vi "Sievert_auto_RLC.vi"() -> ()   [LabVIEW 2011]
uses:
  <vilib>/Utility/error.llb/DialogType.ctl
  <vilib>/DAQmx/write.llb/DAQmx Write (Digital Bool 1Line 1Point).vi
  <vilib>/DAQmx/create/channels.llb/DAQmx Create Channel (DO-Digital Output).vi
  <vilib>/DAQmx/miscellaneous.llb/DAQmx Fill In Error Info.vi
  <vilib>/Analysis/Matrix/Numeric/Conversions/Array To Matrix - RA.vi
  <vilib>/Analysis/Matrix/Numeric/Conversions/Matrix To Array - RM.vi
  <vilib>/Analysis/NI_AALPro.lvlib
  <vilib>/Analysis/Matrix/NI_Matrix.lvlib
  <vilib>/Analysis/NI_AALBase.lvlib
panel:
  out "MEASURE C [F ]":dbl
  out "Automatico 2":dynamicdata(graph)
  out "termopar K 2":dbl format="%.3g"
  out "termopar K":string
  out "output NTC":dbl
  out "termopar K":dbl format="%.3g"
  out "path RLC_mean":path
  out "estagio 5":i32
  out "FIM":bool=TRUE
  out "limpo":i32
  in  "N fit":i32=5
  in  "ATM wait":u32
  in  "SET":i32
  in  "time subarray":dbl[](array[numeric])
  out "P cinetica mean 2":dbl format="%0.2f"
  out "T cinetica mean 3":dbl format="%0.2f"
  out "Time cinetica":dbl format="%0.2f"
  in  "T subarray 3":dbl[](array[numeric])
  in  "P T  index 2":i32
  in  "P subarray 2":dbl[](array[numeric])
  in  "Numeric":dbl=4.0
  in  "T subarray 2":dbl[](array[numeric])
  out "T cinetica mean 2":dbl format="%0.2f"
  out "P cinetica mean":dbl format="%0.2f"
  in  "P subarray":dbl[](array[numeric])
  in  "P T  index":i32
  out "T string":string
  out "P string":string
  out "path 2_cinetica":path
  out "Polynomial Coefficients 2":dbl[](array[numeric])
  out "Polynomial Coefficients":dbl[](array[numeric])
  in  "Count SET":i32=-1
  out "Set atual":i32
  out "mean pressure":dbl format="%.4p"
  out "Set number":i32
  in  "Tab Control":enum32{"Manual", "Automatico", "RLC - CDH2"}(tab)
  out "T":bool
  out "ZPf2":bool
  out "Pf2":bool
  out "Pit":bool
  out "ZPit":bool
  out "Camara":dbl(slide) scale=0.0..59.5 scale format="%#_3g"
  in  "Save manual":bool
  in  "Open Button":bool
  out "String 2":string
  in  "ATM":bool
  in  "Câmara":bool
  in  "Vácuo":bool
  in  "Entrada Gás":bool
  in  "Manual Ctrl":bool
  in  "stop":bool
  out "P-manual":dynamicdata(graph)
  in  "Clear":bool
  out "path":path
  in  "Nota":string
  in  "Sample name":string
  in  "File name":string
  out "Linear Model Graph":dbl[][](graph)
  out "Linear Model Graph 2":dbl[][](graph)
  in  "N to fit":i32=60
  out "N":i32
  out "Vácuo":bool
  out "Atm":bool
  out "Câmara":bool
  out "String_cinetica":string
  out "Vol Ref":dbl(slide) scale=0.0..60.0 scale format="%#_4f"
  out "Entrada gás":bool
  in  "Guardar\nCinetica":bool
  out "p fit":dbl format="%#_4g"
  out "T fit":dbl format="%#_4g"
  in  "Open Button 2":bool
  out "x >= y?":bool
  in  "seconds":dbl
  out "Elapsed Time (sec)":dbl format="%.1f"
  out "bar/N":dbl format="%#_4p"
  in  "correção NTC":dbl
  out "mean H2 sensor (V)":dbl format="%#_4p"
  out "Boolean 3":bool
  out "String 3":string
  out "T 2":bool
  out "ZPit 2":bool
  out "Pit 2":bool
  out "Pf2 2":bool
  out "ZPf2 2":bool
  out "Camara 2":dbl(slide) scale=0.0..18.0 scale format="%#_3g"
  out "Vácuo 2":bool
  out "Atm 2":bool
  out "Câmara 2":bool
  out "Vol Ref 3":dbl(slide) scale=0.0..25.0 scale format="%#_4f"
  out "Entrada gás 2":bool
  in  "Auto Ctrl":bool
  in  "Play Button":bool
  out "time stamp":timestamp format="%<%.2X>T"
  out "Time (sec)":dbl format="%.1f"
  in  "clear":bool
  out "Automatico":dynamicdata(graph)
  out "Linear P":T1(graph)
  out "Linear T":T1(graph)
  out "Contador":i32
  in  "STOP (bar/s)":dbl format="%#_5p"
  out "P (bar/s)":dbl format="%#_5p"
  out "bar/s":dbl format="%#_4p"
  out "P fit":dbl format="%#_4g"
  out "T fit":dbl format="%#_4g"
  out "x = y?":bool
  out "teste slope":i32
  in  "Set P auto":dbl
  in  "Step P":dbl=2.0
  in  "P_max":dbl=2.0
  in  "P_max camara":dbl=2.0
  out "Carga":bool=TRUE
  out "Descarga":bool
  out "String":string
  in  "P_min descarga":dbl
  in  "Boolean":bool
  in  "Array":dbl[](array[numeric])
  out "Boolean 2":bool
  out "Desc SET":i32
  in  "ZPf2 time":dbl=24.0
  in  "Ciclos":dbl
  out "Efetuados":dbl
  in  "patamar milliseconds to wait":u32=500
  in  "N fit patamar":i32=100
  in  "Step ZPit":dbl
  out "Read ZPit":bool
  in  "Estagio auto":i32
  out "mean H2 sensor":dbl format="%#_4p"
  out "String 4":string
  in  "Combo Box":string(combo)
  in  "Refresh Button":bool
  in  "Close RLC 2":bool
  in  "RLC on/off":bool
  out "mean 16":dbl format="%.3p"
  out "mean 15":dbl format="%.3p"
  out "mean 14":dbl format="%.3p"
  out "mean 13":dbl format="%.3p"
  out "mean 12":dbl format="%.3p"
  out "mean 11":dbl format="%.3p"
  out "mean 10":dbl format="%.3p"
  out "mean 9":dbl format="%.3p"
  out "mean 8":dbl format="%.3p"
  out "mean 7":dbl format="%.3p"
  out "mean 6":dbl format="%.3p"
  out "mean 5":dbl format="%.3p"
  out "mean 4":dbl format="%.3p"
  out "mean 3":dbl format="%.3p"
  out "mean 2":dbl format="%.3p"
  out "mean":dbl format="%.3p"
  out "SET 2":dbl format="%#_3g"
  out "C-50-L":bool
  out "MEASURE B":dbl
  out "MEASURE A":dbl
  out "C-50-N":bool
  out "MEASURE B 2":dbl
  out "MEASURE A 2":dbl
  out "C-100-L":bool
  out "MEASURE B 3":dbl
  out "MEASURE A 3":dbl
  out "C-100-N":bool
  out "MEASURE B 4":dbl
  out "MEASURE A 4":dbl
  out "C-1K-L":bool
  out "MEASURE B 5":dbl
  out "MEASURE A 5":dbl
  out "C-1K-N":bool
  out "MEASURE B 6":dbl
  out "MEASURE A 6":dbl
  out "C-10K-L":bool
  out "MEASURE B 7":dbl
  out "MEASURE A 7":dbl
  out "C-10K-N":bool
  out "MEASURE B 8":dbl
  out "MEASURE A 8":dbl
  out "Z-50-L":bool
  out "MEASURE B 9":dbl
  out "MEASURE A 9":dbl
  out "Z-50-N":bool
  out "MEASURE B 10":dbl
  out "MEASURE A 10":dbl
  out "Z-100-L":bool
  out "MEASURE B 11":dbl
  out "MEASURE A 11":dbl
  out "Z-100-N":bool
  out "MEASURE B 12":dbl
  out "MEASURE A 12":dbl
  out "Z-1K-L":bool
  out "MEASURE B 13":dbl
  out "MEASURE A 13":dbl
  out "Z-1K-N":bool
  out "MEASURE B 14":dbl
  out "MEASURE A 14":dbl
  out "Z-10K-L":bool
  out "MEASURE B 15":dbl
  out "MEASURE A 15":dbl
  out "Z-10K-N":bool
  out "MEASURE B 16":dbl
  out "MEASURE A 16":dbl
  out "RLC300 - digimess":string
  in  "Time RLC":u32=5000
  in  "Ligar RLC":bool
  out "path RLC_completo":path
  out "Waveform Chart P 2":dbl[][](graph)
  out "Waveform Chart":dynamicdata(graph)
  in  "graph RLC":bool
  in  "Refresh Button 2":bool
  # "P vol ref"
  # "P Câmara"
  # "P vol ref"
  # "P Câmara"
  # "C ( F )"
  # "R ( Ohm )"
  # "Z ( Ohm )"
  # "Phase ( deg)"
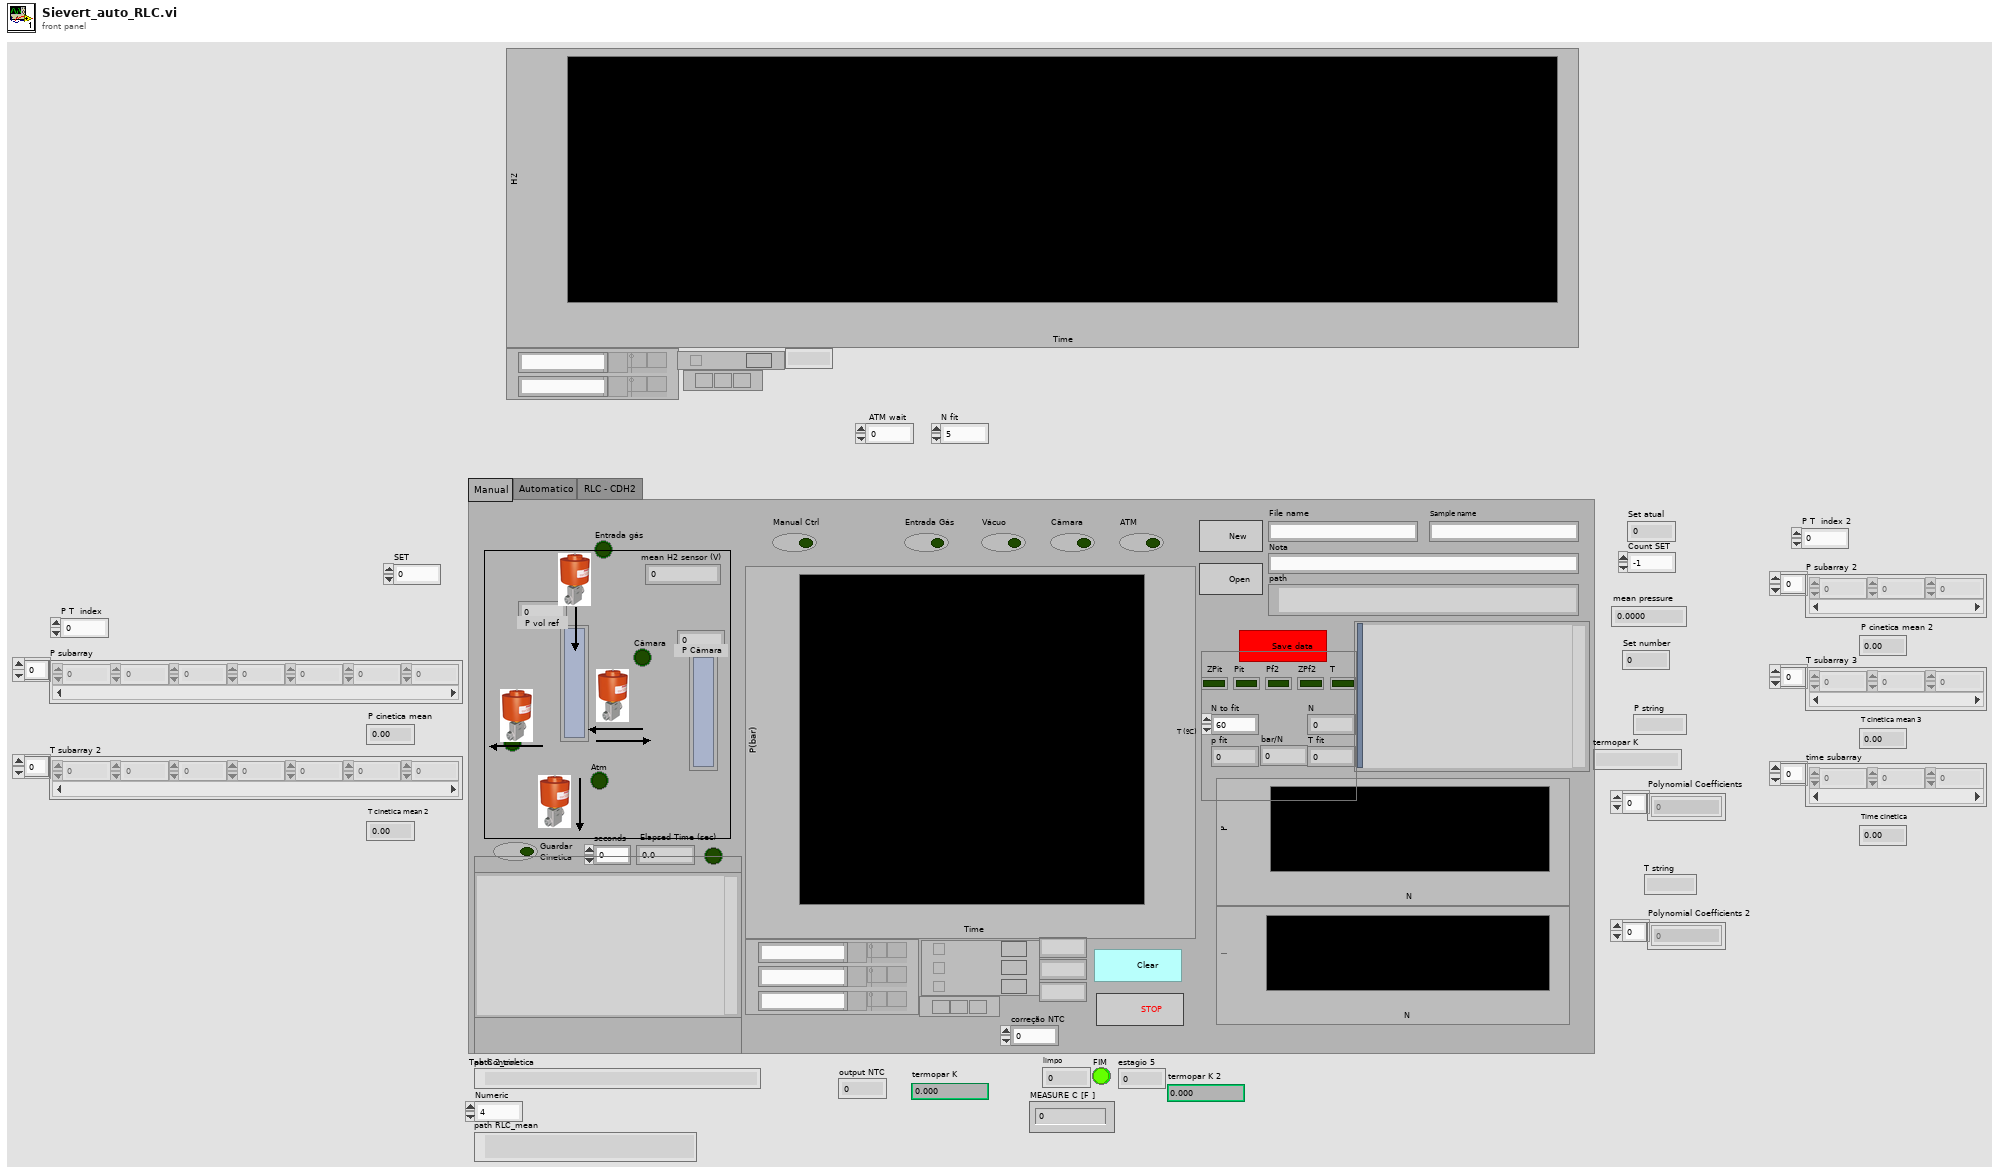
[diagram p1: front panel]
types:
  T1 = cluster{"Real 2D Array":dbl[], "Best Linear Fit":dbl[]}[]
  T2 = enum16{"open", "replace", "create", "open or create", "replace or create", "replace or create with confirmation"}
  T3 = typedef "NI_Matrix.lvlib/RealMatrix.ctl" = dbl[][]
  T4 = cluster{"Real 2D Array":dbl[], "Real 2D Array":dbl[]}
  T5 = typedef "DialogType.ctl" = u16
  T6 = cluster{"Real 2D Array":dbl[], "Best Linear Fit":dbl[]}
  T7 = cluster{"Real 2D Array":dbl[], "Best Polynomial Fit":dbl[]}
  T8 = cluster{"Real 2D Array":dbl[], "Best Polynomial Fit":dbl[]}[]
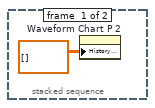
[diagram p5: hidden frame]
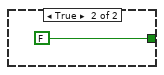
[diagram p10: hidden frame]
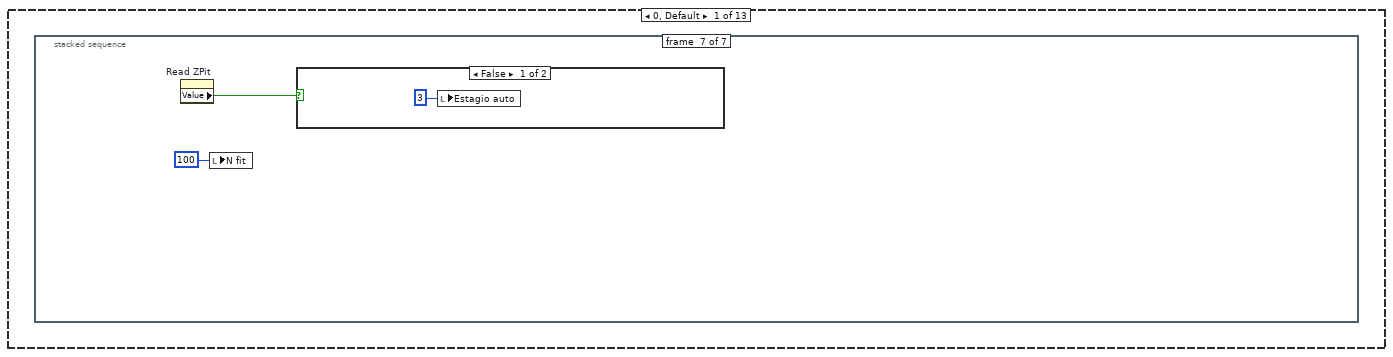
[diagram p13: hidden frame]
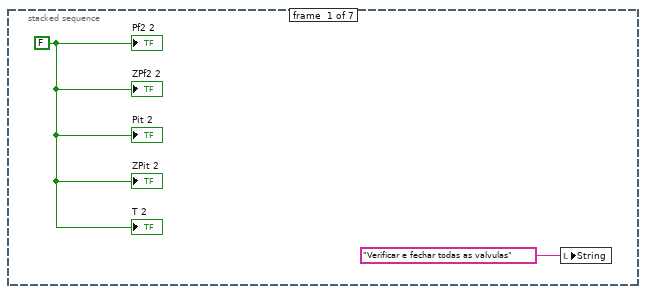
[diagram p14: hidden frame]
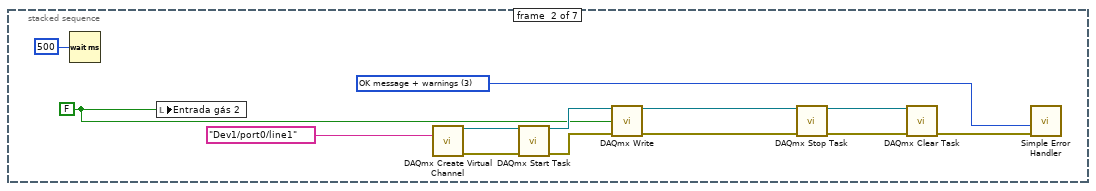
[diagram p15: hidden frame]
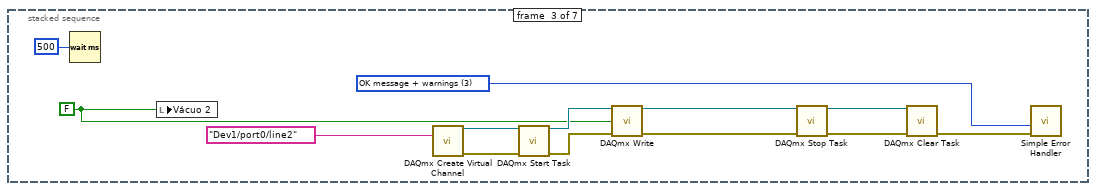
[diagram p16: hidden frame]
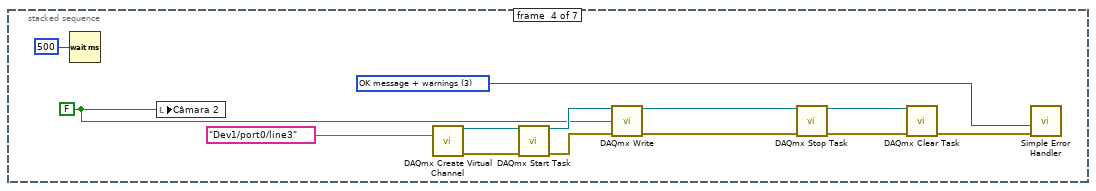
[diagram p17: hidden frame]
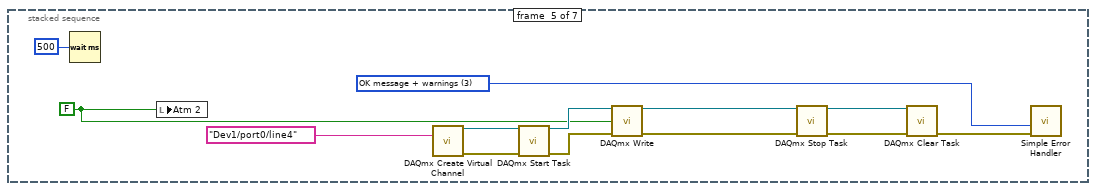
[diagram p18: hidden frame]
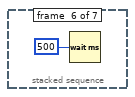
[diagram p19: hidden frame]
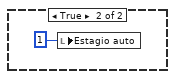
[diagram p20: hidden frame]
diagram:
  n1 = local write "N to fit"(5 ("Numeric")) -> ()
  n2 = local write "correção NTC"(0.5 ("correção NTC")) -> ()
  n3 = local write "Step ZPit"(5.0 ("Step ZPit")) -> ()
  n4 = local write "Time RLC"(u32 5 ("Time RLC")) -> ()
  n5 = local write "Ciclos"(0.0 ("Ciclos")) -> ()
  n6 = local write "Desc SET"(0 ("Desc SET")) -> ()
  n7 = local write "Efetuados"(0.0 ("Efetuados")) -> ()
  n8 = local write "estagio 5"(0 ("estagio 5")) -> ()
  n9 = local write "teste slope"(0 ("teste slope")) -> ()
  n10 = local write "SET"(0 ("SET auto")) -> ()
  n11 = local write "limpo"(0 ("limpo")) -> ()
  n12 = local write "N fit"(5 ("N fit")) -> ()
  n13 = local write "ATM wait"(u32 4 ("ATM wait")) -> ()
  n14 = local write "Estagio auto"(0 ("Estagio auto")) -> ()
  n15 = local write "P T  index"(0 ("index")) -> ()
  n16 = local write "seconds"(2.0 ("seconds")) -> ()
  n17 = local write "Read ZPit"(TRUE ("Read ZPit")) -> ()
  n18 = local write "Descarga"(FALSE ("Descarga")) -> ()
  n19 = local write "Carga"(TRUE ("Carga")) -> ()
  n20 = local write "FIM"(FALSE ("FIM")) -> ()
  n21 = local write "P_max"(50.0 ("P_max")) -> ()
  n22 = local write "P_max camara"(25.0 ("P_max camara")) -> ()
  n23 = local write "Set P auto"(0.5 ("Set P auto")) -> ()
  n24 = local write "P_min descarga"(0.025 ("P_min descarga")) -> ()
  n25 = local write "P subarray"(dbl[] [0.0, 1.0] ("subarray")) -> ()
  n26 = local write "T subarray 2"(dbl[] [0.0, 1.0] ("subarray")) -> ()
  n27 = local write "Combo Box"("rlc_read_cCN.py" ("Combo Box")) -> ()
  n28 = while {
    tunnel: path "C:/H2_Painel/painel_auto/RLC_CDH" ("Path") -> [w35]
    stop <- w47 stop-if-true
    n29 = property on="FIM" class="Bool (strict)"() -> ("Value"=w45:bool)  [unwired: 2 in, 2 out]
    n30 = property on="path" class="Path"() -> ("Value"=w42:path)  [unwired: 2 in, 2 out]
    n31 = case shown="True" "Ligar RLC" {
      tunnel: w35 -> [_ w222]
      frame False {
      }
      frame True {
        n32 = call "RLC_open.vi"("Path"=w222) -> ("String 2"=w223:string)  [unwired: 9 in, 1 out]
        n33 = local write "RLC300 - digimess"(w223) -> ()
      }
    }
    n34 = case shown="True" "Auto Ctrl" {
      tunnel: w35 -> [_ w228]
      tunnel: "RLC on/off" -> [_ w227]
      tunnel: [_ w226] -> w38
      frame False {
      }
      frame True {
        n35 = local write "P T  index 2"(0 ("P T  index")) -> ()
        n36 = for {
          N: "N fit" -> [w250]
          tunnel: w228 -> [w241]
          tunnel: w227 -> [w240]
          tunnel: [w239] -> w226
          i -> [w252]
          w256 = 0 ("polynomial order")
          w247 = 0 ("polynomial order")
          n37 = case shown="True" "clear" {
            frame False {
            }
            frame True {
              n38 = property on="Linear P" class="XYGraph (strict)"("Value"=T1 [] ("Linear P")) -> ()  [unwired: 2 in, 2 out]
              n39 = property on="Linear T" class="XYGraph (strict)"("Value"=T1 [] ("Linear T")) -> ()  [unwired: 2 in, 2 out]
              n40 = property on="Automatico" class="WFChart (strict)"("History Data"=dynamicdata[] []) -> ()  [unwired: 2 in, 2 out]
            }
          }
          n41 = property on="path 2_cinetica" class="Path"() -> ("Value"=w244:path)  [unwired: 2 in, 2 out]
          n42 = Increment(x=w252) -> (x+1=w251:i32)
          n43 = call "Read P T.vi"("correção NTC"="correção NTC") -> ("P Set 2 Output 2"=w277:dbl, "output NTC"=w238:dbl, "mean H2 sensor"=w234:dbl, "termopar K"=w237:dbl)  [unwired: 7 out]
          "termopar K 2" <- w237
          "mean H2 sensor" <- w234
          n44 = Equal?(x=w251, y=w250) -> (x = y?=w253:bool)
          "x = y?" <- w253
          n45 = Merge Signals(w234) -> (→"Automatico 2":dynamicdata)
          n46 = Multiply(x=w277, y=10.0) -> (x*y=w246:dbl)
          n47 = local write "Vol Ref 3"(w246) -> ()
          n48 = Merge Signals(w246, w238, w237) -> (→"Automatico":dynamicdata)
          n49 = call "Elapsed Time2"("Reset"=w253) -> ("Elapsed Time (s)"=w267:dbl)  [unwired: 11 in, 7 out]
          "Time (sec)" <- w267
          n50 = stacked-sequence {
            tunnel: w246 -> [w1588 _]
            tunnel: w238 -> [w1574 _]
            tunnel: [w1555 _] -> w265
            tunnel: [w1571 _] -> w264
            tunnel: w267 -> [w1558 _]
            tunnel: [w1556 _] -> w261
            tunnel: [w1554 _] -> w243
            tunnel: [w1553 _] -> w242
            frame #0 {
              w1557 = 2 ("y")
              n51 = property on="P subarray 2" class="Arr (strict)"() -> ("Value"=w1590:dbl[])  [unwired: 2 in, 2 out]
              n52 = property on="T subarray 3" class="Arr (strict)"() -> ("Value"=w1580:dbl[])  [unwired: 2 in, 2 out]
              n53 = property on="time subarray" class="Arr (strict)"() -> ("Value"=w1567:dbl[])  [unwired: 2 in, 2 out]
              n54 = property on="P T  index 2" class="DigNum (strict)"() -> ("Value"=w1559:i32)  [unwired: 2 in, 2 out]
              n55 = Replace Array Subset(array=w1567, new element=w1558, index=w1559) -> (w1560:dbl[])
              n56 = Replace Array Subset(array=w1590, new element=w1588, index=w1559) -> (w1573:dbl[])
              n57 = Replace Array Subset(array=w1580, new element=w1574, index=w1559) -> (w1572:dbl[])
              n58 = call-poly <vilib>:"Array To Matrix.vi"("Real 1D Array"=w1560) -> ("Real Matrix (Column Vector)"=w1570:T3)
              n59 = call-poly <vilib>:"Array To Matrix.vi"("Real 1D Array"=w1573) -> ("Real Matrix (Column Vector)"=w1593:T3)
              n60 = call-poly <vilib>:"Array To Matrix.vi"("Real 1D Array"=w1572) -> ("Real Matrix (Column Vector)"=w1583:T3)
              n61 = Matrix Size(0:w1570) -> (1:w1569:i32, 2:w1568:i32)
              n62 = Matrix Size(0:w1593) -> (1:w1592:i32, 2:w1591:i32)
              n63 = Matrix Size(0:w1583) -> (1:w1582:i32, 2:w1581:i32)
              n64 = Increment(x=w1569) -> (x+1=w1561:i32)
              n65 = Increment(x=w1592) -> (x+1=w1584:i32)
              n66 = Increment(x=w1582) -> (x+1=w1575:i32)
              n67 = Subtract(x=w1561, y=w1557) -> (x-y=w1562:i32)
              n68 = Subtract(x=w1584, y=w1557) -> (x-y=w1585:i32)
              n69 = Subtract(x=w1575, y=w1557) -> (x-y=w1576:i32)
              n70 = Resize Matrix(1:w1568, 2:w1561, 4:w1570) -> (0:w1566:T3)
              n71 = Resize Matrix(1:w1591, 2:w1584, 4:w1593) -> (0:w1589:T3)
              n72 = Resize Matrix(1:w1581, 2:w1575, 4:w1583) -> (0:w1579:T3)
              n73 = call-poly <vilib>:"Matrix To Array.vi"("Real Matrix"=w1566) -> ("Real 2D Array"=w1564:dbl[][])
              n74 = call-poly <vilib>:"Matrix To Array.vi"("Real Matrix"=w1589) -> ("Real 2D Array"=w1587:dbl[][])
              n75 = call-poly <vilib>:"Matrix To Array.vi"("Real Matrix"=w1579) -> ("Real 2D Array"=w1578:dbl[][])
              n76 = Reshape Array(w1564, w1561) -> (w1563:dbl[])
              n77 = Reshape Array(w1587, w1584) -> (w1586:dbl[])
              n78 = Reshape Array(w1578, w1575) -> (w1577:dbl[])
              n79 = local write "time subarray"(w1563) -> ()
              n80 = local write "P subarray 2"(w1586) -> ()
              n81 = local write "T subarray 3"(w1577) -> ()
              n82 = Reshape Array(w1563, w1562) -> (w1556:dbl[])
              n83 = Reshape Array(w1586, w1585) -> (w1555:dbl[])
              n84 = Reshape Array(w1577, w1576) -> (w1571:dbl[])
              n85 = call <vilib>:"Mean.vi"("X"=w1556) -> ("mean"=→"Time cinetica":dbl)  [unwired: 1 out]
              n86 = call <vilib>:"Mean.vi"("X"=w1555) -> ("mean"=w1554:dbl)  [unwired: 1 out]
              "P cinetica mean 2" <- w1554
              n87 = call <vilib>:"Mean.vi"("X"=w1571) -> ("mean"=w1553:dbl)  [unwired: 1 out]
              "T cinetica mean 3" <- w1553
            }
            frame #1 {
              n88 = property on="P T  index 2" class="DigNum (strict)"() -> ("Value"=w1595:i32)  [unwired: 2 in, 2 out]
              n89 = Increment(x=w1595) -> (x+1=w1594:i32)
              n90 = local write "P T  index 2"(w1594) -> ()
            }
          }
          n91 = To Time Stamp(1:w267) -> (0:→"time stamp":timestamp)
          n92 = call <vilib>:"Linear Fit.vi"("Y"=w264, "X"=w261) -> ("Best Linear Fit"=w273:dbl[])  [unwired: 9 in, 4 out]
          n93 = Bundle("Real 2D Array"=w261, "Real 2D Array"=w264) -> (w271:T4)  [unwired: 1 in]
          n94 = Bundle("Real 2D Array"=w261, "Real 2D Array"=w265) -> (w270:T4)  [unwired: 1 in]
          n95 = call <vilib>:"General Polynomial Fit.vi"("Y"=w264, "polynomial order"=w247, "X"=w261) -> ("Best Polynomial Fit"=w262:dbl[], "Polynomial Coefficients"=w257:dbl[])  [unwired: 9 in, 2 out]
          n96 = call <vilib>:"General Polynomial Fit.vi"("Y"=w265, "polynomial order"=w247, "X"=w261) -> ("Best Polynomial Fit"=w263:dbl[], "Polynomial Coefficients"=w258:dbl[])  [unwired: 9 in, 2 out]
          n97 = call <vilib>:"Linear Fit.vi"("Y"=w265, "X"=w261) -> ("Best Linear Fit"=w268:dbl[], "slope"=w248:dbl)  [unwired: 9 in, 3 out]
          "bar/s" <- w248
          n98 = property on="path" class="Path"() -> ("Value"=w245:path)  [unwired: 2 in, 2 out]
          n99 = case shown="True" "Play Button" {
            tunnel: w245 -> [_ w288]
            tunnel: w246 -> [_ w287]
            tunnel: w244 -> [_ w286]
            tunnel: w243 -> [_ w285]
            tunnel: w242 -> [_ w284]
            tunnel: w241 -> [_ w283]
            tunnel: w240 -> [_ w282]
            tunnel: [_ w281] -> w239
            tunnel: w237 -> [_ w280]
            frame False {
            }
            frame True {
              n100 = case shown="1" "Estagio auto" {
                tunnel: w288 -> [_ _ _ w380 _ _ w533 _ w682 _ _ w1394 w1463]
                tunnel: w287 -> [_ w354 _ _ w429 w480 _ _ _ w1312 _ _ _]
                tunnel: w286 -> [_ _ _ _ _ _ _ w572 _ _ _ _ _]
                tunnel: w285 -> [_ _ _ _ _ _ _ w571 _ _ _ _ _]
                tunnel: w284 -> [_ _ _ _ _ _ _ w570 _ _ _ _ _]
                tunnel: w283 -> [_ _ _ _ _ _ _ _ w660 _ _ _ _]
                tunnel: w282 -> [_ _ _ _ _ _ _ _ w677 _ _ _ _]
                tunnel: [_ _ _ _ _ _ _ _ w659 _ _ _ _] -> w281
                tunnel: w280 -> [_ _ _ _ _ _ _ _ _ _ _ w1389 _]
                frame 0, Default {
                  n101 = stacked-sequence {
                    frame #0 {
                      w290 = FALSE ("Pit")
                      n102 = local write "String"("Verificar e fechar todas as valvulas" ("String")) -> ()
                      "ZPf2 2" <- w290
                      "Pf2 2" <- w290
                      "Pit 2" <- w290
                      "ZPit 2" <- w290
                      "T 2" <- w290
                    }
                    frame #1 {
                      w293 = FALSE ("Boolean 4")
                      w298 = T5 3 items=["no dialog", "OK message", "continue or stop message", "OK message + warnings", "continue/stop + warnings"] ("type of dialog (OK msg:1)")
                      n103 = Wait (ms)(milliseconds to wait=u32 500) -> ()  [unwired: 1 out]
                      n104 = local write "Entrada gás 2"(w293) -> ()
                      n105 = call-poly <vilib>:"DAQmx Create Virtual Channel.vi"("lines"=tag "Dev1/port0/line1") -> ("task out"=w296:refnum<k21>, "error out"=w297:errorcluster)  [unwired: 13 in]
                      n106 = call <vilib>:"DAQmx Start Task.vi"("task/channels in"=w296, "error in"=w297) -> ("task out"=w299:refnum<k21>, "error out"=w300:errorcluster)  [unwired: 12 in]
                      n107 = call-poly <vilib>:"DAQmx Write.vi"("task/channels in"=w299, "data"=w293, "error in"=w300) -> ("task out"=w304:refnum<k21>, "error out"=w301:errorcluster)  [unwired: 10 in, 1 out]
                      n108 = call <vilib>:"DAQmx Stop Task.vi"("task/channels in"=w304, "error in"=w301) -> ("task out"=w303:refnum<k21>, "error out"=w302:errorcluster)  [unwired: 12 in]
                      n109 = call <vilib>:"DAQmx Clear Task.vi"("task in"=w303, "error in"=w302) -> ("error out"=w295:errorcluster)  [unwired: 13 in]
                      n110 = call <vilib>:"Simple Error Handler.vi"("type of dialog (OK msg:1)"=w298, "error in (no error)"=w295) -> ()  [unwired: 3 in, 5 out]
                    }
                    frame #2 {
                      w306 = FALSE ("Boolean 4")
                      w311 = T5 3 items=["no dialog", "OK message", "continue or stop message", "OK message + warnings", "continue/stop + warnings"] ("type of dialog (OK msg:1)")
                      n111 = Wait (ms)(milliseconds to wait=u32 500) -> ()  [unwired: 1 out]
                      n112 = local write "Vácuo 2"(w306) -> ()
                      n113 = call-poly <vilib>:"DAQmx Create Virtual Channel.vi"("lines"=tag "Dev1/port0/line2") -> ("task out"=w309:refnum<k21>, "error out"=w310:errorcluster)  [unwired: 13 in]
                      n114 = call <vilib>:"DAQmx Start Task.vi"("task/channels in"=w309, "error in"=w310) -> ("task out"=w312:refnum<k21>, "error out"=w313:errorcluster)  [unwired: 12 in]
                      n115 = call-poly <vilib>:"DAQmx Write.vi"("task/channels in"=w312, "data"=w306, "error in"=w313) -> ("task out"=w317:refnum<k21>, "error out"=w314:errorcluster)  [unwired: 10 in, 1 out]
                      n116 = call <vilib>:"DAQmx Stop Task.vi"("task/channels in"=w317, "error in"=w314) -> ("task out"=w316:refnum<k21>, "error out"=w315:errorcluster)  [unwired: 12 in]
                      n117 = call <vilib>:"DAQmx Clear Task.vi"("task in"=w316, "error in"=w315) -> ("error out"=w308:errorcluster)  [unwired: 13 in]
                      n118 = call <vilib>:"Simple Error Handler.vi"("type of dialog (OK msg:1)"=w311, "error in (no error)"=w308) -> ()  [unwired: 3 in, 5 out]
                    }
                    frame #3 {
                      w319 = FALSE ("Boolean 4")
                      w324 = T5 3 items=["no dialog", "OK message", "continue or stop message", "OK message + warnings", "continue/stop + warnings"] ("type of dialog (OK msg:1)")
                      n119 = Wait (ms)(milliseconds to wait=u32 500) -> ()  [unwired: 1 out]
                      n120 = local write "Câmara 2"(w319) -> ()
                      n121 = call-poly <vilib>:"DAQmx Create Virtual Channel.vi"("lines"=tag "Dev1/port0/line3") -> ("task out"=w322:refnum<k21>, "error out"=w323:errorcluster)  [unwired: 13 in]
                      n122 = call <vilib>:"DAQmx Start Task.vi"("task/channels in"=w322, "error in"=w323) -> ("task out"=w325:refnum<k21>, "error out"=w326:errorcluster)  [unwired: 12 in]
                      n123 = call-poly <vilib>:"DAQmx Write.vi"("task/channels in"=w325, "data"=w319, "error in"=w326) -> ("task out"=w330:refnum<k21>, "error out"=w327:errorcluster)  [unwired: 10 in, 1 out]
                      n124 = call <vilib>:"DAQmx Stop Task.vi"("task/channels in"=w330, "error in"=w327) -> ("task out"=w329:refnum<k21>, "error out"=w328:errorcluster)  [unwired: 12 in]
                      n125 = call <vilib>:"DAQmx Clear Task.vi"("task in"=w329, "error in"=w328) -> ("error out"=w321:errorcluster)  [unwired: 13 in]
                      n126 = call <vilib>:"Simple Error Handler.vi"("type of dialog (OK msg:1)"=w324, "error in (no error)"=w321) -> ()  [unwired: 3 in, 5 out]
                    }
                    frame #4 {
                      w332 = FALSE ("Boolean 4")
                      w337 = T5 3 items=["no dialog", "OK message", "continue or stop message", "OK message + warnings", "continue/stop + warnings"] ("type of dialog (OK msg:1)")
                      n127 = Wait (ms)(milliseconds to wait=u32 500) -> ()  [unwired: 1 out]
                      n128 = local write "Atm 2"(w332) -> ()
                      n129 = call-poly <vilib>:"DAQmx Create Virtual Channel.vi"("lines"=tag "Dev1/port0/line4") -> ("task out"=w335:refnum<k21>, "error out"=w336:errorcluster)  [unwired: 13 in]
                      n130 = call <vilib>:"DAQmx Start Task.vi"("task/channels in"=w335, "error in"=w336) -> ("task out"=w338:refnum<k21>, "error out"=w339:errorcluster)  [unwired: 12 in]
                      n131 = call-poly <vilib>:"DAQmx Write.vi"("task/channels in"=w338, "data"=w332, "error in"=w339) -> ("task out"=w343:refnum<k21>, "error out"=w340:errorcluster)  [unwired: 10 in, 1 out]
                      n132 = call <vilib>:"DAQmx Stop Task.vi"("task/channels in"=w343, "error in"=w340) -> ("task out"=w342:refnum<k21>, "error out"=w341:errorcluster)  [unwired: 12 in]
                      n133 = call <vilib>:"DAQmx Clear Task.vi"("task in"=w342, "error in"=w341) -> ("error out"=w334:errorcluster)  [unwired: 13 in]
                      n134 = call <vilib>:"Simple Error Handler.vi"("type of dialog (OK msg:1)"=w337, "error in (no error)"=w334) -> ()  [unwired: 3 in, 5 out]
                    }
                    frame #5 {
                      n135 = Wait (ms)(milliseconds to wait=u32 500) -> ()  [unwired: 1 out]
                    }
                    frame #6 {
                      n136 = property on="Read ZPit" class="Bool (strict)"() -> ("Value"=w346:bool)  [unwired: 2 in, 2 out]
                      n137 = local write "N fit"(100 ("N fit")) -> ()
                      n138 = case shown="False" w346 {
                        frame False {
                          n139 = local write "Estagio auto"(3 ("Estagio auto")) -> ()
                        }
                        frame True {
                          n140 = local write "Estagio auto"(1 ("Estagio auto")) -> ()
                        }
                      }
                    }
                  }
                }
                frame 1 {
                  n141 = Greater?(x=w354, y=1.0) -> (0:w353:bool)
                  n142 = case shown="True" w353 {
                    tunnel: [FALSE ("Boolean") TRUE ("Boolean")] -> w350
                    frame False {
                      w366 = TRUE ("Boolean")
                      n143 = local write "Vácuo 2"(w366) -> ()
                      n144 = call "Controle_vacuo.vi"("time (s) to wait vacuo"=u32 5, "Boolean"=w366) -> ("Vacuo"=w367:bool)  [unwired: 9 in]
                      n145 = local write "Vácuo 2"(w367) -> ()
                      n146 = local write "String"("Limpar volume referencia" ("String")) -> ()
                    }
                    frame True {
                      n147 = call "Controle_ATM.vi"("seconds to wait"="ATM wait") -> ("String 2"=w371:string, "Atm"=w370:bool)  [unwired: 9 in]
                      n148 = local write "Atm 2"(w370) -> ()
                      n149 = local write "String"(w371) -> ()
                    }
                  }
                  n150 = for {
                    N: 1 -> [_]
                    tunnel: [w356] -> w351
                    tunnel: w350 -> [w356]
                    n151 = Wait (ms)(milliseconds to wait=u32 500 ("x")) -> ()  [unwired: 1 out]
                  }
                  n152 = case shown="True" w351 {
                    frame False {
                      n153 = local write "Estagio auto"(2 ("Estagio auto")) -> ()
                    }
                    frame True {
                      w361 = TRUE ("Boolean")
                      n154 = local write "Estagio auto"(2 ("Estagio auto")) -> ()
                      n155 = local write "Vácuo 2"(w361) -> ()
                      n156 = call "Controle_vacuo.vi"("time (s) to wait vacuo"=u32 5, "Boolean"=w361) -> ("Vacuo"=w362:bool)  [unwired: 9 in]
                      n157 = local write "Vácuo 2"(w362) -> ()
                      n158 = local write "String"("Limpar volume referencia" ("String")) -> ()
                    }
                  }
                }
                frame 2 {
                  n159 = property on="Contador" class="DigNum (strict)"() -> ("Value"=w375:i32)  [unwired: 2 in, 2 out]
                  n160 = local write "String"("Ler ZPit" ("String")) -> ()
                  n161 = Increment(x=w375) -> (x+1=w374:i32)
                  n162 = Equal?(x=w374, y=100) -> (x = y?=w372:bool)
                  n163 = case shown="True" w372 {
                    frame False {
                    }
                    frame True {
                      n164 = local write "Estagio auto"(3 ("Estagio auto")) -> ()
                    }
                  }
                }
                frame 3 {
                  w383 = "\t"
                  n165 = property on="SET" class="DigNum (strict)"() -> ("Value"=w379:i32)  [unwired: 2 in, 2 out]
                  n166 = property on="Read ZPit" class="Bool (strict)"() -> ("Value"=w378:bool)  [unwired: 2 in, 2 out]
                  n167 = case shown="False" w378 {
                    tunnel: ["  ==>" w390] -> w384
                    frame False {
                    }
                    frame True {
                      n168 = property on="P fit" class="DigNum (strict)"() -> ("Value"=w389:dbl)  [unwired: 2 in, 2 out]
                      n169 = Number To Fractional String(number=w389, precision (6)=i16 3) -> (F-format string=w390:string)  [unwired: 2 in]
                    }
                  }
                  n170 = Number To Decimal String(number=w379) -> (decimal integer string=w382:string)  [unwired: 1 in]
                  n171 = Concatenate Strings(w382, w383, w384, w383) -> (w381:string)
                  n172 = flat-sequence {
                    tunnel: [w394] -> w386
                    tunnel: [w393] -> w385
                    tunnel: w381 -> [w392]
                    tunnel: w380 -> [w391]
                    tunnel: w386 -> [w410]
                    tunnel: w385 -> [w409]
                    frame #0 {
                      n173 = Open/Create/Replace File(file path (use dialog)=w391, operation (0:open)=T2."open") -> (refnum out=w400:refnum<file>, error out=w401:errorcluster)  [unwired: 2 in, 3 out]
                      n174 = Set File Position(refnum=w400, from (0:start)=enum16{"start", "end", "current"}."end", error in=w401) -> (refnum out=w398:refnum<file>, error out=w397:errorcluster)  [unwired: 1 in]
                      n175 = Write to Text File(file (use dialog)=w398, text=w392, error in=w397) -> (refnum out=w402:refnum<file>, error out=w403:errorcluster)  [unwired: 2 out]
                      n176 = Close File(refnum=w402, error in=w403) -> (path=w394:path, error out=w395:errorcluster)
                      n177 = call <vilib>:"Simple Error Handler.vi"("error in (no error)"=w395) -> ("error out"=w393:errorcluster)  [unwired: 1 in, 7 out]
                    }
                    frame #1 {
                      w404 = 0 ("limpo")
                      n178 = local write "Estagio auto"(4 ("Estagio auto")) -> ()
                      n179 = local write "ZPit 2"(TRUE ("ZPit")) -> ()
                      n180 = Wait (ms)(milliseconds to wait=u32 500) -> ()  [unwired: 1 out]
                      n181 = local write "limpo"(w404) -> ()
                      n182 = Read from Text File(file (use dialog)=w410, count=-1 ("Count  3"), error in=w409) -> (refnum out=w411:refnum<file>, text=w415:string, error out=w412:errorcluster)  [unwired: 1 in, 1 out]
                      n183 = local write "String 3"(w415) -> ()
                      n184 = local write "estagio 5"(w404) -> ()
                      n185 = Close File(refnum=w411, error in=w412) -> (error out=w413:errorcluster)  [unwired: 1 out]
                      n186 = call <vilib>:"Simple Error Handler.vi"("error in (no error)"=w413) -> ()  [unwired: 1 in, 8 out]
                      n187 = local write "String"("abrir valvula entrada gas" ("String")) -> ()
                    }
                    frame #2 {
                      w416 = T5 3 items=["no dialog", "OK message", "continue or stop message", "OK message + warnings", "continue/stop + warnings"] ("type of dialog (OK msg:1)")
                      w422 = TRUE ("Boolean 4")
                      n188 = local write "Entrada gás 2"(w422) -> ()
                      n189 = call-poly <vilib>:"DAQmx Create Virtual Channel.vi"("lines"=tag "Dev1/port0/line1") -> ("task out"=w424:refnum<k21>, "error out"=w425:errorcluster)  [unwired: 13 in]
                      n190 = call <vilib>:"DAQmx Start Task.vi"("task/channels in"=w424, "error in"=w425) -> ("task out"=w426:refnum<k21>, "error out"=w427:errorcluster)  [unwired: 12 in]
                      n191 = call-poly <vilib>:"DAQmx Write.vi"("task/channels in"=w426, "data"=w422, "error in"=w427) -> ("task out"=w419:refnum<k21>, "error out"=w418:errorcluster)  [unwired: 10 in, 1 out]
                      n192 = call <vilib>:"DAQmx Stop Task.vi"("task/channels in"=w419, "error in"=w418) -> ("task out"=w420:refnum<k21>, "error out"=w421:errorcluster)  [unwired: 12 in]
                      n193 = call <vilib>:"DAQmx Clear Task.vi"("task in"=w420, "error in"=w421) -> ("error out"=w417:errorcluster)  [unwired: 13 in]
                      n194 = call <vilib>:"Simple Error Handler.vi"("type of dialog (OK msg:1)"=w416, "error in (no error)"=w417) -> ()  [unwired: 3 in, 5 out]
                    }
                  }
                }
                frame 4 {
                  n195 = Greater Or Equal?(x=w429, y="Set P auto") -> (x >= y?=w430:bool)
                  n196 = case shown="True" w430 {
                    tunnel: "Set P auto" -> [_ w445]
                    frame False {
                      w438 = T5 3 items=["no dialog", "OK message", "continue or stop message", "OK message + warnings", "continue/stop + warnings"] ("type of dialog (OK msg:1)")
                      w444 = TRUE ("data")
                      n197 = local write "Estagio auto"(5 ("Estagio auto")) -> ()
                      n198 = Wait (ms)(milliseconds to wait=u32 500) -> ()  [unwired: 1 out]
                      n199 = local write "Entrada gás 2"(w444) -> ()
                      n200 = call-poly <vilib>:"DAQmx Create Virtual Channel.vi"("lines"=tag "Dev1/port0/line1") -> ("task out"=w435:refnum<k21>, "error out"=w434:errorcluster)  [unwired: 13 in]
                      n201 = call <vilib>:"DAQmx Start Task.vi"("task/channels in"=w435, "error in"=w434) -> ("task out"=w433:refnum<k21>, "error out"=w432:errorcluster)  [unwired: 12 in]
                      n202 = call-poly <vilib>:"DAQmx Write.vi"("task/channels in"=w433, "data"=w444, "error in"=w432) -> ("task out"=w441:refnum<k21>, "error out"=w440:errorcluster)  [unwired: 10 in, 1 out]
                      n203 = call <vilib>:"DAQmx Stop Task.vi"("task/channels in"=w441, "error in"=w440) -> ("task out"=w443:refnum<k21>, "error out"=w442:errorcluster)  [unwired: 12 in]
                      n204 = call <vilib>:"DAQmx Clear Task.vi"("task in"=w443, "error in"=w442) -> ("error out"=w439:errorcluster)  [unwired: 13 in]
                      n205 = call <vilib>:"Simple Error Handler.vi"("type of dialog (OK msg:1)"=w438, "error in (no error)"=w439) -> ()  [unwired: 3 in, 5 out]
                    }
                    frame True {
                      n206 = flat-sequence {
                        tunnel: [w448] -> w446
                        tunnel: w445 -> [w448]
                        tunnel: [w463] -> w447
                        tunnel: w446 -> [w462]
                        tunnel: w447 -> [w477]
                        frame #0 {
                          w454 = T5 3 items=["no dialog", "OK message", "continue or stop message", "OK message + warnings", "continue/stop + warnings"] ("type of dialog (OK msg:1)")
                          w461 = FALSE ("data")
                          n207 = Wait (ms)(milliseconds to wait=u32 500) -> ()  [unwired: 1 out]
                          n208 = local write "Entrada gás 2"(w461) -> ()
                          n209 = call-poly <vilib>:"DAQmx Create Virtual Channel.vi"("lines"=tag "Dev1/port0/line1") -> ("task out"=w452:refnum<k21>, "error out"=w453:errorcluster)  [unwired: 13 in]
                          n210 = call <vilib>:"DAQmx Start Task.vi"("task/channels in"=w452, "error in"=w453) -> ("task out"=w450:refnum<k21>, "error out"=w449:errorcluster)  [unwired: 12 in]
                          n211 = call-poly <vilib>:"DAQmx Write.vi"("task/channels in"=w450, "data"=w461, "error in"=w449) -> ("task out"=w458:refnum<k21>, "error out"=w457:errorcluster)  [unwired: 10 in, 1 out]
                          n212 = call <vilib>:"DAQmx Stop Task.vi"("task/channels in"=w458, "error in"=w457) -> ("task out"=w460:refnum<k21>, "error out"=w459:errorcluster)  [unwired: 12 in]
                          n213 = call <vilib>:"DAQmx Clear Task.vi"("task in"=w460, "error in"=w459) -> ("error out"=w455:errorcluster)  [unwired: 13 in]
                          n214 = call <vilib>:"Simple Error Handler.vi"("type of dialog (OK msg:1)"=w454, "error in (no error)"=w455) -> ()  [unwired: 3 in, 5 out]
                        }
                        frame #1 {
                          n215 = stacked-sequence {
                            tunnel: [_ _ _ w474] -> w463
                            tunnel: w462 -> [_ _ w467 _]
                            frame #0 {
                              n216 = call "Controle_ATM.vi"("seconds to wait"=2.0) -> ("Atm"=w465:bool)  [unwired: 9 in, 1 out]
                              n217 = local write "Atm 2"(w465) -> ()
                            }
                            frame #1 {
                              n218 = Wait (ms)(milliseconds to wait=u32 1000) -> ()  [unwired: 1 out]
                            }
                            frame #2 {
                              n219 = Less Or Equal?(x=w467, y=1.5) -> (x <= y?=w469:bool)
                              n220 = case shown="True" w469 {
                                frame False {
                                n221 = call "Controle_ATM.vi"("seconds to wait"=2.0) -> ()  [unwired: 9 in, 2 out]
                                }
                                frame True {
                                w472 = TRUE ("Vácuo")
                                n222 = local write "Vácuo 2"(w472) -> ()
                                n223 = call "Controle_vacuo.vi"("time (s) to wait vacuo"=3.0, "Boolean"=w472) -> ("Vacuo"=w473:bool)  [unwired: 9 in]
                                n224 = local write "Vácuo 2"(w473) -> ()
                                }
                              }
                            }
                            frame #3 {
                              n225 = property on="limpo" class="DigNum (strict)"() -> ("Value"=w475:i32)  [unwired: 2 in, 2 out]
                              n226 = Wait (ms)(milliseconds to wait=u32 1000) -> ()  [unwired: 1 out]
                              n227 = Increment(x=w475) -> (x+1=w474:i32)
                            }
                          }
                        }
                        frame #2 {
                          "limpo" <- w477
                        }
                      }
                    }
                  }
                }
                frame 5 {
                  n228 = property on="Set P auto" class="DigNum (strict)"() -> ("Value"=w479:dbl)  [unwired: 2 in, 2 out]
                  n229 = Greater Or Equal?(x=w480, y=w479) -> (x >= y?=w478:bool)
                  n230 = case shown="False" w478 {
                    selector: w478 -> [_ w502]
                    frame False {
                      n231 = flat-sequence {
                        tunnel: [w482] -> w481
                        tunnel: w481 -> [w498]
                        frame #0 {
                          w485 = T5 3 items=["no dialog", "OK message", "continue or stop message", "OK message + warnings", "continue/stop + warnings"] ("type of dialog (OK msg:1)")
                          w495 = TRUE ("Boolean 4")
                          n232 = property on="estagio 5" class="DigNum (strict)"() -> ("Value"=w483:i32)  [unwired: 2 in, 2 out]
                          n233 = local write "Entrada gás 2"(w495) -> ()
                          n234 = Increment(x=w483) -> (x+1=w482:i32)
                          n235 = call-poly <vilib>:"DAQmx Create Virtual Channel.vi"("lines"=tag "Dev1/port0/line1") -> ("task out"=w489:refnum<k21>, "error out"=w488:errorcluster)  [unwired: 13 in]
                          n236 = call <vilib>:"DAQmx Start Task.vi"("task/channels in"=w489, "error in"=w488) -> ("task out"=w487:refnum<k21>, "error out"=w486:errorcluster)  [unwired: 12 in]
                          n237 = call-poly <vilib>:"DAQmx Write.vi"("task/channels in"=w487, "data"=w495, "error in"=w486) -> ("task out"=w492:refnum<k21>, "error out"=w491:errorcluster)  [unwired: 10 in, 1 out]
                          n238 = call <vilib>:"DAQmx Stop Task.vi"("task/channels in"=w492, "error in"=w491) -> ("task out"=w493:refnum<k21>, "error out"=w494:errorcluster)  [unwired: 12 in]
                          n239 = call <vilib>:"DAQmx Clear Task.vi"("task in"=w493, "error in"=w494) -> ("error out"=w484:errorcluster)  [unwired: 13 in]
                          n240 = call <vilib>:"Simple Error Handler.vi"("type of dialog (OK msg:1)"=w485, "error in (no error)"=w484) -> ()  [unwired: 3 in, 5 out]
                        }
                        frame #1 {
                          n241 = Less?(x=w498, y=6) -> (x < y?=w496:bool)
                          n242 = case shown="False" w496 {
                            frame False {
                              n243 = local write "Estagio auto"(5 ("Estagio auto")) -> ()
                            }
                            frame True {
                              n244 = local write "Estagio auto"(4 ("Estagio auto")) -> ()
                            }
                          }
                          "estagio 5" <- w498
                        }
                      }
                    }
                    frame True {
                      n245 = flat-sequence {
                        tunnel: w502 -> [w503]
                        tunnel: [w503] -> w501
                        tunnel: w501 -> [w519]
                        frame #0 {
                          w504 = FALSE ("Boolean 4")
                          w509 = T5 3 items=["no dialog", "OK message", "continue or stop message", "OK message + warnings", "continue/stop + warnings"] ("type of dialog (OK msg:1)")
                          n246 = local write "Entrada gás 2"(w504) -> ()
                          n247 = call-poly <vilib>:"DAQmx Create Virtual Channel.vi"("lines"=tag "Dev1/port0/line1") -> ("task out"=w507:refnum<k21>, "error out"=w508:errorcluster)  [unwired: 13 in]
                          n248 = call <vilib>:"DAQmx Start Task.vi"("task/channels in"=w507, "error in"=w508) -> ("task out"=w510:refnum<k21>, "error out"=w511:errorcluster)  [unwired: 12 in]
                          n249 = call-poly <vilib>:"DAQmx Write.vi"("task/channels in"=w510, "data"=w504, "error in"=w511) -> ("task out"=w515:refnum<k21>, "error out"=w512:errorcluster)  [unwired: 10 in, 1 out]
                          n250 = call <vilib>:"DAQmx Stop Task.vi"("task/channels in"=w515, "error in"=w512) -> ("task out"=w514:refnum<k21>, "error out"=w513:errorcluster)  [unwired: 12 in]
                          n251 = call <vilib>:"DAQmx Clear Task.vi"("task in"=w514, "error in"=w513) -> ("error out"=w506:errorcluster)  [unwired: 13 in]
                          n252 = call <vilib>:"Simple Error Handler.vi"("type of dialog (OK msg:1)"=w509, "error in (no error)"=w506) -> ()  [unwired: 3 in, 5 out]
                        }
                        frame #1 {
                          n253 = property on="estagio 5" class="DigNum (strict)"() -> ("Value"=w517:i32)  [unwired: 2 in, 2 out]
                          n254 = Greater?(x=w517, y=5) -> (0:w520:bool)
                          n255 = And(x=w519, y=w520) -> (x .and. y?=w518:bool)
                          n256 = case shown="False" w518 {
                            frame False {
                              n257 = local write "Estagio auto"(4 ("Estagio auto")) -> ()
                              n258 = Wait (ms)(milliseconds to wait=u32 500) -> ()  [unwired: 1 out]
                            }
                            frame True {
                              n259 = property on="Contador" class="DigNum (strict)"() -> ("Value"=w523:i32)  [unwired: 2 in, 2 out]
                              n260 = local write "String"("Ler Pit" ("String")) -> ()
                              n261 = Increment(x=w523) -> (x+1=w526:i32)
                              n262 = Equal?(x=w526, y=100) -> (x = y?=w524:bool)
                              n263 = case shown="True" w524 {
                                frame False {
                                }
                                frame True {
                                n264 = local write "Estagio auto"(6 ("Estagio auto")) -> ()
                                }
                              }
                            }
                          }
                        }
                      }
                    }
                  }
                }
                frame 6 {
                  n265 = property on="Contador" class="DigNum (strict)"() -> ("Value"=w529:i32)  [unwired: 2 in, 2 out]
                  n266 = Increment(x=w529) -> (x+1=w532:i32)
                  n267 = Equal?(x=w532, y=100) -> (x = y?=w530:bool)
                  n268 = case shown="True" w530 {
                    tunnel: w533 -> [_ w534]
                    frame False {
                    }
                    frame True {
                      n269 = property on="P fit" class="DigNum (strict)"() -> ("Value"=w535:dbl)  [unwired: 2 in, 2 out]
                      n270 = Number To Fractional String(number=w535, precision (6)=i16 3) -> (F-format string=w539:string)  [unwired: 2 in]
                      n271 = Concatenate Strings(w539, "\t") -> (w537:string)
                      n272 = flat-sequence {
                        tunnel: [w545] -> w541
                        tunnel: [w544] -> w540
                        tunnel: w537 -> [w543]
                        tunnel: w534 -> [w542]
                        tunnel: w541 -> [w561]
                        tunnel: w540 -> [w560]
                        frame #0 {
                          n273 = Open/Create/Replace File(file path (use dialog)=w542, operation (0:open)=T2."open") -> (refnum out=w551:refnum<file>, error out=w552:errorcluster)  [unwired: 2 in, 3 out]
                          n274 = Set File Position(refnum=w551, from (0:start)=enum16{"start", "end", "current"}."end", error in=w552) -> (refnum out=w549:refnum<file>, error out=w548:errorcluster)  [unwired: 1 in]
                          n275 = Write to Text File(file (use dialog)=w549, text=w543, error in=w548) -> (refnum out=w553:refnum<file>, error out=w554:errorcluster)  [unwired: 2 out]
                          n276 = Close File(refnum=w553, error in=w554) -> (path=w545:path, error out=w546:errorcluster)
                          n277 = call <vilib>:"Simple Error Handler.vi"("error in (no error)"=w546) -> ("error out"=w544:errorcluster)  [unwired: 1 in, 7 out]
                        }
                        frame #1 {
                          n278 = local write "Estagio auto"(7 ("Estagio auto")) -> ()
                          n279 = local write "teste slope"(0 ("teste slope")) -> ()
                          n280 = local write "Pit 2"(TRUE ("ZPit")) -> ()
                          n281 = Wait (ms)(milliseconds to wait=u32 500) -> ()  [unwired: 1 out]
                          n282 = Read from Text File(file (use dialog)=w561, count=-1 ("Count  3"), error in=w560) -> (refnum out=w562:refnum<file>, text=w566:string, error out=w563:errorcluster)  [unwired: 1 in, 1 out]
                          n283 = local write "String 3"(w566) -> ()
                          n284 = Close File(refnum=w562, error in=w563) -> (error out=w564:errorcluster)  [unwired: 1 out]
                          n285 = call <vilib>:"Simple Error Handler.vi"("error in (no error)"=w564) -> ()  [unwired: 1 in, 8 out]
                          n286 = local write "String"("abrir valvula entrada camara" ("String")) -> ()
                        }
                      }
                    }
                  }
                }
                frame 7 {
                  n287 = flat-sequence {
                    tunnel: w570 -> [w574]
                    tunnel: w571 -> [w575]
                    tunnel: w572 -> [w576]
                    tunnel: [w576] -> w569
                    tunnel: [w575] -> w568
                    tunnel: [w574] -> w567
                    tunnel: w569 -> [w580]
                    tunnel: w568 -> [w579]
                    tunnel: w567 -> [w578]
                    frame #0 {
                      n288 = local write "N fit"("N fit patamar") -> ()
                    }
                    frame #1 {
                      n289 = flat-sequence {
                        tunnel: w580 -> [w592]
                        tunnel: w579 -> [w591]
                        tunnel: w578 -> [w590]
                        frame #0 {
                          w605 = "\t"
                          w611 = i16 4 ("precision (6)")
                          n290 = Number To Fractional String(number=w591, precision (6)=w611) -> (F-format string=w606:string)  [unwired: 2 in]
                          n291 = Number To Fractional String(number=w590, precision (6)=w611) -> (F-format string=w604:string)  [unwired: 2 in]
                          n292 = Open/Create/Replace File(file path (use dialog)=w592, operation (0:open)=T2."open") -> (refnum out=w600:refnum<file>, error out=w593:errorcluster)  [unwired: 2 in, 3 out]
                          n293 = Get Date/Time String(date format (0)=enum16{"short", "long", "abbreviated"}."short", want seconds? (F)=TRUE) -> (date string=w608:string, time string=w607:string)  [unwired: 1 in]
                          n294 = Set File Position(refnum=w600, from (0:start)=enum16{"start", "end", "current"}."end", error in=w593) -> (refnum out=w598:refnum<file>, error out=w597:errorcluster)  [unwired: 1 in]
                          n295 = Concatenate Strings(w608, w605, w607, w605, w606, w605, w604, "\r\n") -> (w594:string)
                          n296 = Write to Text File(file (use dialog)=w598, text=w594, error in=w597) -> (refnum out=w601:refnum<file>, error out=w602:errorcluster)  [unwired: 2 out]
                          n297 = Close File(refnum=w601, error in=w602) -> (error out=w595:errorcluster)  [unwired: 1 out]
                          n298 = call <vilib>:"Simple Error Handler.vi"("error in (no error)"=w595) -> ()  [unwired: 1 in, 8 out]
                        }
                      }
                      n299 = property on="Contador" class="DigNum (strict)"() -> ("Value"=w588:i32)  [unwired: 2 in, 2 out]
                      n300 = Increment(x=w588) -> (x+1=w587:i32)
                      n301 = property on="N fit patamar" class="DigNum (strict)"() -> ("Value"=w577:i32)  [unwired: 2 in, 2 out]
                      n302 = Equal?(x=w587, y=w577) -> (x = y?=w589:bool)
                      n303 = case shown="True" w589 {
                        tunnel: [FALSE w616] -> w586
                        tunnel: [_ w615] -> w585
                        frame False {
                        }
                        frame True {
                          n304 = property on="P (bar/s)" class="DigNum (strict)"() -> ("Value"=w618:dbl)  [unwired: 2 in, 2 out]
                          n305 = Absolute Value(x=w618) -> (abs(x)=w617:dbl)
                          n306 = Less Or Equal?(x=w617, y="STOP (bar/s)") -> (x <= y?=w616:bool)
                          n307 = case shown="True" w616 {
                            tunnel: [_ w620] -> w615
                            frame False {
                            }
                            frame True {
                              n308 = property on="teste slope" class="DigNum (strict)"() -> ("Value"=w621:i32)  [unwired: 2 in, 2 out]
                              n309 = local write "Estagio auto"(7 ("Estagio auto")) -> ()
                              n310 = Increment(x=w621) -> (x+1=w620:i32)
                              "teste slope" <- w620
                            }
                          }
                        }
                      }
                      n311 = Greater Or Equal?(x=w585, y=5) -> (x >= y?=w583:bool)
                      n312 = And(x=w589, y=w583) -> (x .and. y?=w582:bool)
                      n313 = case shown="True" w582 {
                        frame False {
                        }
                        frame True {
                          n314 = flat-sequence {
                            frame #0 {
                              n315 = Wait (ms)(milliseconds to wait=u32 500) -> ()  [unwired: 1 out]
                              n316 = local write "N fit"(100 ("N fit")) -> ()
                            }
                            frame #1 {
                              n317 = local write "Estagio auto"(8 ("Estagio auto")) -> ()
                            }
                          }
                        }
                      }
                      n318 = case shown="True" w582 {
                        tunnel: [TRUE ("Boolean") FALSE ("Boolean")] -> w581
                        frame False {
                        }
                        frame True {
                        }
                      }
                      n319 = case shown="False" w586 {
                        tunnel: w581 -> [_ w637]
                        frame False {
                          w635 = T5 3 items=["no dialog", "OK message", "continue or stop message", "OK message + warnings", "continue/stop + warnings"] ("type of dialog (OK msg:1)")
                          w631 = TRUE ("Boolean")
                          n320 = case shown="True" w631 {
                            frame False {
                            }
                            frame True {
                              n321 = property on="Vol Ref 3" class="Slide (strict)"() -> ("Value"=w636:dbl)  [unwired: 2 in, 2 out]
                              n322 = local write "Camara 2"(w636) -> ()
                            }
                          }
                          n323 = local write "Câmara 2"(w631) -> ()
                          n324 = call-poly <vilib>:"DAQmx Create Virtual Channel.vi"("lines"=tag "Dev1/port0/line3") -> ("task out"=w624:refnum<k21>, "error out"=w625:errorcluster)  [unwired: 13 in]
                          n325 = Wait (ms)(milliseconds to wait="patamar milliseconds to wait") -> ()  [unwired: 1 out]
                          n326 = call <vilib>:"DAQmx Start Task.vi"("task/channels in"=w624, "error in"=w625) -> ("task out"=w626:refnum<k21>, "error out"=w627:errorcluster)  [unwired: 12 in]
                          n327 = call-poly <vilib>:"DAQmx Write.vi"("task/channels in"=w626, "data"=w631, "error in"=w627) -> ("task out"=w632:refnum<k21>, "error out"=w633:errorcluster)  [unwired: 10 in, 1 out]
                          n328 = call <vilib>:"DAQmx Stop Task.vi"("task/channels in"=w632, "error in"=w633) -> ("task out"=w629:refnum<k21>, "error out"=w628:errorcluster)  [unwired: 12 in]
                          n329 = call <vilib>:"DAQmx Clear Task.vi"("task in"=w629, "error in"=w628) -> ("error out"=w634:errorcluster)  [unwired: 13 in]
                          n330 = call <vilib>:"Simple Error Handler.vi"("type of dialog (OK msg:1)"=w635, "error in (no error)"=w634) -> ()  [unwired: 3 in, 5 out]
                        }
                        frame True {
                          n331 = flat-sequence {
                            tunnel: w637 -> [w638]
                            frame #0 {
                              w640 = T5 3 items=["no dialog", "OK message", "continue or stop message", "OK message + warnings", "continue/stop + warnings"] ("type of dialog (OK msg:1)")
                              n332 = local write "Câmara 2"(w638) -> ()
                              n333 = call-poly <vilib>:"DAQmx Create Virtual Channel.vi"("lines"=tag "Dev1/port0/line3") -> ("task out"=w649:refnum<k21>, "error out"=w648:errorcluster)  [unwired: 13 in]
                              n334 = call <vilib>:"DAQmx Start Task.vi"("task/channels in"=w649, "error in"=w648) -> ("task out"=w647:refnum<k21>, "error out"=w646:errorcluster)  [unwired: 12 in]
                              n335 = call-poly <vilib>:"DAQmx Write.vi"("task/channels in"=w647, "data"=w638, "error in"=w646) -> ("task out"=w642:refnum<k21>, "error out"=w641:errorcluster)  [unwired: 10 in, 1 out]
                              n336 = call <vilib>:"DAQmx Stop Task.vi"("task/channels in"=w642, "error in"=w641) -> ("task out"=w644:refnum<k21>, "error out"=w645:errorcluster)  [unwired: 12 in]
                              n337 = call <vilib>:"DAQmx Clear Task.vi"("task in"=w644, "error in"=w645) -> ("error out"=w639:errorcluster)  [unwired: 13 in]
                              n338 = call <vilib>:"Simple Error Handler.vi"("type of dialog (OK msg:1)"=w640, "error in (no error)"=w639) -> ()  [unwired: 3 in, 5 out]
                            }
                            frame #1 {
                              n339 = Wait (ms)(milliseconds to wait=u32 2000) -> ()  [unwired: 1 out]
                            }
                          }
                        }
                      }
                    }
                  }
                }
                frame 8 {
                  n340 = property on="Contador" class="DigNum (strict)"() -> ("Value"=w679:i32)  [unwired: 2 in, 2 out]
                  n341 = Increment(x=w679) -> (x+1=w681:i32)
                  n342 = Equal?(x=w681, y=100) -> (x = y?=w678:bool)
                  n343 = case shown="False" w677 {
                    tunnel: [FALSE ("Save manual") w1275] -> w657
                    tunnel: w678 -> [_ w1275]
                    frame False {
                    }
                    frame True {
                    }
                  }
                  n344 = case shown="True" w678 {
                    tunnel: w682 -> [_ w1276]
                    frame False {
                    }
                    frame True {
                      n345 = property on="P fit" class="DigNum (strict)"() -> ("Value"=w1277:dbl)  [unwired: 2 in, 2 out]
                      n346 = Number To Fractional String(number=w1277, precision (6)=i16 3) -> (F-format string=w1281:string)  [unwired: 2 in]
                      n347 = Concatenate Strings(w1281, "\t") -> (w1279:string)
                      n348 = flat-sequence {
                        tunnel: [w1288] -> w1283
                        tunnel: [w1287] -> w1282
                        tunnel: w1279 -> [w1286]
                        tunnel: w1276 -> [w1285]
                        tunnel: w1283 -> [w1303]
                        tunnel: w1282 -> [w1302]
                        frame #0 {
                          n349 = Wait (ms)(milliseconds to wait=u32 500) -> ()  [unwired: 1 out]
                          n350 = Open/Create/Replace File(file path (use dialog)=w1285, operation (0:open)=T2."open") -> (refnum out=w1294:refnum<file>, error out=w1295:errorcluster)  [unwired: 2 in, 3 out]
                          n351 = Set File Position(refnum=w1294, from (0:start)=enum16{"start", "end", "current"}."end", error in=w1295) -> (refnum out=w1292:refnum<file>, error out=w1291:errorcluster)  [unwired: 1 in]
                          n352 = Write to Text File(file (use dialog)=w1292, text=w1286, error in=w1291) -> (refnum out=w1296:refnum<file>, error out=w1297:errorcluster)  [unwired: 2 out]
                          n353 = Close File(refnum=w1296, error in=w1297) -> (path=w1288:path, error out=w1289:errorcluster)
                          n354 = call <vilib>:"Simple Error Handler.vi"("error in (no error)"=w1289) -> ("error out"=w1287:errorcluster)  [unwired: 1 in, 7 out]
                        }
                        frame #1 {
                          n355 = local write "Estagio auto"(9 ("Estagio auto")) -> ()
                          n356 = local write "Pf2 2"(TRUE ("ZPit")) -> ()
                          n357 = Wait (ms)(milliseconds to wait=u32 500) -> ()  [unwired: 1 out]
                          n358 = Read from Text File(file (use dialog)=w1303, count=-1 ("Count  3"), error in=w1302) -> (refnum out=w1304:refnum<file>, text=w1308:string, error out=w1305:errorcluster)  [unwired: 1 in, 1 out]
                          n359 = local write "String 3"(w1308) -> ()
                          n360 = Close File(refnum=w1304, error in=w1305) -> (error out=w1306:errorcluster)  [unwired: 1 out]
                          n361 = local write "String"("abrir valvula vacuo" ("String")) -> ()
                          n362 = call <vilib>:"Simple Error Handler.vi"("error in (no error)"=w1306) -> ()  [unwired: 1 in, 8 out]
                        }
                      }
                    }
                  }
                  n363 = flat-sequence {
                    tunnel: w657 -> [w684]
                    tunnel: w660 -> [w685]
                    tunnel: [w685] -> w655
                    tunnel: [w684] -> w654
                    tunnel: [w687] -> w676
                    tunnel: [w689] -> w675
                    tunnel: [w690] -> w674
                    tunnel: [w691] -> w673
                    tunnel: [w692] -> w672
                    tunnel: [w693] -> w671
                    tunnel: [w694] -> w670
                    tunnel: [w695] -> w669
                    tunnel: [w696] -> w668
                    tunnel: [w697] -> w667
                    tunnel: [w698] -> w666
                    tunnel: [w699] -> w665
                    tunnel: [w700] -> w664
                    tunnel: [w701] -> w663
                    tunnel: [w702] -> w662
                    tunnel: [w688] -> w661
                    tunnel: [w686] -> w658
                    tunnel: w655 -> [w704]
                    tunnel: w654 -> [w703]
                    tunnel: w676 -> [w1225]
                    tunnel: w675 -> [w1224]
                    tunnel: w674 -> [w1223]
                    tunnel: w673 -> [w1222]
                    tunnel: w672 -> [w1221]
                    tunnel: w671 -> [w1220]
                    tunnel: w670 -> [w1219]
                    tunnel: w669 -> [w1218]
                    tunnel: w668 -> [w1217]
                    tunnel: w667 -> [w1216]
                    tunnel: w666 -> [w1215]
                    tunnel: w665 -> [w1214]
                    tunnel: w664 -> [w1213]
                    tunnel: w663 -> [w1212]
                    tunnel: w662 -> [w1211]
                    tunnel: w661 -> [w1210]
                    tunnel: [w1208] -> w659
                    tunnel: w658 -> [w1208]
                    tunnel: [TRUE ("graph RLC")] -> w656
                    frame #0 {
                      n364 = local write "graph RLC"(FALSE) -> ()
                    }
                    frame #1 {
                      n365 = case shown="False" w703 {
                        tunnel: [FALSE w741] -> w686
                        tunnel: w704 -> [_ w723]
                        tunnel: [_ w721] -> w687
                        tunnel: [_ w720] -> w688
                        tunnel: [_ w719] -> w689
                        tunnel: [_ w718] -> w690
                        tunnel: [_ w717] -> w691
                        tunnel: [_ w716] -> w692
                        tunnel: [_ w715] -> w693
                        tunnel: [_ w714] -> w694
                        tunnel: [_ w713] -> w695
                        tunnel: [_ w712] -> w696
                        tunnel: [_ w711] -> w697
                        tunnel: [_ w710] -> w698
                        tunnel: [_ w709] -> w699
                        tunnel: [_ w708] -> w700
                        tunnel: [_ w707] -> w701
                        tunnel: [_ w706] -> w702
                        frame False {
                        }
                        frame True {
                          n366 = property on="path RLC_completo" class="Path"() -> ("Value"=w722:path)  [unwired: 2 in, 2 out]
                          n367 = for {
                            N: 5 -> [_]
                            tunnel: TRUE -> [w764]
                            tunnel: FALSE -> [w763]
                            tunnel: [w762] -> w741
                            tunnel: [w761] -> w739 mode=indexing
                            tunnel: [w760] -> w738 mode=indexing
                            tunnel: [w759] -> w737 mode=indexing
                            tunnel: [w758] -> w736 mode=indexing
                            tunnel: [w757] -> w735 mode=indexing
                            tunnel: [w756] -> w734 mode=indexing
                            tunnel: [w755] -> w733 mode=indexing
                            tunnel: [w754] -> w732 mode=indexing
                            tunnel: [w753] -> w731 mode=indexing
                            tunnel: [w752] -> w730 mode=indexing
                            tunnel: [w751] -> w729 mode=indexing
                            tunnel: [w750] -> w728 mode=indexing
                            tunnel: [w749] -> w727 mode=indexing
                            tunnel: [w748] -> w726 mode=indexing
                            tunnel: [w747] -> w725 mode=indexing
                            tunnel: [w746] -> w724 mode=indexing
                            tunnel: w723 -> [w745]
                            tunnel: w722 -> [w744]
                            n368 = stacked-sequence {
                              tunnel: w764 -> [_ w812 w838 w865 w890 w917 w942 w969 w995 w1020 w1046 w1072 w1098 w1124 w1150 w1176 w1203 _]
                              tunnel: w763 -> [w786 _ _ _ _ _ _ _ _ _ _ _ _ _ _ _ _ w1207]
                              tunnel: [_ _ _ _ _ _ _ _ _ _ _ _ _ _ _ _ _ TRUE] -> w762
                              tunnel: [_ w792 _ _ _ _ _ _ _ _ _ _ _ _ _ _ _ _] -> w761
                              tunnel: [_ _ w818 _ _ _ _ _ _ _ _ _ _ _ _ _ _ _] -> w760
                              tunnel: [_ _ _ w844 _ _ _ _ _ _ _ _ _ _ _ _ _ _] -> w759
                              tunnel: [_ _ _ _ w870 _ _ _ _ _ _ _ _ _ _ _ _ _] -> w758
                              tunnel: [_ _ _ _ _ w896 _ _ _ _ _ _ _ _ _ _ _ _] -> w757
                              tunnel: [_ _ _ _ _ _ w922 _ _ _ _ _ _ _ _ _ _ _] -> w756
                              tunnel: [_ _ _ _ _ _ _ w948 _ _ _ _ _ _ _ _ _ _] -> w755
                              tunnel: [_ _ _ _ _ _ _ _ w974 _ _ _ _ _ _ _ _ _] -> w754
                              tunnel: [_ _ _ _ _ _ _ _ _ w1000 _ _ _ _ _ _ _ _] -> w753
                              tunnel: [_ _ _ _ _ _ _ _ _ _ w1026 _ _ _ _ _ _ _] -> w752
                              tunnel: [_ _ _ _ _ _ _ _ _ _ _ w1052 _ _ _ _ _ _] -> w751
                              tunnel: [_ _ _ _ _ _ _ _ _ _ _ _ w1078 _ _ _ _ _] -> w750
                              tunnel: [_ _ _ _ _ _ _ _ _ _ _ _ _ w1104 _ _ _ _] -> w749
                              tunnel: [_ _ _ _ _ _ _ _ _ _ _ _ _ _ w1130 _ _ _] -> w748
                              tunnel: [_ _ _ _ _ _ _ _ _ _ _ _ _ _ _ w1156 _ _] -> w747
                              tunnel: [_ _ _ _ _ _ _ _ _ _ _ _ _ _ _ _ w1182 _] -> w746
                              tunnel: w745 -> [_ w791 w817 w843 w869 w895 w921 w947 w973 w999 w1025 w1051 w1077 w1103 w1129 w1155 w1181 _]
                              tunnel: w744 -> [w765 w787 w815 w841 w867 w893 w919 w945 w971 w997 w1023 w1049 w1075 w1101 w1127 w1153 w1179 _]
                              frame #0 {
                                w766 = "\t"
                                n369 = local write "C-50-L"(w786) -> ()
                                n370 = local write "C-50-N"(w786) -> ()
                                n371 = local write "Z-50-L"(w786) -> ()
                                n372 = local write "C-1K-N"(w786) -> ()
                                n373 = local write "C-1K-L"(w786) -> ()
                                n374 = local write "Z-50-N"(w786) -> ()
                                n375 = local write "Z-1K-N"(w786) -> ()
                                n376 = local write "Z-1K-L"(w786) -> ()
                                n377 = local write "C-10K-L"(w786) -> ()
                                n378 = local write "C-100-N"(w786) -> ()
                                n379 = local write "C-10K-N"(w786) -> ()
                                n380 = local write "Z-100-L"(w786) -> ()
                                n381 = local write "Z-10K-L"(w786) -> ()
                                n382 = local write "Z-100-N"(w786) -> ()
                                n383 = local write "Z-10K-N"(w786) -> ()
                                n384 = local write "C-100-L"(w786) -> ()
                                n385 = Open/Create/Replace File(file path (use dialog)=w765, operation (0:open)=T2."open") -> (refnum out=w780:refnum<file>, error out=w779:errorcluster)  [unwired: 2 in, 3 out]
                                n386 = Get Date/Time String(date format (0)=enum16{"short", "long", "abbreviated"}."short", want seconds? (F)=TRUE) -> (date string=w772:string, time string=w771:string)  [unwired: 1 in]
                                n387 = feedback #1() -> (w770:dbl)  [unwired: 1 in]
                                "SET 2" <- w770
                                n388 = Set File Position(refnum=w780, from (0:start)=enum16{"start", "end", "current"}."end", error in=w779) -> (refnum out=w782:refnum<file>, error out=w783:errorcluster)  [unwired: 1 in]
                                n389 = Number To Fractional String(number=w770, precision (6)=i16 2) -> (F-format string=w769:string)  [unwired: 2 in]
                                n390 = Add(x=w770, y=0.2) -> (x+y=w776:dbl)
                                n391 = feedback-in #1(w776) -> ()
                                n392 = Concatenate Strings(w769, w766, w772, w766, w771, w766) -> (w768:string)
                                n393 = Write to Text File(file (use dialog)=w782, text=w768, error in=w783) -> (refnum out=w778:refnum<file>, error out=w777:errorcluster)  [unwired: 1 in, 1 out]
                                n394 = Close File(refnum=w778, error in=w777) -> (error out=w785:errorcluster)  [unwired: 1 out]
                                n395 = call <vilib>:"Simple Error Handler.vi"("error in (no error)"=w785) -> ()  [unwired: 1 in, 8 out]
                              }
                              frame #1 {
                                w793 = "\t"
                                w811 = i16 4 ("width (-)")
                                n396 = Open/Create/Replace File(file path (use dialog)=w787, operation (0:open)=T2."open") -> (refnum out=w802:refnum<file>, error out=w801:errorcluster)  [unwired: 2 in, 3 out]
                                n397 = Multiply(x="Time RLC", y=u32 1000) -> (x*y=w790:u32)
                                n398 = Wait (ms)(milliseconds to wait=w790) -> ()  [unwired: 1 out]
                                n399 = Set File Position(refnum=w802, from (0:start)=enum16{"start", "end", "current"}."end", error in=w801) -> (refnum out=w804:refnum<file>, error out=w805:errorcluster)  [unwired: 1 in]
                                n400 = call "RLC_read.vi"("Path"=w791, "String"="cmd /c rlc_read_cAL.py") -> ("MEASURE A"=w792:dbl, "MEASURE V [V]"=w809:dbl, "concatenated string"=w813:string, "MEASURE B"=w810:dbl, "MEASURE I [A]"=w808:dbl)  [unwired: 1 out]
                                "MEASURE A" <- w792
                                "MEASURE B" <- w810
                                n401 = Number To Engineering String(2:w811, 4:w808) -> (0:w794:string)  [unwired: 2 in]
                                n402 = local write "RLC300 - digimess"(w813) -> ()
                                n403 = Number To Engineering String(2:w811, 4:w809) -> (0:w795:string)  [unwired: 2 in]
                                n404 = Number To Engineering String(2:w811, 4:w792) -> (0:w797:string)  [unwired: 2 in]
                                n405 = Number To Engineering String(2:w811, 4:w810) -> (0:w796:string)  [unwired: 2 in]
                                n406 = Concatenate Strings(w797, w793, w796, w793, w795, w793, w794, w793) -> (w798:string)
                                n407 = Write to Text File(file (use dialog)=w804, text=w798, error in=w805) -> (refnum out=w800:refnum<file>, error out=w799:errorcluster)  [unwired: 1 in, 1 out]
                                n408 = Close File(refnum=w800, error in=w799) -> (error out=w807:errorcluster)  [unwired: 1 out]
                                n409 = call <vilib>:"Simple Error Handler.vi"("error in (no error)"=w807) -> ()  [unwired: 1 in, 8 out]
                                "C-50-L" <- w812
                              }
                              frame #2 {
                                w822 = "\t"
                                w837 = i16 4 ("width (-)")
                                n410 = property on="Time RLC" class="DigNum (strict)"() -> ("Value"=w816:u32)  [unwired: 2 in, 2 out]
                                n411 = Wait (ms)(milliseconds to wait=w816) -> ()  [unwired: 1 out]
                                n412 = Open/Create/Replace File(file path (use dialog)=w815, operation (0:open)=T2."open") -> (refnum out=w831:refnum<file>, error out=w830:errorcluster)  [unwired: 2 in, 3 out]
                                n413 = Set File Position(refnum=w831, from (0:start)=enum16{"start", "end", "current"}."end", error in=w830) -> (refnum out=w833:refnum<file>, error out=w834:errorcluster)  [unwired: 1 in]
                                n414 = call "RLC_read.vi"("Path"=w817, "String"="cmd /c rlc_read_cAN.py") -> ("MEASURE A"=w818:dbl, "MEASURE V [V]"=w820:dbl, "concatenated string"=w840:string, "MEASURE B"=w821:dbl, "MEASURE I [A]"=w819:dbl)  [unwired: 1 out]
                                "MEASURE A 2" <- w818
                                "MEASURE B 2" <- w821
                                n415 = Number To Engineering String(2:w837, 4:w819) -> (0:w823:string)  [unwired: 2 in]
                                n416 = local write "RLC300 - digimess"(w840) -> ()
                                n417 = Number To Engineering String(2:w837, 4:w820) -> (0:w824:string)  [unwired: 2 in]
                                n418 = Number To Engineering String(2:w837, 4:w818) -> (0:w826:string)  [unwired: 2 in]
                                n419 = Number To Engineering String(2:w837, 4:w821) -> (0:w825:string)  [unwired: 2 in]
                                n420 = Concatenate Strings(w826, w822, w825, w822, w824, w822, w823, w822) -> (w827:string)
                                n421 = Write to Text File(file (use dialog)=w833, text=w827, error in=w834) -> (refnum out=w829:refnum<file>, error out=w828:errorcluster)  [unwired: 1 in, 1 out]
                                n422 = Close File(refnum=w829, error in=w828) -> (error out=w836:errorcluster)  [unwired: 1 out]
                                n423 = call <vilib>:"Simple Error Handler.vi"("error in (no error)"=w836) -> ()  [unwired: 1 in, 8 out]
                                "C-50-N" <- w838
                              }
                              frame #3 {
                                w848 = "\t"
                                w863 = i16 4 ("width (-)")
                                n424 = property on="Time RLC" class="DigNum (strict)"() -> ("Value"=w842:u32)  [unwired: 2 in, 2 out]
                                n425 = Wait (ms)(milliseconds to wait=w842) -> ()  [unwired: 1 out]
                                n426 = Open/Create/Replace File(file path (use dialog)=w841, operation (0:open)=T2."open") -> (refnum out=w857:refnum<file>, error out=w856:errorcluster)  [unwired: 2 in, 3 out]
                                n427 = Set File Position(refnum=w857, from (0:start)=enum16{"start", "end", "current"}."end", error in=w856) -> (refnum out=w859:refnum<file>, error out=w860:errorcluster)  [unwired: 1 in]
                                n428 = call "RLC_read.vi"("Path"=w843, "String"="cmd /c rlc_read_cBL.py") -> ("MEASURE A"=w844:dbl, "MEASURE V [V]"=w846:dbl, "concatenated string"=w866:string, "MEASURE B"=w847:dbl, "MEASURE I [A]"=w845:dbl)  [unwired: 1 out]
                                "MEASURE A 3" <- w844
                                "MEASURE B 3" <- w847
                                n429 = Number To Engineering String(2:w863, 4:w845) -> (0:w849:string)  [unwired: 2 in]
                                n430 = local write "RLC300 - digimess"(w866) -> ()
                                n431 = Number To Engineering String(2:w863, 4:w846) -> (0:w850:string)  [unwired: 2 in]
                                n432 = Number To Engineering String(2:w863, 4:w844) -> (0:w852:string)  [unwired: 2 in]
                                n433 = Number To Engineering String(2:w863, 4:w847) -> (0:w851:string)  [unwired: 2 in]
                                n434 = Concatenate Strings(w852, w848, w851, w848, w850, w848, w849, w848) -> (w853:string)
                                n435 = Write to Text File(file (use dialog)=w859, text=w853, error in=w860) -> (refnum out=w855:refnum<file>, error out=w854:errorcluster)  [unwired: 1 in, 1 out]
                                n436 = Close File(refnum=w855, error in=w854) -> (error out=w862:errorcluster)  [unwired: 1 out]
                                n437 = call <vilib>:"Simple Error Handler.vi"("error in (no error)"=w862) -> ()  [unwired: 1 in, 8 out]
                                "C-100-L" <- w865
                              }
                              frame #4 {
                                w874 = "\t"
                                w889 = i16 4 ("width (-)")
                                n438 = property on="Time RLC" class="DigNum (strict)"() -> ("Value"=w868:u32)  [unwired: 2 in, 2 out]
                                n439 = Wait (ms)(milliseconds to wait=w868) -> ()  [unwired: 1 out]
                                n440 = Open/Create/Replace File(file path (use dialog)=w867, operation (0:open)=T2."open") -> (refnum out=w883:refnum<file>, error out=w882:errorcluster)  [unwired: 2 in, 3 out]
                                n441 = Set File Position(refnum=w883, from (0:start)=enum16{"start", "end", "current"}."end", error in=w882) -> (refnum out=w885:refnum<file>, error out=w886:errorcluster)  [unwired: 1 in]
                                n442 = call "RLC_read.vi"("Path"=w869, "String"="cmd /c rlc_read_cBN.py") -> ("MEASURE A"=w870:dbl, "MEASURE V [V]"=w872:dbl, "concatenated string"=w892:string, "MEASURE B"=w873:dbl, "MEASURE I [A]"=w871:dbl)  [unwired: 1 out]
                                "MEASURE A 4" <- w870
                                "MEASURE B 4" <- w873
                                n443 = Number To Engineering String(2:w889, 4:w871) -> (0:w875:string)  [unwired: 2 in]
                                n444 = local write "RLC300 - digimess"(w892) -> ()
                                n445 = Number To Engineering String(2:w889, 4:w872) -> (0:w876:string)  [unwired: 2 in]
                                n446 = Number To Engineering String(2:w889, 4:w870) -> (0:w878:string)  [unwired: 2 in]
                                n447 = Number To Engineering String(2:w889, 4:w873) -> (0:w877:string)  [unwired: 2 in]
                                n448 = Concatenate Strings(w878, w874, w877, w874, w876, w874, w875, w874) -> (w879:string)
                                n449 = Write to Text File(file (use dialog)=w885, text=w879, error in=w886) -> (refnum out=w881:refnum<file>, error out=w880:errorcluster)  [unwired: 1 in, 1 out]
                                n450 = Close File(refnum=w881, error in=w880) -> (error out=w888:errorcluster)  [unwired: 1 out]
                                n451 = call <vilib>:"Simple Error Handler.vi"("error in (no error)"=w888) -> ()  [unwired: 1 in, 8 out]
                                "C-100-N" <- w890
                              }
                              frame #5 {
                                w915 = "\t"
                                w900 = i16 4 ("width (-)")
                                n452 = property on="Time RLC" class="DigNum (strict)"() -> ("Value"=w894:u32)  [unwired: 2 in, 2 out]
                                n453 = Wait (ms)(milliseconds to wait=w894) -> ()  [unwired: 1 out]
                                n454 = Open/Create/Replace File(file path (use dialog)=w893, operation (0:open)=T2."open") -> (refnum out=w906:refnum<file>, error out=w907:errorcluster)  [unwired: 2 in, 3 out]
                                n455 = Set File Position(refnum=w906, from (0:start)=enum16{"start", "end", "current"}."end", error in=w907) -> (refnum out=w904:refnum<file>, error out=w903:errorcluster)  [unwired: 1 in]
                                n456 = call "RLC_read.vi"("Path"=w895, "String"="cmd /c rlc_read_cCL.py") -> ("MEASURE A"=w896:dbl, "MEASURE V [V]"=w898:dbl, "concatenated string"=w918:string, "MEASURE B"=w899:dbl, "MEASURE I [A]"=w897:dbl)  [unwired: 1 out]
                                "MEASURE A 5" <- w896
                                "MEASURE B 5" <- w899
                                n457 = Number To Engineering String(2:w900, 4:w897) -> (0:w914:string)  [unwired: 2 in]
                                n458 = local write "RLC300 - digimess"(w918) -> ()
                                n459 = Number To Engineering String(2:w900, 4:w898) -> (0:w913:string)  [unwired: 2 in]
                                n460 = Number To Engineering String(2:w900, 4:w896) -> (0:w911:string)  [unwired: 2 in]
                                n461 = Number To Engineering String(2:w900, 4:w899) -> (0:w912:string)  [unwired: 2 in]
                                n462 = Concatenate Strings(w911, w915, w912, w915, w913, w915, w914, w915) -> (w910:string)
                                n463 = Write to Text File(file (use dialog)=w904, text=w910, error in=w903) -> (refnum out=w908:refnum<file>, error out=w909:errorcluster)  [unwired: 1 in, 1 out]
                                n464 = Close File(refnum=w908, error in=w909) -> (error out=w901:errorcluster)  [unwired: 1 out]
                                n465 = call <vilib>:"Simple Error Handler.vi"("error in (no error)"=w901) -> ()  [unwired: 1 in, 8 out]
                                "C-1K-L" <- w917
                              }
                              frame #6 {
                                w941 = "\t"
                                w926 = i16 4 ("width (-)")
                                n466 = property on="Time RLC" class="DigNum (strict)"() -> ("Value"=w920:u32)  [unwired: 2 in, 2 out]
                                n467 = Wait (ms)(milliseconds to wait=w920) -> ()  [unwired: 1 out]
                                n468 = Open/Create/Replace File(file path (use dialog)=w919, operation (0:open)=T2."open") -> (refnum out=w932:refnum<file>, error out=w933:errorcluster)  [unwired: 2 in, 3 out]
                                n469 = Set File Position(refnum=w932, from (0:start)=enum16{"start", "end", "current"}."end", error in=w933) -> (refnum out=w930:refnum<file>, error out=w929:errorcluster)  [unwired: 1 in]
                                n470 = call "RLC_read.vi"("Path"=w921, "String"="cmd /c rlc_read_cCN.py") -> ("MEASURE A"=w922:dbl, "MEASURE V [V]"=w924:dbl, "concatenated string"=w944:string, "MEASURE B"=w925:dbl, "MEASURE I [A]"=w923:dbl)  [unwired: 1 out]
                                "MEASURE A 6" <- w922
                                "MEASURE B 6" <- w925
                                n471 = Number To Engineering String(2:w926, 4:w923) -> (0:w940:string)  [unwired: 2 in]
                                n472 = local write "RLC300 - digimess"(w944) -> ()
                                n473 = Number To Engineering String(2:w926, 4:w924) -> (0:w939:string)  [unwired: 2 in]
                                n474 = Number To Engineering String(2:w926, 4:w922) -> (0:w937:string)  [unwired: 2 in]
                                n475 = Number To Engineering String(2:w926, 4:w925) -> (0:w938:string)  [unwired: 2 in]
                                n476 = Concatenate Strings(w937, w941, w938, w941, w939, w941, w940, w941) -> (w936:string)
                                n477 = Write to Text File(file (use dialog)=w930, text=w936, error in=w929) -> (refnum out=w934:refnum<file>, error out=w935:errorcluster)  [unwired: 1 in, 1 out]
                                n478 = Close File(refnum=w934, error in=w935) -> (error out=w927:errorcluster)  [unwired: 1 out]
                                n479 = call <vilib>:"Simple Error Handler.vi"("error in (no error)"=w927) -> ()  [unwired: 1 in, 8 out]
                                "C-1K-N" <- w942
                              }
                              frame #7 {
                                w952 = "\t"
                                w967 = i16 4 ("width (-)")
                                n480 = property on="Time RLC" class="DigNum (strict)"() -> ("Value"=w946:u32)  [unwired: 2 in, 2 out]
                                n481 = Wait (ms)(milliseconds to wait=w946) -> ()  [unwired: 1 out]
                                n482 = Open/Create/Replace File(file path (use dialog)=w945, operation (0:open)=T2."open") -> (refnum out=w961:refnum<file>, error out=w960:errorcluster)  [unwired: 2 in, 3 out]
                                n483 = Set File Position(refnum=w961, from (0:start)=enum16{"start", "end", "current"}."end", error in=w960) -> (refnum out=w963:refnum<file>, error out=w964:errorcluster)  [unwired: 1 in]
                                n484 = call "RLC_read.vi"("Path"=w947, "String"="cmd /c rlc_read_cDL.py") -> ("MEASURE A"=w948:dbl, "MEASURE V [V]"=w950:dbl, "concatenated string"=w970:string, "MEASURE B"=w951:dbl, "MEASURE I [A]"=w949:dbl)  [unwired: 1 out]
                                "MEASURE A 7" <- w948
                                "MEASURE B 7" <- w951
                                n485 = Number To Engineering String(2:w967, 4:w949) -> (0:w953:string)  [unwired: 2 in]
                                n486 = local write "RLC300 - digimess"(w970) -> ()
                                n487 = Number To Engineering String(2:w967, 4:w950) -> (0:w954:string)  [unwired: 2 in]
                                n488 = Number To Engineering String(2:w967, 4:w948) -> (0:w956:string)  [unwired: 2 in]
                                n489 = Number To Engineering String(2:w967, 4:w951) -> (0:w955:string)  [unwired: 2 in]
                                n490 = Concatenate Strings(w956, w952, w955, w952, w954, w952, w953, w952) -> (w957:string)
                                n491 = Write to Text File(file (use dialog)=w963, text=w957, error in=w964) -> (refnum out=w959:refnum<file>, error out=w958:errorcluster)  [unwired: 1 in, 1 out]
                                n492 = Close File(refnum=w959, error in=w958) -> (error out=w966:errorcluster)  [unwired: 1 out]
                                n493 = call <vilib>:"Simple Error Handler.vi"("error in (no error)"=w966) -> ()  [unwired: 1 in, 8 out]
                                "C-10K-L" <- w969
                              }
                              frame #8 {
                                w978 = "\t"
                                w993 = i16 4 ("width (-)")
                                n494 = property on="Time RLC" class="DigNum (strict)"() -> ("Value"=w972:u32)  [unwired: 2 in, 2 out]
                                n495 = Wait (ms)(milliseconds to wait=w972) -> ()  [unwired: 1 out]
                                n496 = Open/Create/Replace File(file path (use dialog)=w971, operation (0:open)=T2."open") -> (refnum out=w987:refnum<file>, error out=w986:errorcluster)  [unwired: 2 in, 3 out]
                                n497 = Set File Position(refnum=w987, from (0:start)=enum16{"start", "end", "current"}."end", error in=w986) -> (refnum out=w989:refnum<file>, error out=w990:errorcluster)  [unwired: 1 in]
                                n498 = call "RLC_read.vi"("Path"=w973, "String"="cmd /c rlc_read_cDN.py") -> ("MEASURE A"=w974:dbl, "MEASURE V [V]"=w976:dbl, "concatenated string"=w996:string, "MEASURE B"=w977:dbl, "MEASURE I [A]"=w975:dbl)  [unwired: 1 out]
                                "MEASURE A 8" <- w974
                                "MEASURE B 8" <- w977
                                n499 = Number To Engineering String(2:w993, 4:w975) -> (0:w979:string)  [unwired: 2 in]
                                n500 = local write "RLC300 - digimess"(w996) -> ()
                                n501 = Number To Engineering String(2:w993, 4:w976) -> (0:w980:string)  [unwired: 2 in]
                                n502 = Number To Engineering String(2:w993, 4:w974) -> (0:w982:string)  [unwired: 2 in]
                                n503 = Number To Engineering String(2:w993, 4:w977) -> (0:w981:string)  [unwired: 2 in]
                                n504 = Concatenate Strings(w982, w978, w981, w978, w980, w978, w979, w978) -> (w983:string)
                                n505 = Write to Text File(file (use dialog)=w989, text=w983, error in=w990) -> (refnum out=w985:refnum<file>, error out=w984:errorcluster)  [unwired: 1 in, 1 out]
                                n506 = Close File(refnum=w985, error in=w984) -> (error out=w992:errorcluster)  [unwired: 1 out]
                                n507 = call <vilib>:"Simple Error Handler.vi"("error in (no error)"=w992) -> ()  [unwired: 1 in, 8 out]
                                "C-10K-N" <- w995
                              }
                              frame #9 {
                                w1004 = "\t"
                                w1019 = i16 4 ("width (-)")
                                n508 = property on="Time RLC" class="DigNum (strict)"() -> ("Value"=w998:u32)  [unwired: 2 in, 2 out]
                                n509 = Wait (ms)(milliseconds to wait=w998) -> ()  [unwired: 1 out]
                                n510 = Open/Create/Replace File(file path (use dialog)=w997, operation (0:open)=T2."open") -> (refnum out=w1013:refnum<file>, error out=w1012:errorcluster)  [unwired: 2 in, 3 out]
                                n511 = Set File Position(refnum=w1013, from (0:start)=enum16{"start", "end", "current"}."end", error in=w1012) -> (refnum out=w1015:refnum<file>, error out=w1016:errorcluster)  [unwired: 1 in]
                                n512 = call "RLC_read.vi"("Path"=w999, "String"="cmd /c rlc_read_ZAL.py") -> ("MEASURE A"=w1000:dbl, "MEASURE V [V]"=w1002:dbl, "concatenated string"=w1021:string, "MEASURE B"=w1003:dbl, "MEASURE I [A]"=w1001:dbl)  [unwired: 1 out]
                                "MEASURE A 9" <- w1000
                                "MEASURE B 9" <- w1003
                                n513 = Number To Engineering String(2:w1019, 4:w1001) -> (0:w1005:string)  [unwired: 2 in]
                                n514 = local write "RLC300 - digimess"(w1021) -> ()
                                n515 = Number To Engineering String(2:w1019, 4:w1002) -> (0:w1006:string)  [unwired: 2 in]
                                n516 = Number To Engineering String(2:w1019, 4:w1000) -> (0:w1008:string)  [unwired: 2 in]
                                n517 = Number To Engineering String(2:w1019, 4:w1003) -> (0:w1007:string)  [unwired: 2 in]
                                n518 = Concatenate Strings(w1008, w1004, w1007, w1004, w1006, w1004, w1005, w1004) -> (w1009:string)
                                n519 = Write to Text File(file (use dialog)=w1015, text=w1009, error in=w1016) -> (refnum out=w1011:refnum<file>, error out=w1010:errorcluster)  [unwired: 1 in, 1 out]
                                n520 = Close File(refnum=w1011, error in=w1010) -> (error out=w1018:errorcluster)  [unwired: 1 out]
                                n521 = call <vilib>:"Simple Error Handler.vi"("error in (no error)"=w1018) -> ()  [unwired: 1 in, 8 out]
                                "Z-50-L" <- w1020
                              }
                              frame #10 {
                                w1030 = "\t"
                                w1045 = i16 4 ("width (-)")
                                n522 = property on="Time RLC" class="DigNum (strict)"() -> ("Value"=w1024:u32)  [unwired: 2 in, 2 out]
                                n523 = Wait (ms)(milliseconds to wait=w1024) -> ()  [unwired: 1 out]
                                n524 = Open/Create/Replace File(file path (use dialog)=w1023, operation (0:open)=T2."open") -> (refnum out=w1039:refnum<file>, error out=w1038:errorcluster)  [unwired: 2 in, 3 out]
                                n525 = Set File Position(refnum=w1039, from (0:start)=enum16{"start", "end", "current"}."end", error in=w1038) -> (refnum out=w1041:refnum<file>, error out=w1042:errorcluster)  [unwired: 1 in]
                                n526 = call "RLC_read.vi"("Path"=w1025, "String"="cmd /c rlc_read_ZAN.py") -> ("MEASURE A"=w1026:dbl, "MEASURE V [V]"=w1028:dbl, "concatenated string"=w1047:string, "MEASURE B"=w1029:dbl, "MEASURE I [A]"=w1027:dbl)  [unwired: 1 out]
                                "MEASURE A 10" <- w1026
                                "MEASURE B 10" <- w1029
                                n527 = Number To Engineering String(2:w1045, 4:w1027) -> (0:w1031:string)  [unwired: 2 in]
                                n528 = local write "RLC300 - digimess"(w1047) -> ()
                                n529 = Number To Engineering String(2:w1045, 4:w1028) -> (0:w1032:string)  [unwired: 2 in]
                                n530 = Number To Engineering String(2:w1045, 4:w1026) -> (0:w1034:string)  [unwired: 2 in]
                                n531 = Number To Engineering String(2:w1045, 4:w1029) -> (0:w1033:string)  [unwired: 2 in]
                                n532 = Concatenate Strings(w1034, w1030, w1033, w1030, w1032, w1030, w1031, w1030) -> (w1035:string)
                                n533 = Write to Text File(file (use dialog)=w1041, text=w1035, error in=w1042) -> (refnum out=w1037:refnum<file>, error out=w1036:errorcluster)  [unwired: 1 in, 1 out]
                                n534 = Close File(refnum=w1037, error in=w1036) -> (error out=w1044:errorcluster)  [unwired: 1 out]
                                n535 = call <vilib>:"Simple Error Handler.vi"("error in (no error)"=w1044) -> ()  [unwired: 1 in, 8 out]
                                "Z-50-N" <- w1046
                              }
                              frame #11 {
                                w1056 = "\t"
                                w1071 = i16 4 ("width (-)")
                                n536 = property on="Time RLC" class="DigNum (strict)"() -> ("Value"=w1050:u32)  [unwired: 2 in, 2 out]
                                n537 = Wait (ms)(milliseconds to wait=w1050) -> ()  [unwired: 1 out]
                                n538 = Open/Create/Replace File(file path (use dialog)=w1049, operation (0:open)=T2."open") -> (refnum out=w1065:refnum<file>, error out=w1064:errorcluster)  [unwired: 2 in, 3 out]
                                n539 = Set File Position(refnum=w1065, from (0:start)=enum16{"start", "end", "current"}."end", error in=w1064) -> (refnum out=w1067:refnum<file>, error out=w1068:errorcluster)  [unwired: 1 in]
                                n540 = call "RLC_read.vi"("Path"=w1051, "String"="cmd /c rlc_read_ZBL.py") -> ("MEASURE A"=w1052:dbl, "MEASURE V [V]"=w1054:dbl, "concatenated string"=w1073:string, "MEASURE B"=w1055:dbl, "MEASURE I [A]"=w1053:dbl)  [unwired: 1 out]
                                "MEASURE A 11" <- w1052
                                "MEASURE B 11" <- w1055
                                n541 = Number To Engineering String(2:w1071, 4:w1053) -> (0:w1057:string)  [unwired: 2 in]
                                n542 = local write "RLC300 - digimess"(w1073) -> ()
                                n543 = Number To Engineering String(2:w1071, 4:w1054) -> (0:w1058:string)  [unwired: 2 in]
                                n544 = Number To Engineering String(2:w1071, 4:w1052) -> (0:w1060:string)  [unwired: 2 in]
                                n545 = Number To Engineering String(2:w1071, 4:w1055) -> (0:w1059:string)  [unwired: 2 in]
                                n546 = Concatenate Strings(w1060, w1056, w1059, w1056, w1058, w1056, w1057, w1056) -> (w1061:string)
                                n547 = Write to Text File(file (use dialog)=w1067, text=w1061, error in=w1068) -> (refnum out=w1063:refnum<file>, error out=w1062:errorcluster)  [unwired: 1 in, 1 out]
                                n548 = Close File(refnum=w1063, error in=w1062) -> (error out=w1070:errorcluster)  [unwired: 1 out]
                                n549 = call <vilib>:"Simple Error Handler.vi"("error in (no error)"=w1070) -> ()  [unwired: 1 in, 8 out]
                                "Z-100-L" <- w1072
                              }
                              frame #12 {
                                w1082 = "\t"
                                w1097 = i16 4 ("width (-)")
                                n550 = property on="Time RLC" class="DigNum (strict)"() -> ("Value"=w1076:u32)  [unwired: 2 in, 2 out]
                                n551 = Wait (ms)(milliseconds to wait=w1076) -> ()  [unwired: 1 out]
                                n552 = Open/Create/Replace File(file path (use dialog)=w1075, operation (0:open)=T2."open") -> (refnum out=w1091:refnum<file>, error out=w1090:errorcluster)  [unwired: 2 in, 3 out]
                                n553 = Set File Position(refnum=w1091, from (0:start)=enum16{"start", "end", "current"}."end", error in=w1090) -> (refnum out=w1093:refnum<file>, error out=w1094:errorcluster)  [unwired: 1 in]
                                n554 = call "RLC_read.vi"("Path"=w1077, "String"="cmd /c rlc_read_ZBN.py") -> ("MEASURE A"=w1078:dbl, "MEASURE V [V]"=w1080:dbl, "concatenated string"=w1099:string, "MEASURE B"=w1081:dbl, "MEASURE I [A]"=w1079:dbl)  [unwired: 1 out]
                                "MEASURE A 12" <- w1078
                                "MEASURE B 12" <- w1081
                                n555 = Number To Engineering String(2:w1097, 4:w1079) -> (0:w1083:string)  [unwired: 2 in]
                                n556 = local write "RLC300 - digimess"(w1099) -> ()
                                n557 = Number To Engineering String(2:w1097, 4:w1080) -> (0:w1084:string)  [unwired: 2 in]
                                n558 = Number To Engineering String(2:w1097, 4:w1078) -> (0:w1086:string)  [unwired: 2 in]
                                n559 = Number To Engineering String(2:w1097, 4:w1081) -> (0:w1085:string)  [unwired: 2 in]
                                n560 = Concatenate Strings(w1086, w1082, w1085, w1082, w1084, w1082, w1083, w1082) -> (w1087:string)
                                n561 = Write to Text File(file (use dialog)=w1093, text=w1087, error in=w1094) -> (refnum out=w1089:refnum<file>, error out=w1088:errorcluster)  [unwired: 1 in, 1 out]
                                n562 = Close File(refnum=w1089, error in=w1088) -> (error out=w1096:errorcluster)  [unwired: 1 out]
                                n563 = call <vilib>:"Simple Error Handler.vi"("error in (no error)"=w1096) -> ()  [unwired: 1 in, 8 out]
                                "Z-100-N" <- w1098
                              }
                              frame #13 {
                                w1108 = "\t"
                                w1123 = i16 4 ("width (-)")
                                n564 = property on="Time RLC" class="DigNum (strict)"() -> ("Value"=w1102:u32)  [unwired: 2 in, 2 out]
                                n565 = Wait (ms)(milliseconds to wait=w1102) -> ()  [unwired: 1 out]
                                n566 = Open/Create/Replace File(file path (use dialog)=w1101, operation (0:open)=T2."open") -> (refnum out=w1117:refnum<file>, error out=w1116:errorcluster)  [unwired: 2 in, 3 out]
                                n567 = Set File Position(refnum=w1117, from (0:start)=enum16{"start", "end", "current"}."end", error in=w1116) -> (refnum out=w1119:refnum<file>, error out=w1120:errorcluster)  [unwired: 1 in]
                                n568 = call "RLC_read.vi"("Path"=w1103, "String"="cmd /c rlc_read_ZCL.py") -> ("MEASURE A"=w1104:dbl, "MEASURE V [V]"=w1106:dbl, "concatenated string"=w1125:string, "MEASURE B"=w1107:dbl, "MEASURE I [A]"=w1105:dbl)  [unwired: 1 out]
                                "MEASURE A 13" <- w1104
                                "MEASURE B 13" <- w1107
                                n569 = Number To Engineering String(2:w1123, 4:w1105) -> (0:w1109:string)  [unwired: 2 in]
                                n570 = local write "RLC300 - digimess"(w1125) -> ()
                                n571 = Number To Engineering String(2:w1123, 4:w1106) -> (0:w1110:string)  [unwired: 2 in]
                                n572 = Number To Engineering String(2:w1123, 4:w1104) -> (0:w1112:string)  [unwired: 2 in]
                                n573 = Number To Engineering String(2:w1123, 4:w1107) -> (0:w1111:string)  [unwired: 2 in]
                                n574 = Concatenate Strings(w1112, w1108, w1111, w1108, w1110, w1108, w1109, w1108) -> (w1113:string)
                                n575 = Write to Text File(file (use dialog)=w1119, text=w1113, error in=w1120) -> (refnum out=w1115:refnum<file>, error out=w1114:errorcluster)  [unwired: 1 in, 1 out]
                                n576 = Close File(refnum=w1115, error in=w1114) -> (error out=w1122:errorcluster)  [unwired: 1 out]
                                n577 = call <vilib>:"Simple Error Handler.vi"("error in (no error)"=w1122) -> ()  [unwired: 1 in, 8 out]
                                "Z-1K-L" <- w1124
                              }
                              frame #14 {
                                w1134 = "\t"
                                w1149 = i16 4 ("width (-)")
                                n578 = property on="Time RLC" class="DigNum (strict)"() -> ("Value"=w1128:u32)  [unwired: 2 in, 2 out]
                                n579 = Wait (ms)(milliseconds to wait=w1128) -> ()  [unwired: 1 out]
                                n580 = Open/Create/Replace File(file path (use dialog)=w1127, operation (0:open)=T2."open") -> (refnum out=w1143:refnum<file>, error out=w1142:errorcluster)  [unwired: 2 in, 3 out]
                                n581 = Set File Position(refnum=w1143, from (0:start)=enum16{"start", "end", "current"}."end", error in=w1142) -> (refnum out=w1145:refnum<file>, error out=w1146:errorcluster)  [unwired: 1 in]
                                n582 = call "RLC_read.vi"("Path"=w1129, "String"="cmd /c rlc_read_ZCN.py") -> ("MEASURE A"=w1130:dbl, "MEASURE V [V]"=w1132:dbl, "concatenated string"=w1151:string, "MEASURE B"=w1133:dbl, "MEASURE I [A]"=w1131:dbl)  [unwired: 1 out]
                                "MEASURE A 14" <- w1130
                                "MEASURE B 14" <- w1133
                                n583 = Number To Engineering String(2:w1149, 4:w1131) -> (0:w1135:string)  [unwired: 2 in]
                                n584 = local write "RLC300 - digimess"(w1151) -> ()
                                n585 = Number To Engineering String(2:w1149, 4:w1132) -> (0:w1136:string)  [unwired: 2 in]
                                n586 = Number To Engineering String(2:w1149, 4:w1130) -> (0:w1138:string)  [unwired: 2 in]
                                n587 = Number To Engineering String(2:w1149, 4:w1133) -> (0:w1137:string)  [unwired: 2 in]
                                n588 = Concatenate Strings(w1138, w1134, w1137, w1134, w1136, w1134, w1135, w1134) -> (w1139:string)
                                n589 = Write to Text File(file (use dialog)=w1145, text=w1139, error in=w1146) -> (refnum out=w1141:refnum<file>, error out=w1140:errorcluster)  [unwired: 1 in, 1 out]
                                n590 = Close File(refnum=w1141, error in=w1140) -> (error out=w1148:errorcluster)  [unwired: 1 out]
                                n591 = call <vilib>:"Simple Error Handler.vi"("error in (no error)"=w1148) -> ()  [unwired: 1 in, 8 out]
                                "Z-1K-N" <- w1150
                              }
                              frame #15 {
                                w1160 = "\t"
                                w1175 = i16 4 ("width (-)")
                                n592 = property on="Time RLC" class="DigNum (strict)"() -> ("Value"=w1154:u32)  [unwired: 2 in, 2 out]
                                n593 = Wait (ms)(milliseconds to wait=w1154) -> ()  [unwired: 1 out]
                                n594 = Open/Create/Replace File(file path (use dialog)=w1153, operation (0:open)=T2."open") -> (refnum out=w1169:refnum<file>, error out=w1168:errorcluster)  [unwired: 2 in, 3 out]
                                n595 = Set File Position(refnum=w1169, from (0:start)=enum16{"start", "end", "current"}."end", error in=w1168) -> (refnum out=w1171:refnum<file>, error out=w1172:errorcluster)  [unwired: 1 in]
                                n596 = call "RLC_read.vi"("Path"=w1155, "String"="cmd /c rlc_read_ZDL.py") -> ("MEASURE A"=w1156:dbl, "MEASURE V [V]"=w1158:dbl, "concatenated string"=w1177:string, "MEASURE B"=w1159:dbl, "MEASURE I [A]"=w1157:dbl)  [unwired: 1 out]
                                "MEASURE A 15" <- w1156
                                "MEASURE B 15" <- w1159
                                n597 = Number To Engineering String(2:w1175, 4:w1157) -> (0:w1161:string)  [unwired: 2 in]
                                n598 = local write "RLC300 - digimess"(w1177) -> ()
                                n599 = Number To Engineering String(2:w1175, 4:w1158) -> (0:w1162:string)  [unwired: 2 in]
                                n600 = Number To Engineering String(2:w1175, 4:w1156) -> (0:w1164:string)  [unwired: 2 in]
                                n601 = Number To Engineering String(2:w1175, 4:w1159) -> (0:w1163:string)  [unwired: 2 in]
                                n602 = Concatenate Strings(w1164, w1160, w1163, w1160, w1162, w1160, w1161, w1160) -> (w1165:string)
                                n603 = Write to Text File(file (use dialog)=w1171, text=w1165, error in=w1172) -> (refnum out=w1167:refnum<file>, error out=w1166:errorcluster)  [unwired: 1 in, 1 out]
                                n604 = Close File(refnum=w1167, error in=w1166) -> (error out=w1174:errorcluster)  [unwired: 1 out]
                                n605 = call <vilib>:"Simple Error Handler.vi"("error in (no error)"=w1174) -> ()  [unwired: 1 in, 8 out]
                                "Z-10K-L" <- w1176
                              }
                              frame #16 {
                                w1187 = "\t"
                                w1202 = i16 4 ("width (-)")
                                n606 = property on="Time RLC" class="DigNum (strict)"() -> ("Value"=w1180:u32)  [unwired: 2 in, 2 out]
                                n607 = Wait (ms)(milliseconds to wait=w1180) -> ()  [unwired: 1 out]
                                n608 = Open/Create/Replace File(file path (use dialog)=w1179, operation (0:open)=T2."open") -> (refnum out=w1196:refnum<file>, error out=w1195:errorcluster)  [unwired: 2 in, 3 out]
                                n609 = Set File Position(refnum=w1196, from (0:start)=enum16{"start", "end", "current"}."end", error in=w1195) -> (refnum out=w1198:refnum<file>, error out=w1199:errorcluster)  [unwired: 1 in]
                                n610 = call "RLC_read.vi"("Path"=w1181, "String"="cmd /c rlc_read_ZDN.py") -> ("MEASURE A"=w1182:dbl, "MEASURE V [V]"=w1185:dbl, "concatenated string"=w1204:string, "MEASURE B"=w1186:dbl, "MEASURE I [A]"=w1184:dbl)  [unwired: 1 out]
                                "MEASURE A 16" <- w1182
                                "MEASURE B 16" <- w1186
                                n611 = Number To Engineering String(2:w1202, 4:w1184) -> (0:w1188:string)  [unwired: 2 in]
                                n612 = local write "RLC300 - digimess"(w1204) -> ()
                                n613 = Number To Engineering String(2:w1202, 4:w1185) -> (0:w1189:string)  [unwired: 2 in]
                                n614 = Number To Engineering String(2:w1202, 4:w1182) -> (0:w1191:string)  [unwired: 2 in]
                                n615 = Number To Engineering String(2:w1202, 4:w1186) -> (0:w1190:string)  [unwired: 2 in]
                                n616 = Concatenate Strings(w1191, w1187, w1190, w1187, w1189, w1187, w1188, w1187, "\r\n") -> (w1192:string)
                                n617 = Write to Text File(file (use dialog)=w1198, text=w1192, error in=w1199) -> (refnum out=w1194:refnum<file>, error out=w1193:errorcluster)  [unwired: 1 in, 1 out]
                                n618 = Close File(refnum=w1194, error in=w1193) -> (error out=w1201:errorcluster)  [unwired: 1 out]
                                n619 = call <vilib>:"Simple Error Handler.vi"("error in (no error)"=w1201) -> ()  [unwired: 1 in, 8 out]
                                "Z-10K-N" <- w1203
                              }
                              frame #17 {
                                n620 = local write "Z-50-L"(w1207) -> ()
                                n621 = local write "Z-1K-L"(w1207) -> ()
                                n622 = local write "Z-1K-N"(w1207) -> ()
                                n623 = local write "C-50-N"(w1207) -> ()
                                n624 = local write "C-50-L"(w1207) -> ()
                                n625 = local write "Z-50-N"(w1207) -> ()
                                n626 = local write "C-1K-N"(w1207) -> ()
                                n627 = local write "C-1K-L"(w1207) -> ()
                                n628 = local write "Z-100-L"(w1207) -> ()
                                n629 = local write "Z-100-N"(w1207) -> ()
                                n630 = local write "Z-10K-L"(w1207) -> ()
                                n631 = local write "Z-10K-N"(w1207) -> ()
                                n632 = local write "C-10K-N"(w1207) -> ()
                                n633 = local write "C-10K-L"(w1207) -> ()
                                n634 = local write "C-100-N"(w1207) -> ()
                                n635 = local write "C-100-L"(w1207) -> ()
                              }
                            }
                          }
                          n636 = call <vilib>:"Mean.vi"("X"=w738) -> ("mean"=w720:dbl)  [unwired: 1 out]
                          "mean 2" <- w720
                          n637 = call <vilib>:"Mean.vi"("X"=w737) -> ("mean"=w719:dbl)  [unwired: 1 out]
                          "mean 3" <- w719
                          n638 = call <vilib>:"Mean.vi"("X"=w736) -> ("mean"=w718:dbl)  [unwired: 1 out]
                          "mean 4" <- w718
                          n639 = call <vilib>:"Mean.vi"("X"=w735) -> ("mean"=w717:dbl)  [unwired: 1 out]
                          "mean 5" <- w717
                          n640 = call <vilib>:"Mean.vi"("X"=w734) -> ("mean"=w716:dbl)  [unwired: 1 out]
                          "mean 6" <- w716
                          n641 = call <vilib>:"Mean.vi"("X"=w733) -> ("mean"=w715:dbl)  [unwired: 1 out]
                          "mean 7" <- w715
                          n642 = call <vilib>:"Mean.vi"("X"=w732) -> ("mean"=w714:dbl)  [unwired: 1 out]
                          "mean 8" <- w714
                          n643 = call <vilib>:"Mean.vi"("X"=w731) -> ("mean"=w713:dbl)  [unwired: 1 out]
                          "mean 9" <- w713
                          n644 = call <vilib>:"Mean.vi"("X"=w730) -> ("mean"=w712:dbl)  [unwired: 1 out]
                          "mean 10" <- w712
                          n645 = call <vilib>:"Mean.vi"("X"=w729) -> ("mean"=w711:dbl)  [unwired: 1 out]
                          "mean 11" <- w711
                          n646 = call <vilib>:"Mean.vi"("X"=w728) -> ("mean"=w710:dbl)  [unwired: 1 out]
                          "mean 12" <- w710
                          n647 = call <vilib>:"Mean.vi"("X"=w727) -> ("mean"=w709:dbl)  [unwired: 1 out]
                          "mean 13" <- w709
                          n648 = call <vilib>:"Mean.vi"("X"=w726) -> ("mean"=w708:dbl)  [unwired: 1 out]
                          "mean 14" <- w708
                          n649 = call <vilib>:"Mean.vi"("X"=w725) -> ("mean"=w707:dbl)  [unwired: 1 out]
                          "mean 15" <- w707
                          n650 = call <vilib>:"Mean.vi"("X"=w739) -> ("mean"=w721:dbl)  [unwired: 1 out]
                          "mean" <- w721
                          n651 = call <vilib>:"Mean.vi"("X"=w724) -> ("mean"=w706:dbl)  [unwired: 1 out]
                          "mean 16" <- w706
                        }
                      }
                    }
                    frame #2 {
                      n652 = case shown="True" w1208 {
                        tunnel: w1225 -> [_ w1241]
                        tunnel: w1224 -> [_ w1240]
                        tunnel: w1223 -> [_ w1239]
                        tunnel: w1222 -> [_ w1238]
                        tunnel: w1221 -> [_ w1237]
                        tunnel: w1220 -> [_ w1236]
                        tunnel: w1219 -> [_ w1235]
                        tunnel: w1218 -> [_ w1234]
                        tunnel: w1217 -> [_ w1233]
                        tunnel: w1216 -> [_ w1232]
                        tunnel: w1215 -> [_ w1231]
                        tunnel: w1214 -> [_ w1230]
                        tunnel: w1213 -> [_ w1229]
                        tunnel: w1212 -> [_ w1228]
                        tunnel: w1211 -> [_ w1227]
                        tunnel: w1210 -> [_ w1226]
                        frame False {
                        }
                        frame True {
                          w1255 = "\t"
                          w1272 = i16 4 ("precision (6)")
                          n653 = property on="SET" class="DigNum (strict)"() -> ("Value"=w1273:i32)  [unwired: 2 in, 2 out]
                          n654 = Number To Engineering String(2:w1272, 4:w1226) -> (0:w1269:string)  [unwired: 2 in]
                          n655 = Number To Engineering String(2:w1272, 4:w1240) -> (0:w1268:string)  [unwired: 2 in]
                          n656 = Number To Engineering String(2:w1272, 4:w1239) -> (0:w1267:string)  [unwired: 2 in]
                          n657 = Number To Engineering String(2:w1272, 4:w1238) -> (0:w1266:string)  [unwired: 2 in]
                          n658 = Number To Engineering String(2:w1272, 4:w1237) -> (0:w1265:string)  [unwired: 2 in]
                          n659 = Number To Engineering String(2:w1272, 4:w1236) -> (0:w1264:string)  [unwired: 2 in]
                          n660 = Number To Engineering String(2:w1272, 4:w1235) -> (0:w1263:string)  [unwired: 2 in]
                          n661 = Number To Engineering String(2:w1272, 4:w1234) -> (0:w1262:string)  [unwired: 2 in]
                          n662 = Number To Engineering String(2:w1272, 4:w1233) -> (0:w1261:string)  [unwired: 2 in]
                          n663 = Number To Engineering String(2:w1272, 4:w1232) -> (0:w1260:string)  [unwired: 2 in]
                          n664 = Number To Engineering String(2:w1272, 4:w1231) -> (0:w1259:string)  [unwired: 2 in]
                          n665 = Number To Engineering String(2:w1272, 4:w1230) -> (0:w1258:string)  [unwired: 2 in]
                          n666 = Number To Engineering String(2:w1272, 4:w1229) -> (0:w1257:string)  [unwired: 2 in]
                          n667 = Number To Engineering String(2:w1272, 4:w1228) -> (0:w1256:string)  [unwired: 2 in]
                          n668 = Number To Engineering String(2:w1272, 4:w1241) -> (0:w1270:string)  [unwired: 2 in]
                          n669 = Number To Engineering String(2:w1272, 4:w1227) -> (0:w1254:string)  [unwired: 2 in]
                          n670 = Number To Decimal String(number=w1273) -> (decimal integer string=w1271:string)  [unwired: 1 in]
                          n671 = property on="path RLC_mean" class="Path"() -> ("Value"=w1242:path)  [unwired: 2 in, 2 out]
                          n672 = Open/Create/Replace File(file path (use dialog)=w1242, operation (0:open)=T2."open") -> (refnum out=w1247:refnum<file>, error out=w1246:errorcluster)  [unwired: 2 in, 3 out]
                          n673 = Concatenate Strings(w1271, w1255, w1270, w1255, w1269, w1255, w1268, w1255, w1267, w1255, w1266, w1255, w1265, w1255, w1264, w1255, w1263, w1255, w1262, w1255, w1261, w1255, w1260, w1255, w1259, w1255, w1258, w1255, w1257, w1255, w1256, w1255, w1254, "\r\n") -> (w1243:string)
                          n674 = Set File Position(refnum=w1247, from (0:start)=enum16{"start", "end", "current"}."end", error in=w1246) -> (refnum out=w1249:refnum<file>, error out=w1250:errorcluster)  [unwired: 1 in]
                          n675 = Write to Text File(file (use dialog)=w1249, text=w1243, error in=w1250) -> (refnum out=w1245:refnum<file>, error out=w1244:errorcluster)  [unwired: 1 in, 1 out]
                          n676 = Close File(refnum=w1245, error in=w1244) -> (error out=w1252:errorcluster)  [unwired: 1 out]
                          n677 = call <vilib>:"Simple Error Handler.vi"("error in (no error)"=w1252) -> ()  [unwired: 1 in, 8 out]
                        }
                      }
                    }
                  }
                  n678 = local write "graph RLC"(w656) -> ()
                }
                frame 9 {
                  n679 = flat-sequence {
                    tunnel: w1312 -> [w1323]
                    tunnel: [w1323] -> w1311
                    tunnel: [w1317] -> w1310
                    tunnel: [w1316] -> w1309
                    tunnel: w1311 -> [w1348]
                    tunnel: w1310 -> [_]
                    tunnel: w1309 -> [w1345]
                    frame #0 {
                      n680 = property on="SET" class="DigNum (strict)"() -> ("Value"=w1321:i32)  [unwired: 2 in, 2 out]
                      n681 = Increment(x=w1321) -> (x+1=w1316:i32)
                      n682 = property on="P_max camara" class="DigNum (strict)"() -> ("Value"=w1314:dbl)  [unwired: 2 in, 2 out]
                      n683 = local write "SET"(w1316) -> ()
                      n684 = property on="Camara 2" class="Slide (strict)"() -> ("Value"=w1315:dbl)  [unwired: 2 in, 2 out]
                      n685 = case shown="False" "Boolean" {
                        selector: "Boolean" -> [w1329 w1334]
                        tunnel: [w1331 w1338] -> w1318
                        tunnel: w1316 -> [w1332 _]
                        frame False {
                          n686 = local write "Boolean 2"(w1329) -> ()
                          n687 = Index Array(array="Array", index=w1332) -> (element=w1331:dbl)
                          n688 = Not(x=w1329) -> (.not. x?=→"Boolean 3":bool)
                        }
                        frame True {
                          n689 = property on="Set P auto" class="DigNum (strict)"() -> ("Value"=w1336:dbl)  [unwired: 2 in, 2 out]
                          n690 = Add(x="Step P", y=w1336) -> (x+y=w1338:dbl)
                          n691 = Not(x=w1334) -> (.not. x?=w1335:bool)
                          n692 = local write "Boolean 3"(w1335) -> ()
                          "Boolean 2" <- w1334
                        }
                      }
                      n693 = Greater?(x=w1315, y=w1314) -> (0:w1313:bool)
                      n694 = case shown="True" w1313 {
                        frame False {
                        }
                        frame True {
                          n695 = property on="Desc SET" class="DigNum (strict)"() -> ("Value"=w1325:i32)  [unwired: 2 in, 2 out]
                          n696 = local write "Descarga"(TRUE ("Descarga")) -> ()
                          n697 = Increment(x=w1325) -> (x+1=w1324:i32)
                          n698 = local write "Desc SET"(w1324) -> ()
                        }
                      }
                      n699 = Greater?(x=w1318, y="P_max") -> (0:w1320:bool)
                      n700 = case shown="True" w1320 {
                        tunnel: [w1327 w1328] -> w1317
                        tunnel: "P_max" -> [_ w1328]
                        tunnel: w1318 -> [w1327 _]
                        frame False {
                        }
                        frame True {
                        }
                      }
                      n701 = local write "Set P auto"(w1317) -> ()
                    }
                    frame #1 {
                      n702 = property on="Desc SET" class="DigNum (strict)"() -> ("Value"=w1340:i32)  [unwired: 2 in, 2 out]
                      n703 = Quotient & Remainder(x=w1345, y="Step ZPit") -> (x-y*floor(x/y)=w1346:dbl)  [unwired: 1 out]
                      n704 = Greater Than 0?(x=w1340) -> (x > 0?=w1342:bool)
                      n705 = Equal To 0?(x=w1346) -> (x = 0?=w1344:bool)
                      "Read ZPit" <- w1344
                      n706 = property on="Descarga" class="Bool (strict)"() -> ("Value"=w1339:bool)  [unwired: 2 in, 2 out]
                      n707 = And(x=w1342, y=w1339) -> (x .and. y?=w1341:bool)
                      n708 = case shown="True" w1341 {
                        tunnel: w1344 -> [w1349 _]
                        tunnel: [w1349 w1350] -> w1343
                        frame False {
                        }
                        frame True {
                          w1350 = TRUE
                          n709 = local write "Read ZPit"(w1350) -> ()
                        }
                      }
                      n710 = case shown="True" w1343 {
                        tunnel: w1348 -> [_ w1352]
                        frame False {
                          n711 = local write "Estagio auto"(11 ("Estagio auto")) -> ()
                        }
                        frame True {
                          n712 = Greater?(x=w1352, y=1.0) -> (0:w1357:bool)
                          n713 = case shown="False" w1357 {
                            tunnel: [FALSE ("Boolean") TRUE ("Boolean")] -> w1355
                            frame False {
                              w1377 = TRUE ("Boolean")
                              n714 = local write "Vácuo 2"(w1377) -> ()
                              n715 = Multiply(x="ZPf2 time", y=0.0741) -> (x*y=w1372:dbl)
                              n716 = local write "String"("Limpar volume referencia" ("String")) -> ()
                              n717 = Add(x=w1372, y=1.9801) -> (x+y=w1370:dbl)
                              n718 = call "Controle_vacuo.vi"("time (s) to wait vacuo"=w1370, "Boolean"=w1377) -> ("Vacuo"=w1378:bool)  [unwired: 9 in]
                              n719 = local write "Vácuo 2"(w1378) -> ()
                            }
                            frame True {
                              n720 = property on="ATM wait" class="DigNum (strict)"() -> ("Value"=w1379:u32)  [unwired: 2 in, 2 out]
                              n721 = call "Controle_ATM.vi"("seconds to wait"=w1379) -> ("String 2"=w1382:string, "Atm"=w1381:bool)  [unwired: 9 in]
                              n722 = local write "Atm 2"(w1381) -> ()
                              n723 = local write "String"(w1382) -> ()
                            }
                          }
                          n724 = for {
                            N: 1 -> [_]
                            tunnel: [w1359] -> w1354
                            tunnel: w1355 -> [w1359]
                            n725 = Wait (ms)(milliseconds to wait=u32 500 ("x")) -> ()  [unwired: 1 out]
                          }
                          n726 = case shown="True" w1354 {
                            frame False {
                              n727 = local write "Estagio auto"(10 ("Estagio auto")) -> ()
                            }
                            frame True {
                              w1368 = TRUE ("Boolean")
                              n728 = property on="ZPf2 time" class="DigNum (strict)"() -> ("Value"=w1362:dbl)  [unwired: 2 in, 2 out]
                              n729 = local write "Estagio auto"(10 ("Estagio auto")) -> ()
                              n730 = Multiply(x=w1362, y=0.0741) -> (x*y=w1364:dbl)
                              n731 = local write "Vácuo 2"(w1368) -> ()
                              n732 = local write "String"("Limpar volume referencia" ("String")) -> ()
                              n733 = Add(x=w1364, y=1.9801) -> (x+y=w1361:dbl)
                              n734 = call "Controle_vacuo.vi"("time (s) to wait vacuo"=w1361, "Boolean"=w1368) -> ("Vacuo"=w1369:bool)  [unwired: 9 in]
                              n735 = local write "Vácuo 2"(w1369) -> ()
                            }
                          }
                        }
                      }
                    }
                  }
                }
                frame 10 {
                  n736 = property on="Contador" class="DigNum (strict)"() -> ("Value"=w1383:i32)  [unwired: 2 in, 2 out]
                  n737 = Increment(x=w1383) -> (x+1=w1386:i32)
                  n738 = local write "String"("Ler ZPf2 e T" ("String")) -> ()
                  n739 = Equal?(x=w1386, y=100) -> (x = y?=w1384:bool)
                  n740 = case shown="True" w1384 {
                    frame False {
                    }
                    frame True {
                      n741 = local write "Estagio auto"(11 ("Estagio auto")) -> ()
                    }
                  }
                }
                frame 11 {
                  n742 = property on="Contador" class="DigNum (strict)"() -> ("Value"=w1391:i32)  [unwired: 2 in, 2 out]
                  n743 = Increment(x=w1391) -> (x+1=w1393:i32)
                  n744 = Equal?(x=w1393, y=100) -> (x = y?=w1390:bool)
                  n745 = case shown="True" w1390 {
                    tunnel: w1394 -> [_ w1405]
                    tunnel: w1389 -> [_ w1395]
                    frame False {
                    }
                    frame True {
                      w1396 = i16 3 ("precision (6)")
                      w1399 = "\t"
                      n746 = property on="Read ZPit" class="Bool (strict)"() -> ("Value"=w1400:bool)  [unwired: 2 in, 2 out]
                      n747 = property on="T fit" class="DigNum (strict)"() -> ("Value"=w1401:dbl)  [unwired: 2 in, 2 out]
                      n748 = case shown="False" w1400 {
                        tunnel: ["  ==>" w1411] -> w1404
                        tunnel: w1396 -> [_ w1410]
                        frame False {
                        }
                        frame True {
                          n749 = property on="P fit" class="DigNum (strict)"() -> ("Value"=w1409:dbl)  [unwired: 2 in, 2 out]
                          n750 = Number To Fractional String(number=w1409, precision (6)=w1410) -> (F-format string=w1411:string)  [unwired: 2 in]
                        }
                      }
                      n751 = Number To Fractional String(number=w1401, precision (6)=w1396) -> (F-format string=w1403:string)  [unwired: 2 in]
                      n752 = Number To Fractional String(number=w1395, precision (6)=w1396) -> (F-format string=w1398:string)  [unwired: 2 in]
                      n753 = Concatenate Strings(w1404, w1399, w1403, w1399, w1398, "\r\n") -> (w1402:string)
                      n754 = flat-sequence {
                        tunnel: [w1415] -> w1407
                        tunnel: [w1414] -> w1406
                        tunnel: w1402 -> [w1413]
                        tunnel: w1405 -> [w1412]
                        tunnel: w1407 -> [w1429]
                        tunnel: w1406 -> [w1428]
                        frame #0 {
                          n755 = Open/Create/Replace File(file path (use dialog)=w1412, operation (0:open)=T2."open") -> (refnum out=w1421:refnum<file>, error out=w1422:errorcluster)  [unwired: 2 in, 3 out]
                          n756 = Set File Position(refnum=w1421, from (0:start)=enum16{"start", "end", "current"}."end", error in=w1422) -> (refnum out=w1419:refnum<file>, error out=w1418:errorcluster)  [unwired: 1 in]
                          n757 = Write to Text File(file (use dialog)=w1419, text=w1413, error in=w1418) -> (refnum out=w1423:refnum<file>, error out=w1424:errorcluster)  [unwired: 2 out]
                          n758 = Close File(refnum=w1423, error in=w1424) -> (path=w1415:path, error out=w1416:errorcluster)
                          n759 = call <vilib>:"Simple Error Handler.vi"("error in (no error)"=w1416) -> ("error out"=w1414:errorcluster)  [unwired: 1 in, 7 out]
                        }
                        frame #1 {
                          w1425 = TRUE ("ZPit")
                          n760 = Wait (ms)(milliseconds to wait=u32 500) -> ()  [unwired: 1 out]
                          n761 = local write "T 2"(w1425) -> ()
                          n762 = local write "ZPf2 2"(w1425) -> ()
                          n763 = Read from Text File(file (use dialog)=w1429, count=-1 ("Count  3"), error in=w1428) -> (refnum out=w1430:refnum<file>, text=w1434:string, error out=w1431:errorcluster)  [unwired: 1 in, 1 out]
                          n764 = local write "String 3"(w1434) -> ()
                          n765 = Close File(refnum=w1430, error in=w1431) -> (error out=w1432:errorcluster)  [unwired: 1 out]
                          n766 = local write "String"("abrir valvula entrada gas" ("String")) -> ()
                          n767 = call <vilib>:"Simple Error Handler.vi"("error in (no error)"=w1432) -> ()  [unwired: 1 in, 8 out]
                        }
                        frame #2 {
                          n768 = property on="Desc SET" class="DigNum (strict)"() -> ("Value"=w1436:i32)  [unwired: 2 in, 2 out]
                          n769 = Greater Than 0?(x=w1436) -> (x > 0?=w1435:bool)
                          n770 = property on="Camara 2" class="Slide (strict)"() -> ("Value"=w1443:dbl)  [unwired: 2 in, 2 out]
                          n771 = Greater?(x=w1443, y="P_max camara") -> (0:w1441:bool)
                          n772 = property on="Carga" class="Bool (strict)"() -> ("Value"=w1440:bool)  [unwired: 2 in, 2 out]
                          n773 = And(x=w1441, y=w1440) -> (x .and. y?=w1438:bool)
                          n774 = case shown="False" w1435 {
                            tunnel: w1438 -> [w1444 _]
                            tunnel: [w1444 TRUE] -> w1437
                            frame False {
                            }
                            frame True {
                            }
                          }
                          n775 = case shown="False" w1437 {
                            tunnel: [5 ("N fit") 100 ("N fit")] -> w1439
                            frame False {
                              n776 = local write "Estagio auto"(0 ("Estagio auto")) -> ()
                              "Carga" <- TRUE
                              "Descarga" <- FALSE
                            }
                            frame True {
                              n777 = local write "teste slope"(0 ("teste slope")) -> ()
                              n778 = local write "Carga"(FALSE ("Carga")) -> ()
                              n779 = local write "Descarga"(TRUE ("Descarga")) -> ()
                              n780 = local write "Estagio auto"(12 ("Estagio auto")) -> ()
                            }
                          }
                          n781 = local write "N fit"(w1439) -> ()
                        }
                      }
                    }
                  }
                }
                frame 12 {
                  w1460 = "\t"
                  n782 = property on="SET" class="DigNum (strict)"() -> ("Value"=w1464:i32)  [unwired: 2 in, 2 out]
                  n783 = Number To Decimal String(number=w1464) -> (decimal integer string=w1467:string)  [unwired: 1 in]
                  n784 = Number To Fractional String(number=0.0, precision (6)=i16 3) -> (F-format string=w1461:string)  [unwired: 2 in]
                  n785 = Concatenate Strings(w1467, w1460, w1461, w1460, w1461, w1460) -> (w1466:string)
                  n786 = flat-sequence {
                    tunnel: w1463 -> [w1472]
                    tunnel: w1466 -> [w1473]
                    tunnel: [w1473] -> w1459
                    tunnel: [w1472] -> w1458
                    tunnel: [w1477] -> w1469
                    tunnel: [w1476] -> w1468
                    tunnel: w1459 -> [w1475]
                    tunnel: w1458 -> [w1474]
                    tunnel: [w1474] -> w1457
                    tunnel: w1469 -> [w1493]
                    tunnel: w1468 -> [w1492]
                    tunnel: w1457 -> [w1487]
                    tunnel: [w1487] -> w1456
                    tunnel: w1456 -> [w1501]
                    tunnel: [w1500] -> w1455
                    tunnel: w1455 -> [w1538]
                    frame #0 {
                      w1471 = FALSE ("ZPit 2")
                      n787 = Wait (ms)(milliseconds to wait=u32 1000) -> ()  [unwired: 1 out]
                      n788 = local write "ZPit 2"(w1471) -> ()
                      n789 = local write "Pit 2"(w1471) -> ()
                      n790 = local write "Pf2 2"(w1471) -> ()
                      n791 = local write "ZPf2 2"(w1471) -> ()
                      n792 = local write "T 2"(w1471) -> ()
                    }
                    frame #1 {
                      n793 = Open/Create/Replace File(file path (use dialog)=w1474, operation (0:open)=T2."open") -> (refnum out=w1483:refnum<file>, error out=w1484:errorcluster)  [unwired: 2 in, 3 out]
                      n794 = Set File Position(refnum=w1483, from (0:start)=enum16{"start", "end", "current"}."end", error in=w1484) -> (refnum out=w1481:refnum<file>, error out=w1480:errorcluster)  [unwired: 1 in]
                      n795 = Write to Text File(file (use dialog)=w1481, text=w1475, error in=w1480) -> (refnum out=w1485:refnum<file>, error out=w1486:errorcluster)  [unwired: 2 out]
                      n796 = Close File(refnum=w1485, error in=w1486) -> (path=w1477:path, error out=w1478:errorcluster)
                      n797 = call <vilib>:"Simple Error Handler.vi"("error in (no error)"=w1478) -> ("error out"=w1476:errorcluster)  [unwired: 1 in, 7 out]
                    }
                    frame #2 {
                      w1488 = TRUE ("ZPit")
                      n798 = local write "Estagio auto"(7 ("Estagio auto")) -> ()
                      n799 = Wait (ms)(milliseconds to wait=u32 500) -> ()  [unwired: 1 out]
                      n800 = local write "ZPit 2"(w1488) -> ()
                      n801 = local write "Pit 2"(w1488) -> ()
                      n802 = Read from Text File(file (use dialog)=w1493, count=-1 ("Count  3"), error in=w1492) -> (refnum out=w1494:refnum<file>, text=w1498:string, error out=w1495:errorcluster)  [unwired: 1 in, 1 out]
                      n803 = local write "String 3"(w1498) -> ()
                      n804 = Close File(refnum=w1494, error in=w1495) -> (error out=w1496:errorcluster)  [unwired: 1 out]
                      n805 = call <vilib>:"Simple Error Handler.vi"("error in (no error)"=w1496) -> ()  [unwired: 1 in, 8 out]
                      n806 = local write "String"("abrir valvula camara" ("String")) -> ()
                    }
                    frame #3 {
                      n807 = property on="Camara 2" class="Slide (strict)"() -> ("Value"=w1504:dbl)  [unwired: 2 in, 2 out]
                      n808 = Less?(x=w1504, y="P_min descarga") -> (x < y?=w1499:bool)
                      n809 = property on="Efetuados" class="DigNum (strict)"() -> ("Value"=w1502:dbl)  [unwired: 2 in, 2 out]
                      n810 = case shown="True" w1499 {
                        tunnel: w1502 -> [_ w1533]
                        tunnel: w1501 -> [_ w1522]
                        tunnel: [TRUE ("data") FALSE ("data")] -> w1500
                        tunnel: w1499 -> [_ w1511]
                        frame False {
                          n811 = property on="Desc SET" class="DigNum (strict)"() -> ("Value"=w1506:i32)  [unwired: 2 in, 2 out]
                          n812 = Increment(x=w1506) -> (x+1=→"Desc SET":i32)
                        }
                        frame True {
                          w1520 = "\r\n"
                          n813 = Increment(x=w1533) -> (x+1=w1508:dbl)
                          "Efetuados" <- w1508
                          n814 = local write "Estagio auto"(0 ("Estagio auto")) -> ()
                          n815 = local write "SET"(0 ("SET")) -> ()
                          n816 = local write "Desc SET"(0 ("Desc SET")) -> ()
                          n817 = local write "Descarga"(FALSE ("Descarga")) -> ()
                          n818 = local write "Carga"(TRUE ("Carga")) -> ()
                          n819 = local write "Set P auto"(0.5 ("Set P auto")) -> ()
                          n820 = Open/Create/Replace File(file path (use dialog)=w1522, operation (0:open)=T2."open") -> (refnum out=w1528:refnum<file>, error out=w1529:errorcluster)  [unwired: 2 in, 3 out]
                          n821 = Less Or Equal?(x="Ciclos", y=w1508) -> (x <= y?=w1509:bool)
                          n822 = And(x=w1511, y=w1509) -> (x .and. y?=w1512:bool)
                          n823 = Set File Position(refnum=w1528, from (0:start)=enum16{"start", "end", "current"}."end", error in=w1529) -> (refnum out=w1526:refnum<file>, error out=w1525:errorcluster)  [unwired: 1 in]
                          n824 = case shown="False" w1512 {
                            frame False {
                              n825 = local write "FIM"(FALSE ("FIM")) -> ()
                            }
                            frame True {
                              w1537 = 1 ("N fit")
                              n826 = local write "Auto Ctrl"(FALSE ("Auto Ctrl")) -> ()
                              n827 = local write "N fit"(w1537) -> ()
                              n828 = local write "N to fit"(w1537) -> ()
                              "FIM" <- TRUE ("stop")
                            }
                          }
                          n829 = Concatenate Strings(w1520, ">>>>>>>>>>>>>>" ("string"), w1520, w1520) -> (w1519:string)
                          n830 = Write to Text File(file (use dialog)=w1526, text=w1519, error in=w1525) -> (refnum out=w1530:refnum<file>, error out=w1531:errorcluster)  [unwired: 2 out]
                          n831 = Close File(refnum=w1530, error in=w1531) -> (error out=w1523:errorcluster)  [unwired: 1 out]
                          n832 = call <vilib>:"Simple Error Handler.vi"("error in (no error)"=w1523) -> ()  [unwired: 1 in, 8 out]
                        }
                      }
                    }
                    frame #4 {
                      w1540 = T5 3 items=["no dialog", "OK message", "continue or stop message", "OK message + warnings", "continue/stop + warnings"] ("type of dialog (OK msg:1)")
                      n833 = local write "Câmara 2"(w1538) -> ()
                      n834 = call-poly <vilib>:"DAQmx Create Virtual Channel.vi"("lines"=tag "Dev1/port0/line3") -> ("task out"=w1549:refnum<k21>, "error out"=w1548:errorcluster)  [unwired: 13 in]
                      n835 = call <vilib>:"DAQmx Start Task.vi"("task/channels in"=w1549, "error in"=w1548) -> ("task out"=w1547:refnum<k21>, "error out"=w1546:errorcluster)  [unwired: 12 in]
                      n836 = call-poly <vilib>:"DAQmx Write.vi"("task/channels in"=w1547, "data"=w1538, "error in"=w1546) -> ("task out"=w1542:refnum<k21>, "error out"=w1541:errorcluster)  [unwired: 10 in, 1 out]
                      n837 = call <vilib>:"DAQmx Stop Task.vi"("task/channels in"=w1542, "error in"=w1541) -> ("task out"=w1544:refnum<k21>, "error out"=w1545:errorcluster)  [unwired: 12 in]
                      n838 = call <vilib>:"DAQmx Clear Task.vi"("task in"=w1544, "error in"=w1545) -> ("error out"=w1539:errorcluster)  [unwired: 13 in]
                      n839 = call <vilib>:"Simple Error Handler.vi"("type of dialog (OK msg:1)"=w1540, "error in (no error)"=w1539) -> ()  [unwired: 3 in, 5 out]
                    }
                  }
                }
              }
            }
          }
          n840 = Index Array(array=w258, index=w256) -> (element=w255:dbl)
          n841 = Index Array(array=w257, index=w256) -> (element=w254:dbl)
          n842 = Bundle("Real 2D Array"=w261, "Best Linear Fit"=w273) -> (w272:T6)  [unwired: 1 in]
          n843 = Bundle("Real 2D Array"=w261, "Best Polynomial Fit"=w262) -> (w259:T7)  [unwired: 1 in]
          n844 = Bundle("Real 2D Array"=w261, "Best Polynomial Fit"=w263) -> (w260:T7)  [unwired: 1 in]
          n845 = case shown="True" w253 {
            tunnel: w255 -> [_ w1552]
            tunnel: w254 -> [_ w1551]
            tunnel: w248 -> [_ w1550]
            frame False {
            }
            frame True {
              "P fit" <- w1552
              "T fit" <- w1551
              "P (bar/s)" <- w1550
            }
          }
          n846 = Build Array(w271, w272, w259) -> (→"Linear T":T8)
          n847 = Bundle("Real 2D Array"=w261, "Best Linear Fit"=w268) -> (w269:T6)  [unwired: 1 in]
          n848 = Build Array(w270, w269, w260) -> (→"Linear P":T8)
          "Contador" <- w252
        }
        n849 = local write "P subarray 2"(dbl[] [0.0, 1.0] ("subarray")) -> ()
        n850 = local write "T subarray 3"(dbl[] [0.0, 1.0] ("subarray")) -> ()
        n851 = local write "time subarray"(dbl[] [0.0, 1.0] ("subarray")) -> ()
      }
    }
    n852 = case shown="True" "Manual Ctrl" {
      tunnel: w35 -> [_ w1633]
      tunnel: "RLC on/off" -> [_ w1632]
      tunnel: [FALSE w1635] -> w37
      frame False {
      }
      frame True {
        w1647 = 0 ("polynomial order")
        n853 = for {
          N: "N to fit" -> [_]
          tunnel: [w2316] -> w1622 mode=indexing
          tunnel: [w2321] -> w1640 mode=indexing
          tunnel: [w2321] -> w1626 mode=indexing
          tunnel: [w2312] -> w1631 mode=indexing
          i -> [w2321]
          n854 = case shown="False" "Clear" {
            frame False {
            }
            frame True {
              n855 = property on="P-manual" class="WFChart (strict)"("History Data"=dynamicdata[] []) -> ()  [unwired: 2 in, 2 out]
            }
          }
          n856 = case shown="True" "Câmara" {
            frame False {
            }
            frame True {
              n857 = property on="Vol Ref" class="Slide (strict)"() -> ("Value"=w2369:dbl)  [unwired: 2 in, 2 out]
              n858 = local write "Camara"(w2369) -> ()
            }
          }
          n859 = case shown="True" "Guardar\nCinetica" {
            frame False {
            }
            frame True {
              n860 = feedback #2() -> (w2324:bool)  [unwired: 1 in]
              "x >= y?" <- w2324
              n861 = call "Elapsed Time"("Reset"=w2324) -> ("Elapsed Time (s)"=w2326:dbl)  [unwired: 11 in, 7 out]
              "Elapsed Time (sec)" <- w2326
              n862 = case shown="True" w2324 {
                frame False {
                }
                frame True {
                  n863 = flat-sequence {
                    tunnel: [w2341] -> w2329
                    tunnel: [w2340] -> w2328
                    tunnel: w2329 -> [w2359]
                    tunnel: w2328 -> [w2358]
                    frame #0 {
                      w2334 = "\t"
                      w2331 = i16 4 ("precision (6)")
                      n864 = property on="MEASURE C [F ]" class="DigNum (strict)"() -> ("Value"=w2330:dbl)  [unwired: 2 in, 2 out]
                      n865 = property on="termopar K" class="DigNum (strict)"() -> ("Value"=w2335:dbl)  [unwired: 2 in, 2 out]
                      n866 = Number To Fractional String(number=w2335, precision (6)=w2331) -> (F-format string=w2336:string)  [unwired: 2 in]
                      n867 = property on="P cinetica mean" class="DigNum (strict)"() -> ("Value"=w2338:dbl)  [unwired: 2 in, 2 out]
                      n868 = property on="T cinetica mean 2" class="DigNum (strict)"() -> ("Value"=w2337:dbl)  [unwired: 2 in, 2 out]
                      n869 = property on="path 2_cinetica" class="Path"() -> ("Value"=w2339:path)  [unwired: 2 in, 2 out]
                      n870 = Get Date/Time String(date format (0)=enum16{"short", "long", "abbreviated"}."short", want seconds? (F)=TRUE) -> (date string=w2355:string, time string=w2354:string)  [unwired: 1 in]
                      n871 = Number To Exponential String(number=w2330, precision (6)=w2331) -> (E-format string=w2333:string)  [unwired: 2 in]
                      n872 = Number To Fractional String(number=w2338, precision (6)=w2331) -> (F-format string=w2353:string)  [unwired: 2 in]
                      n873 = Number To Fractional String(number=w2337, precision (6)=w2331) -> (F-format string=w2352:string)  [unwired: 2 in]
                      n874 = Open/Create/Replace File(file path (use dialog)=w2339, operation (0:open)=T2."open") -> (refnum out=w2348:refnum<file>, error out=w2349:errorcluster)  [unwired: 2 in, 3 out]
                      n875 = Concatenate Strings(w2355, w2334, w2354, w2334, w2353, w2334, w2352, w2334, w2336, w2334, w2333, "\r\n") -> (w2342:string)
                      n876 = Set File Position(refnum=w2348, from (0:start)=enum16{"start", "end", "current"}."end", error in=w2349) -> (refnum out=w2346:refnum<file>, error out=w2345:errorcluster)  [unwired: 1 in]
                      n877 = Write to Text File(file (use dialog)=w2346, text=w2342, error in=w2345) -> (refnum out=w2350:refnum<file>, error out=w2351:errorcluster)  [unwired: 2 out]
                      n878 = Close File(refnum=w2350, error in=w2351) -> (path=w2341:path, error out=w2343:errorcluster)
                      n879 = call <vilib>:"Simple Error Handler.vi"("error in (no error)"=w2343) -> ("error out"=w2340:errorcluster)  [unwired: 1 in, 7 out]
                    }
                    frame #1 {
                      n880 = Read from Text File(file (use dialog)=w2359, count=-1 ("Count  3"), error in=w2358) -> (refnum out=w2360:refnum<file>, text=w2364:string, error out=w2361:errorcluster)  [unwired: 1 in, 1 out]
                      n881 = local write "String_cinetica"(w2364) -> ()
                      n882 = Close File(refnum=w2360, error in=w2361) -> (error out=w2362:errorcluster)  [unwired: 1 out]
                      n883 = call <vilib>:"Simple Error Handler.vi"("error in (no error)"=w2362) -> ()  [unwired: 1 in, 8 out]
                    }
                    frame #2 {
                      n884 = local write "P T  index"(0 ("P T  index")) -> ()
                      n885 = local write "T subarray 2"(dbl[] [0.0, 1.0] ("subarray")) -> ()
                      n886 = local write "P subarray"(dbl[] [0.0, 1.0] ("subarray")) -> ()
                    }
                  }
                }
              }
              n887 = Greater Or Equal?(x=w2326, y="seconds") -> (x >= y?=w2327:bool)
              n888 = feedback-in #2(w2327) -> ()
            }
          }
          n889 = property on="correção NTC" class="DigNum (strict)"() -> ("Value"=w2310:dbl)  [unwired: 2 in, 2 out]
          n890 = call "Read P T.vi"("correção NTC"=w2310) -> ("P Set 2 Output 2"=w2322:dbl, "output NTC"=w2312:dbl, "mean H2 sensor"=→"mean H2 sensor (V)":dbl, "termopar K"=w2311:dbl)  [unwired: 7 out]
          "termopar K" <- w2311
          "output NTC" <- w2312
          n891 = stacked-sequence {
            tunnel: "Entrada Gás" -> [w2400 _ _ _]
            tunnel: "Vácuo" -> [_ w2412 _ _]
            tunnel: "Câmara" -> [_ _ w2424 _]
            tunnel: "ATM" -> [_ _ _ w2436]
            frame #0 {
              w2405 = T5 3 items=["no dialog", "OK message", "continue or stop message", "OK message + warnings", "continue/stop + warnings"] ("type of dialog (OK msg:1)")
              n892 = property on="Entrada gás" class="Bool (strict)"("Value"=w2400) -> ()  [unwired: 2 in, 2 out]
              n893 = call-poly <vilib>:"DAQmx Create Virtual Channel.vi"("lines"=tag "Dev1/port0/line1") -> ("task out"=w2403:refnum<k21>, "error out"=w2404:errorcluster)  [unwired: 13 in]
              n894 = call <vilib>:"DAQmx Start Task.vi"("task/channels in"=w2403, "error in"=w2404) -> ("task out"=w2406:refnum<k21>, "error out"=w2407:errorcluster)  [unwired: 12 in]
              n895 = call-poly <vilib>:"DAQmx Write.vi"("task/channels in"=w2406, "data"=w2400, "error in"=w2407) -> ("task out"=w2411:refnum<k21>, "error out"=w2408:errorcluster)  [unwired: 10 in, 1 out]
              n896 = call <vilib>:"DAQmx Stop Task.vi"("task/channels in"=w2411, "error in"=w2408) -> ("task out"=w2410:refnum<k21>, "error out"=w2409:errorcluster)  [unwired: 12 in]
              n897 = call <vilib>:"DAQmx Clear Task.vi"("task in"=w2410, "error in"=w2409) -> ("error out"=w2402:errorcluster)  [unwired: 13 in]
              n898 = call <vilib>:"Simple Error Handler.vi"("type of dialog (OK msg:1)"=w2405, "error in (no error)"=w2402) -> ()  [unwired: 3 in, 5 out]
            }
            frame #1 {
              w2417 = T5 3 items=["no dialog", "OK message", "continue or stop message", "OK message + warnings", "continue/stop + warnings"] ("type of dialog (OK msg:1)")
              n899 = property on="Vácuo" class="Bool (strict)"("Value"=w2412) -> ()  [unwired: 2 in, 2 out]
              n900 = call-poly <vilib>:"DAQmx Create Virtual Channel.vi"("lines"=tag "Dev1/port0/line2") -> ("task out"=w2415:refnum<k21>, "error out"=w2416:errorcluster)  [unwired: 13 in]
              n901 = call <vilib>:"DAQmx Start Task.vi"("task/channels in"=w2415, "error in"=w2416) -> ("task out"=w2418:refnum<k21>, "error out"=w2419:errorcluster)  [unwired: 12 in]
              n902 = call-poly <vilib>:"DAQmx Write.vi"("task/channels in"=w2418, "data"=w2412, "error in"=w2419) -> ("task out"=w2423:refnum<k21>, "error out"=w2420:errorcluster)  [unwired: 10 in, 1 out]
              n903 = call <vilib>:"DAQmx Stop Task.vi"("task/channels in"=w2423, "error in"=w2420) -> ("task out"=w2422:refnum<k21>, "error out"=w2421:errorcluster)  [unwired: 12 in]
              n904 = call <vilib>:"DAQmx Clear Task.vi"("task in"=w2422, "error in"=w2421) -> ("error out"=w2414:errorcluster)  [unwired: 13 in]
              n905 = call <vilib>:"Simple Error Handler.vi"("type of dialog (OK msg:1)"=w2417, "error in (no error)"=w2414) -> ()  [unwired: 3 in, 5 out]
            }
            frame #2 {
              w2429 = T5 3 items=["no dialog", "OK message", "continue or stop message", "OK message + warnings", "continue/stop + warnings"] ("type of dialog (OK msg:1)")
              n906 = property on="Câmara" class="Bool (strict)"("Value"=w2424) -> ()  [unwired: 2 in, 2 out]
              n907 = call-poly <vilib>:"DAQmx Create Virtual Channel.vi"("lines"=tag "Dev1/port0/line3") -> ("task out"=w2427:refnum<k21>, "error out"=w2428:errorcluster)  [unwired: 13 in]
              n908 = call <vilib>:"DAQmx Start Task.vi"("task/channels in"=w2427, "error in"=w2428) -> ("task out"=w2430:refnum<k21>, "error out"=w2431:errorcluster)  [unwired: 12 in]
              n909 = call-poly <vilib>:"DAQmx Write.vi"("task/channels in"=w2430, "data"=w2424, "error in"=w2431) -> ("task out"=w2435:refnum<k21>, "error out"=w2432:errorcluster)  [unwired: 10 in, 1 out]
              n910 = call <vilib>:"DAQmx Stop Task.vi"("task/channels in"=w2435, "error in"=w2432) -> ("task out"=w2434:refnum<k21>, "error out"=w2433:errorcluster)  [unwired: 12 in]
              n911 = call <vilib>:"DAQmx Clear Task.vi"("task in"=w2434, "error in"=w2433) -> ("error out"=w2426:errorcluster)  [unwired: 13 in]
              n912 = call <vilib>:"Simple Error Handler.vi"("type of dialog (OK msg:1)"=w2429, "error in (no error)"=w2426) -> ()  [unwired: 3 in, 5 out]
            }
            frame #3 {
              w2441 = T5 3 items=["no dialog", "OK message", "continue or stop message", "OK message + warnings", "continue/stop + warnings"] ("type of dialog (OK msg:1)")
              n913 = property on="Atm" class="Bool (strict)"("Value"=w2436) -> ()  [unwired: 2 in, 2 out]
              n914 = call-poly <vilib>:"DAQmx Create Virtual Channel.vi"("lines"=tag "Dev1/port0/line4") -> ("task out"=w2439:refnum<k21>, "error out"=w2440:errorcluster)  [unwired: 13 in]
              n915 = call <vilib>:"DAQmx Start Task.vi"("task/channels in"=w2439, "error in"=w2440) -> ("task out"=w2442:refnum<k21>, "error out"=w2443:errorcluster)  [unwired: 12 in]
              n916 = call-poly <vilib>:"DAQmx Write.vi"("task/channels in"=w2442, "data"=w2436, "error in"=w2443) -> ("task out"=w2447:refnum<k21>, "error out"=w2444:errorcluster)  [unwired: 10 in, 1 out]
              n917 = call <vilib>:"DAQmx Stop Task.vi"("task/channels in"=w2447, "error in"=w2444) -> ("task out"=w2446:refnum<k21>, "error out"=w2445:errorcluster)  [unwired: 12 in]
              n918 = call <vilib>:"DAQmx Clear Task.vi"("task in"=w2446, "error in"=w2445) -> ("error out"=w2438:errorcluster)  [unwired: 13 in]
              n919 = call <vilib>:"Simple Error Handler.vi"("type of dialog (OK msg:1)"=w2441, "error in (no error)"=w2438) -> ()  [unwired: 3 in, 5 out]
            }
          }
          n920 = Multiply(x=w2322, y=10.0) -> (x*y=w2316:dbl)
          n921 = local write "Vol Ref"(w2316) -> ()
          n922 = stacked-sequence {
            tunnel: w2316 -> [w2392 _]
            tunnel: w2312 -> [w2371 _]
            frame #0 {
              w2370 = 2 ("y")
              n923 = property on="P subarray" class="Arr (strict)"() -> ("Value"=w2394:dbl[])  [unwired: 2 in, 2 out]
              n924 = property on="P T  index" class="DigNum (strict)"() -> ("Value"=w2372:i32)  [unwired: 2 in, 2 out]
              n925 = Replace Array Subset(array=w2394, new element=w2392, index=w2372) -> (w2390:dbl[])
              n926 = property on="T subarray 2" class="Arr (strict)"() -> ("Value"=w2381:dbl[])  [unwired: 2 in, 2 out]
              n927 = Replace Array Subset(array=w2381, new element=w2371, index=w2372) -> (w2378:dbl[])
              n928 = call-poly <vilib>:"Array To Matrix.vi"("Real 1D Array"=w2390) -> ("Real Matrix (Column Vector)"=w2397:T3)
              n929 = Matrix Size(0:w2397) -> (1:w2396:i32, 2:w2395:i32)
              n930 = call-poly <vilib>:"Array To Matrix.vi"("Real 1D Array"=w2378) -> ("Real Matrix (Column Vector)"=w2384:T3)
              n931 = Matrix Size(0:w2384) -> (1:w2383:i32, 2:w2382:i32)
              n932 = Increment(x=w2396) -> (x+1=w2385:i32)
              n933 = Subtract(x=w2385, y=w2370) -> (x-y=w2386:i32)
              n934 = Resize Matrix(1:w2395, 2:w2385, 4:w2397) -> (0:w2393:T3)
              n935 = Increment(x=w2383) -> (x+1=w2373:i32)
              n936 = Subtract(x=w2373, y=w2370) -> (x-y=w2374:i32)
              n937 = Resize Matrix(1:w2382, 2:w2373, 4:w2384) -> (0:w2380:T3)
              n938 = call-poly <vilib>:"Matrix To Array.vi"("Real Matrix"=w2393) -> ("Real 2D Array"=w2388:dbl[][])
              n939 = call-poly <vilib>:"Matrix To Array.vi"("Real Matrix"=w2380) -> ("Real 2D Array"=w2376:dbl[][])
              n940 = Reshape Array(w2388, w2385) -> (w2387:dbl[])
              n941 = Reshape Array(w2376, w2373) -> (w2375:dbl[])
              n942 = local write "P subarray"(w2387) -> ()
              n943 = Reshape Array(w2387, w2386) -> (w2389:dbl[])
              n944 = local write "T subarray 2"(w2375) -> ()
              n945 = call <vilib>:"Mean.vi"("X"=w2389) -> ("mean"=→"P cinetica mean":dbl)  [unwired: 1 out]
              n946 = Reshape Array(w2375, w2374) -> (w2377:dbl[])
              n947 = call <vilib>:"Mean.vi"("X"=w2377) -> ("mean"=→"T cinetica mean 2":dbl)  [unwired: 1 out]
            }
            frame #1 {
              n948 = property on="P T  index" class="DigNum (strict)"() -> ("Value"=w2399:i32)  [unwired: 2 in, 2 out]
              n949 = Increment(x=w2399) -> (x+1=w2398:i32)
              n950 = local write "P T  index"(w2398) -> ()
            }
          }
          n951 = Merge Signals(w2316, w2312, w2311) -> (→"P-manual":dynamicdata)
          "N" <- w2321
        }
        n952 = case shown="True" "Save manual" {
          selector: "Save manual" -> [_ w2249]
          frame False {
          }
          frame True {
            n953 = feedback #3() -> (w2245:dbl)  [unwired: 1 in]
            n954 = Equal To 0?(x=w2245) -> (x = 0?=w2251:bool)
            n955 = stacked-sequence {
              tunnel: w2251 -> [_ w2267 _]
              tunnel: [_ w2266 _] -> w2247
              frame #0 {
                w2260 = i16 3 ("precision (6)")
                n956 = property on="T fit" class="DigNum (strict)"() -> ("Value"=w2262:dbl)  [unwired: 2 in, 2 out]
                n957 = property on="p fit" class="DigNum (strict)"() -> ("Value"=w2263:dbl)  [unwired: 2 in, 2 out]
                n958 = property on="termopar K" class="DigNum (strict)"() -> ("Value"=w2261:dbl)  [unwired: 2 in, 2 out]
                n959 = Number To Fractional String(number=w2262, precision (6)=w2260) -> (F-format string=→"T string":string)  [unwired: 2 in]
                n960 = Number To Fractional String(number=w2263, precision (6)=w2260) -> (F-format string=→"P string":string)  [unwired: 2 in]
                n961 = Number To Fractional String(number=w2261, precision (6)=w2260) -> (F-format string=→"termopar K":string)  [unwired: 2 in]
              }
              frame #1 {
                n962 = case shown="True" w2267 {
                  tunnel: [TRUE ("y") FALSE ("y")] -> w2266
                  frame False {
                    n963 = property on="path" class="Path"() -> ("Value"=w2271:path)  [unwired: 2 in, 2 out]
                    n964 = property on="P string" class="Str"() -> ("Value"=w2270:string)  [unwired: 2 in, 2 out]
                    n965 = Concatenate Strings(w2270, "\t") -> (w2268:string)
                    n966 = Open/Create/Replace File(file path (use dialog)=w2271, operation (0:open)=T2."open") -> (refnum out=w2275:refnum<file>, error out=w2274:errorcluster)  [unwired: 2 in, 3 out]
                    n967 = Set File Position(refnum=w2275, from (0:start)=enum16{"start", "end", "current"}."end", error in=w2274) -> (refnum out=w2277:refnum<file>, error out=w2278:errorcluster)  [unwired: 1 in]
                    n968 = Write to Text File(file (use dialog)=w2277, text=w2268, error in=w2278) -> (refnum out=w2273:refnum<file>, error out=w2272:errorcluster)  [unwired: 2 out]
                    n969 = Close File(refnum=w2273, error in=w2272) -> (error out=w2280:errorcluster)  [unwired: 1 out]
                    n970 = call <vilib>:"Simple Error Handler.vi"("error in (no error)"=w2280) -> ()  [unwired: 1 in, 8 out]
                  }
                  frame True {
                    w2283 = "\t"
                    n971 = property on="path" class="Path"() -> ("Value"=w2290:path)  [unwired: 2 in, 2 out]
                    n972 = property on="Count SET" class="DigNum (strict)"() -> ("Value"=w2286:i32)  [unwired: 2 in, 2 out]
                    n973 = Open/Create/Replace File(file path (use dialog)=w2290, operation (0:open)=T2."open") -> (refnum out=w2289:refnum<file>, error out=w2288:errorcluster)  [unwired: 2 in, 3 out]
                    n974 = Increment(x=w2286) -> (x+1=w2287:i32)
                    "Set atual" <- w2287
                    n975 = Set File Position(refnum=w2289, from (0:start)=enum16{"start", "end", "current"}."end", error in=w2288) -> (refnum out=w2298:refnum<file>, error out=w2299:errorcluster)  [unwired: 1 in]
                    n976 = Number To Decimal String(number=w2287) -> (decimal integer string=w2291:string)  [unwired: 1 in]
                    n977 = property on="termopar K" class="Str"() -> ("Value"=w2282:string)  [unwired: 2 in, 2 out]
                    n978 = property on="T string" class="Str"() -> ("Value"=w2284:string)  [unwired: 2 in, 2 out]
                    n979 = Concatenate Strings(w2284, w2283, w2282, "\r\n", w2291, w2283) -> (w2293:string)
                    n980 = Write to Text File(file (use dialog)=w2298, text=w2293, error in=w2299) -> (refnum out=w2296:refnum<file>, error out=w2295:errorcluster)  [unwired: 2 out]
                    n981 = Close File(refnum=w2296, error in=w2295) -> (error out=w2301:errorcluster)  [unwired: 1 out]
                    n982 = call <vilib>:"Simple Error Handler.vi"("error in (no error)"=w2301) -> ()  [unwired: 1 in, 8 out]
                    "T" <- TRUE ("T")
                  }
                }
              }
              frame #2 {
                n983 = property on="path" class="Path"() -> ("Value"=w2303:path)  [unwired: 2 in, 2 out]
                n984 = property on="Set atual" class="DigNum (strict)"() -> ("Value"=w2302:i32)  [unwired: 2 in, 2 out]
                n985 = local write "Count SET"(w2302) -> ()
                n986 = Read from Text File(file (use dialog)=w2303, count=-1 ("Count  3")) -> (refnum out=w2305:refnum<file>, text=w2304:string, error out=w2306:errorcluster)  [unwired: 2 in, 1 out]
                n987 = property on="String 2" class="Str"("Value"=w2304) -> ()  [unwired: 2 in, 2 out]
                n988 = Close File(refnum=w2305, error in=w2306) -> (error out=w2308:errorcluster)  [unwired: 1 out]
                n989 = call <vilib>:"Simple Error Handler.vi"("error in (no error)"=w2308) -> ()  [unwired: 1 in, 8 out]
              }
            }
            n990 = Implies(1:w2247, 2:w2249) -> (0:w2248:bool)
            n991 = Select(t=w2245, s=w2248, f=5.0 ("t")) -> (s? t:f=w2246:dbl)
            n992 = case shown="1" w2246 {
              frame 0, Default {
              }
              frame 1 {
                "ZPf2" <- TRUE ("ZPf2")
              }
              frame 2 {
                "Pf2" <- TRUE ("Pf2")
              }
              frame 3 {
                "Pit" <- TRUE ("Pit")
              }
              frame 4 {
                n993 = local write "T"(FALSE ("T")) -> ()
                "ZPit" <- TRUE ("ZPit")
              }
              frame 5 {
                w2258 = FALSE
                n994 = local write "Pit"(w2258) -> ()
                n995 = local write "ZPf2"(w2258) -> ()
                n996 = local write "ZPit"(w2258) -> ()
                n997 = local write "Pf2"(w2258) -> ()
              }
            }
            n998 = Decrement(x=w2246) -> (x-1=w2252:dbl)
            n999 = feedback-in #3(w2252) -> ()
          }
        }
        n1000 = case shown="True" w1632 {
          tunnel: [FALSE ("Save manual") w2244] -> w1634
          tunnel: "Save manual" -> [_ w2244]
          frame False {
          }
          frame True {
          }
        }
        n1001 = case shown="True" w1632 {
          tunnel: [FALSE w1652] -> w1635
          tunnel: w1634 -> [_ w1651]
          tunnel: w1633 -> [_ w1650]
          frame False {
          }
          frame True {
            n1002 = flat-sequence {
              tunnel: w1650 -> [w1673]
              tunnel: w1651 -> [w1674]
              tunnel: [w1674] -> w1671
              tunnel: [w1673] -> w1670
              tunnel: [w1681] -> w1669
              tunnel: [w1682] -> w1668
              tunnel: [w1683] -> w1667
              tunnel: [w1684] -> w1666
              tunnel: [w1685] -> w1665
              tunnel: [w1686] -> w1664
              tunnel: [w1687] -> w1663
              tunnel: [w1689] -> w1662
              tunnel: [w1690] -> w1661
              tunnel: [w1691] -> w1660
              tunnel: [w1692] -> w1659
              tunnel: [w1693] -> w1658
              tunnel: [w1688] -> w1657
              tunnel: [w1680] -> w1656
              tunnel: [w1679] -> w1655
              tunnel: [w1678] -> w1654
              tunnel: [w1677] -> w1653
              tunnel: w1671 -> [w1676]
              tunnel: w1670 -> [w1675]
              tunnel: w1669 -> [w2191]
              tunnel: w1668 -> [w2190]
              tunnel: w1667 -> [w2189]
              tunnel: w1666 -> [w2188]
              tunnel: w1665 -> [w2187]
              tunnel: w1664 -> [w2186]
              tunnel: w1663 -> [w2185]
              tunnel: w1662 -> [w2184]
              tunnel: w1661 -> [w2183]
              tunnel: w1660 -> [w2182]
              tunnel: w1659 -> [w2181]
              tunnel: w1658 -> [w2180]
              tunnel: w1657 -> [w2179]
              tunnel: w1656 -> [w2192]
              tunnel: w1655 -> [w2193]
              tunnel: w1654 -> [w2194]
              tunnel: [w2177] -> w1652
              tunnel: w1653 -> [w2177]
              tunnel: [TRUE] -> w1649
              frame #0 {
                n1003 = local write "graph RLC"(FALSE) -> ()
              }
              frame #1 {
                n1004 = case shown="True" w1676 {
                  tunnel: [_ w1728] -> w1677
                  tunnel: w1675 -> [_ w1710]
                  tunnel: [_ w1709] -> w1678
                  tunnel: [_ w1708] -> w1679
                  tunnel: [_ w1707] -> w1680
                  tunnel: [_ w1706] -> w1681
                  tunnel: [_ w1705] -> w1682
                  tunnel: [_ w1704] -> w1683
                  tunnel: [_ w1703] -> w1684
                  tunnel: [_ w1702] -> w1685
                  tunnel: [_ w1701] -> w1686
                  tunnel: [_ w1700] -> w1687
                  tunnel: [_ w1699] -> w1688
                  tunnel: [_ w1698] -> w1689
                  tunnel: [_ w1697] -> w1690
                  tunnel: [_ w1696] -> w1691
                  tunnel: [_ w1695] -> w1692
                  tunnel: [_ w1694] -> w1693
                  frame False {
                  }
                  frame True {
                    n1005 = for {
                      N: 5 -> [_]
                      tunnel: TRUE -> [w1751]
                      tunnel: FALSE -> [w1750]
                      tunnel: [w1749] -> w1728
                      tunnel: [w1748] -> w1726 mode=indexing
                      tunnel: [w1747] -> w1725 mode=indexing
                      tunnel: [w1746] -> w1724 mode=indexing
                      tunnel: [w1745] -> w1723 mode=indexing
                      tunnel: [w1744] -> w1722 mode=indexing
                      tunnel: [w1743] -> w1721 mode=indexing
                      tunnel: [w1742] -> w1720 mode=indexing
                      tunnel: [w1741] -> w1719 mode=indexing
                      tunnel: [w1740] -> w1718 mode=indexing
                      tunnel: [w1739] -> w1717 mode=indexing
                      tunnel: [w1738] -> w1716 mode=indexing
                      tunnel: [w1737] -> w1715 mode=indexing
                      tunnel: [w1736] -> w1714 mode=indexing
                      tunnel: [w1735] -> w1713 mode=indexing
                      tunnel: [w1734] -> w1712 mode=indexing
                      tunnel: [w1733] -> w1711 mode=indexing
                      tunnel: w1710 -> [w1732]
                      n1006 = property on="path RLC_completo" class="Path"() -> ("Value"=w1731:path)  [unwired: 2 in, 2 out]
                      n1007 = stacked-sequence {
                        tunnel: w1751 -> [_ w1776 w1801 w1826 w1851 w1876 w1901 w1926 w1949 w1974 w2001 w2024 w2051 w2076 w2101 w2124 w2151 _]
                        tunnel: w1750 -> [w1752 _ _ _ _ _ _ _ _ _ _ _ _ _ _ _ _ w2175]
                        tunnel: [_ _ _ _ _ _ _ _ _ _ _ _ _ _ _ _ _ TRUE] -> w1749
                        tunnel: [_ w1775 _ _ _ _ _ _ _ _ _ _ _ _ _ _ _ _] -> w1748
                        tunnel: [_ _ w1800 _ _ _ _ _ _ _ _ _ _ _ _ _ _ _] -> w1747
                        tunnel: [_ _ _ w1825 _ _ _ _ _ _ _ _ _ _ _ _ _ _] -> w1746
                        tunnel: [_ _ _ _ w1850 _ _ _ _ _ _ _ _ _ _ _ _ _] -> w1745
                        tunnel: [_ _ _ _ _ w1875 _ _ _ _ _ _ _ _ _ _ _ _] -> w1744
                        tunnel: [_ _ _ _ _ _ w1900 _ _ _ _ _ _ _ _ _ _ _] -> w1743
                        tunnel: [_ _ _ _ _ _ _ w1925 _ _ _ _ _ _ _ _ _ _] -> w1742
                        tunnel: [_ _ _ _ _ _ _ _ w1951 _ _ _ _ _ _ _ _ _] -> w1741
                        tunnel: [_ _ _ _ _ _ _ _ _ w1976 _ _ _ _ _ _ _ _] -> w1740
                        tunnel: [_ _ _ _ _ _ _ _ _ _ w2000 _ _ _ _ _ _ _] -> w1739
                        tunnel: [_ _ _ _ _ _ _ _ _ _ _ w2026 _ _ _ _ _ _] -> w1738
                        tunnel: [_ _ _ _ _ _ _ _ _ _ _ _ w2050 _ _ _ _ _] -> w1737
                        tunnel: [_ _ _ _ _ _ _ _ _ _ _ _ _ w2075 _ _ _ _] -> w1736
                        tunnel: [_ _ _ _ _ _ _ _ _ _ _ _ _ _ w2100 _ _ _] -> w1735
                        tunnel: [_ _ _ _ _ _ _ _ _ _ _ _ _ _ _ w2126 _ _] -> w1734
                        tunnel: [_ _ _ _ _ _ _ _ _ _ _ _ _ _ _ _ w2150 _] -> w1733
                        tunnel: w1732 -> [_ w1778 w1804 w1828 w1853 w1878 w1903 w1928 w1953 w1978 w2003 w2028 w2053 w2078 w2103 w2128 w2153 _]
                        tunnel: w1731 -> [w1754 w1777 w1803 w1827 w1852 w1877 w1902 w1927 w1952 w1977 w2002 w2027 w2052 w2077 w2102 w2127 w2152 _]
                        frame #0 {
                          w1755 = "\t"
                          n1008 = local write "C-50-L"(w1752) -> ()
                          n1009 = local write "C-50-N"(w1752) -> ()
                          n1010 = local write "Z-50-L"(w1752) -> ()
                          n1011 = local write "Z-50-N"(w1752) -> ()
                          n1012 = local write "C-1K-L"(w1752) -> ()
                          n1013 = local write "C-1K-N"(w1752) -> ()
                          n1014 = local write "Z-1K-N"(w1752) -> ()
                          n1015 = local write "Z-1K-L"(w1752) -> ()
                          n1016 = local write "Z-100-L"(w1752) -> ()
                          n1017 = local write "C-10K-L"(w1752) -> ()
                          n1018 = local write "C-100-N"(w1752) -> ()
                          n1019 = local write "C-10K-N"(w1752) -> ()
                          n1020 = local write "Z-10K-N"(w1752) -> ()
                          n1021 = local write "Z-10K-L"(w1752) -> ()
                          n1022 = local write "Z-100-N"(w1752) -> ()
                          n1023 = local write "C-100-L"(w1752) -> ()
                          n1024 = Open/Create/Replace File(file path (use dialog)=w1754, operation (0:open)=T2."open") -> (refnum out=w1768:refnum<file>, error out=w1767:errorcluster)  [unwired: 2 in, 3 out]
                          n1025 = Get Date/Time String(date format (0)=enum16{"short", "long", "abbreviated"}."short", want seconds? (F)=TRUE) -> (date string=w1760:string, time string=w1759:string)  [unwired: 1 in]
                          n1026 = feedback #4() -> (w1753:dbl)  [unwired: 1 in]
                          n1027 = local write "SET 2"(w1753) -> ()
                          n1028 = Set File Position(refnum=w1768, from (0:start)=enum16{"start", "end", "current"}."end", error in=w1767) -> (refnum out=w1770:refnum<file>, error out=w1771:errorcluster)  [unwired: 1 in]
                          n1029 = Number To Fractional String(number=w1753, precision (6)=i16 2) -> (F-format string=w1758:string)  [unwired: 2 in]
                          n1030 = Add(x=w1753, y=0.2) -> (x+y=w1764:dbl)
                          n1031 = feedback-in #4(w1764) -> ()
                          n1032 = Concatenate Strings(w1758, w1755, w1760, w1755, w1759, w1755) -> (w1757:string)
                          n1033 = Write to Text File(file (use dialog)=w1770, text=w1757, error in=w1771) -> (refnum out=w1766:refnum<file>, error out=w1765:errorcluster)  [unwired: 1 in, 1 out]
                          n1034 = Close File(refnum=w1766, error in=w1765) -> (error out=w1773:errorcluster)  [unwired: 1 out]
                          n1035 = call <vilib>:"Simple Error Handler.vi"("error in (no error)"=w1773) -> ()  [unwired: 1 in, 8 out]
                        }
                        frame #1 {
                          w1779 = "\t"
                          w1796 = i16 4 ("width (-)")
                          n1036 = local write "C-50-L"(w1776) -> ()
                          n1037 = Wait (ms)(milliseconds to wait=u32 5000) -> ()  [unwired: 1 out]
                          n1038 = Open/Create/Replace File(file path (use dialog)=w1777, operation (0:open)=T2."open") -> (refnum out=w1788:refnum<file>, error out=w1787:errorcluster)  [unwired: 2 in, 3 out]
                          n1039 = Set File Position(refnum=w1788, from (0:start)=enum16{"start", "end", "current"}."end", error in=w1787) -> (refnum out=w1790:refnum<file>, error out=w1791:errorcluster)  [unwired: 1 in]
                          n1040 = call "RLC_read.vi"("Path"=w1778, "String"="cmd /c rlc_read_cAL.py") -> ("MEASURE A"=w1775:dbl, "MEASURE V [V]"=w1795:dbl, "MEASURE B"=w1774:dbl, "MEASURE I [A]"=w1794:dbl)  [unwired: 2 out]
                          n1041 = Number To Engineering String(2:w1796, 4:w1794) -> (0:w1780:string)  [unwired: 2 in]
                          n1042 = local write "MEASURE A"(w1775) -> ()
                          n1043 = local write "MEASURE B"(w1774) -> ()
                          n1044 = Number To Engineering String(2:w1796, 4:w1795) -> (0:w1781:string)  [unwired: 2 in]
                          n1045 = Number To Engineering String(2:w1796, 4:w1775) -> (0:w1783:string)  [unwired: 2 in]
                          n1046 = Number To Engineering String(2:w1796, 4:w1774) -> (0:w1782:string)  [unwired: 2 in]
                          n1047 = Concatenate Strings(w1783, w1779, w1782, w1779, w1781, w1779, w1780, w1779) -> (w1784:string)
                          n1048 = Write to Text File(file (use dialog)=w1790, text=w1784, error in=w1791) -> (refnum out=w1786:refnum<file>, error out=w1785:errorcluster)  [unwired: 1 in, 1 out]
                          n1049 = Close File(refnum=w1786, error in=w1785) -> (error out=w1793:errorcluster)  [unwired: 1 out]
                          n1050 = call <vilib>:"Simple Error Handler.vi"("error in (no error)"=w1793) -> ()  [unwired: 1 in, 8 out]
                        }
                        frame #2 {
                          w1807 = "\t"
                          w1821 = i16 4 ("width (-)")
                          n1051 = local write "C-50-N"(w1801) -> ()
                          n1052 = Wait (ms)(milliseconds to wait=u32 5000) -> ()  [unwired: 1 out]
                          n1053 = Open/Create/Replace File(file path (use dialog)=w1803, operation (0:open)=T2."open") -> (refnum out=w1815:refnum<file>, error out=w1814:errorcluster)  [unwired: 2 in, 3 out]
                          n1054 = Set File Position(refnum=w1815, from (0:start)=enum16{"start", "end", "current"}."end", error in=w1814) -> (refnum out=w1817:refnum<file>, error out=w1818:errorcluster)  [unwired: 1 in]
                          n1055 = call "RLC_read.vi"("Path"=w1804, "String"="cmd /c rlc_read_cAN.py") -> ("MEASURE A"=w1800:dbl, "MEASURE V [V]"=w1806:dbl, "MEASURE B"=w1799:dbl, "MEASURE I [A]"=w1805:dbl)  [unwired: 2 out]
                          n1056 = Number To Engineering String(2:w1821, 4:w1805) -> (0:w1808:string)  [unwired: 2 in]
                          n1057 = local write "MEASURE A 2"(w1800) -> ()
                          n1058 = local write "MEASURE B 2"(w1799) -> ()
                          n1059 = Number To Engineering String(2:w1821, 4:w1806) -> (0:w1809:string)  [unwired: 2 in]
                          n1060 = Number To Engineering String(2:w1821, 4:w1800) -> (0:w1811:string)  [unwired: 2 in]
                          n1061 = Number To Engineering String(2:w1821, 4:w1799) -> (0:w1810:string)  [unwired: 2 in]
                          n1062 = Concatenate Strings(w1811, w1807, w1810, w1807, w1809, w1807, w1808, w1807) -> (w1802:string)
                          n1063 = Write to Text File(file (use dialog)=w1817, text=w1802, error in=w1818) -> (refnum out=w1813:refnum<file>, error out=w1812:errorcluster)  [unwired: 1 in, 1 out]
                          n1064 = Close File(refnum=w1813, error in=w1812) -> (error out=w1820:errorcluster)  [unwired: 1 out]
                          n1065 = call <vilib>:"Simple Error Handler.vi"("error in (no error)"=w1820) -> ()  [unwired: 1 in, 8 out]
                        }
                        frame #3 {
                          w1831 = "\t"
                          w1846 = i16 4 ("width (-)")
                          n1066 = Wait (ms)(milliseconds to wait=u32 5000) -> ()  [unwired: 1 out]
                          n1067 = local write "C-100-L"(w1826) -> ()
                          n1068 = Open/Create/Replace File(file path (use dialog)=w1827, operation (0:open)=T2."open") -> (refnum out=w1840:refnum<file>, error out=w1839:errorcluster)  [unwired: 2 in, 3 out]
                          n1069 = Set File Position(refnum=w1840, from (0:start)=enum16{"start", "end", "current"}."end", error in=w1839) -> (refnum out=w1842:refnum<file>, error out=w1843:errorcluster)  [unwired: 1 in]
                          n1070 = call "RLC_read.vi"("Path"=w1828, "String"="cmd /c rlc_read_cBL.py") -> ("MEASURE A"=w1825:dbl, "MEASURE V [V]"=w1830:dbl, "MEASURE B"=w1824:dbl, "MEASURE I [A]"=w1829:dbl)  [unwired: 2 out]
                          n1071 = Number To Engineering String(2:w1846, 4:w1829) -> (0:w1832:string)  [unwired: 2 in]
                          n1072 = local write "MEASURE A 3"(w1825) -> ()
                          n1073 = local write "MEASURE B 3"(w1824) -> ()
                          n1074 = Number To Engineering String(2:w1846, 4:w1830) -> (0:w1833:string)  [unwired: 2 in]
                          n1075 = Number To Engineering String(2:w1846, 4:w1825) -> (0:w1835:string)  [unwired: 2 in]
                          n1076 = Number To Engineering String(2:w1846, 4:w1824) -> (0:w1834:string)  [unwired: 2 in]
                          n1077 = Concatenate Strings(w1835, w1831, w1834, w1831, w1833, w1831, w1832, w1831) -> (w1836:string)
                          n1078 = Write to Text File(file (use dialog)=w1842, text=w1836, error in=w1843) -> (refnum out=w1838:refnum<file>, error out=w1837:errorcluster)  [unwired: 1 in, 1 out]
                          n1079 = Close File(refnum=w1838, error in=w1837) -> (error out=w1845:errorcluster)  [unwired: 1 out]
                          n1080 = call <vilib>:"Simple Error Handler.vi"("error in (no error)"=w1845) -> ()  [unwired: 1 in, 8 out]
                        }
                        frame #4 {
                          w1856 = "\t"
                          w1871 = i16 4 ("width (-)")
                          n1081 = Wait (ms)(milliseconds to wait=u32 5000) -> ()  [unwired: 1 out]
                          n1082 = local write "C-100-N"(w1851) -> ()
                          n1083 = Open/Create/Replace File(file path (use dialog)=w1852, operation (0:open)=T2."open") -> (refnum out=w1865:refnum<file>, error out=w1864:errorcluster)  [unwired: 2 in, 3 out]
                          n1084 = Set File Position(refnum=w1865, from (0:start)=enum16{"start", "end", "current"}."end", error in=w1864) -> (refnum out=w1867:refnum<file>, error out=w1868:errorcluster)  [unwired: 1 in]
                          n1085 = call "RLC_read.vi"("Path"=w1853, "String"="cmd /c rlc_read_cBN.py") -> ("MEASURE A"=w1850:dbl, "MEASURE V [V]"=w1855:dbl, "MEASURE B"=w1849:dbl, "MEASURE I [A]"=w1854:dbl)  [unwired: 2 out]
                          n1086 = Number To Engineering String(2:w1871, 4:w1854) -> (0:w1857:string)  [unwired: 2 in]
                          n1087 = local write "MEASURE A 4"(w1850) -> ()
                          n1088 = local write "MEASURE B 4"(w1849) -> ()
                          n1089 = Number To Engineering String(2:w1871, 4:w1855) -> (0:w1858:string)  [unwired: 2 in]
                          n1090 = Number To Engineering String(2:w1871, 4:w1850) -> (0:w1860:string)  [unwired: 2 in]
                          n1091 = Number To Engineering String(2:w1871, 4:w1849) -> (0:w1859:string)  [unwired: 2 in]
                          n1092 = Concatenate Strings(w1860, w1856, w1859, w1856, w1858, w1856, w1857, w1856) -> (w1861:string)
                          n1093 = Write to Text File(file (use dialog)=w1867, text=w1861, error in=w1868) -> (refnum out=w1863:refnum<file>, error out=w1862:errorcluster)  [unwired: 1 in, 1 out]
                          n1094 = Close File(refnum=w1863, error in=w1862) -> (error out=w1870:errorcluster)  [unwired: 1 out]
                          n1095 = call <vilib>:"Simple Error Handler.vi"("error in (no error)"=w1870) -> ()  [unwired: 1 in, 8 out]
                        }
                        frame #5 {
                          w1896 = "\t"
                          w1881 = i16 4 ("width (-)")
                          n1096 = local write "C-1K-L"(w1876) -> ()
                          n1097 = Wait (ms)(milliseconds to wait=u32 5000) -> ()  [unwired: 1 out]
                          n1098 = Open/Create/Replace File(file path (use dialog)=w1877, operation (0:open)=T2."open") -> (refnum out=w1887:refnum<file>, error out=w1888:errorcluster)  [unwired: 2 in, 3 out]
                          n1099 = Set File Position(refnum=w1887, from (0:start)=enum16{"start", "end", "current"}."end", error in=w1888) -> (refnum out=w1885:refnum<file>, error out=w1884:errorcluster)  [unwired: 1 in]
                          n1100 = call "RLC_read.vi"("Path"=w1878, "String"="cmd /c rlc_read_cCL.py") -> ("MEASURE A"=w1875:dbl, "MEASURE V [V]"=w1880:dbl, "MEASURE B"=w1874:dbl, "MEASURE I [A]"=w1879:dbl)  [unwired: 2 out]
                          n1101 = Number To Engineering String(2:w1881, 4:w1879) -> (0:w1895:string)  [unwired: 2 in]
                          n1102 = local write "MEASURE A 5"(w1875) -> ()
                          n1103 = local write "MEASURE B 5"(w1874) -> ()
                          n1104 = Number To Engineering String(2:w1881, 4:w1880) -> (0:w1894:string)  [unwired: 2 in]
                          n1105 = Number To Engineering String(2:w1881, 4:w1875) -> (0:w1892:string)  [unwired: 2 in]
                          n1106 = Number To Engineering String(2:w1881, 4:w1874) -> (0:w1893:string)  [unwired: 2 in]
                          n1107 = Concatenate Strings(w1892, w1896, w1893, w1896, w1894, w1896, w1895, w1896) -> (w1891:string)
                          n1108 = Write to Text File(file (use dialog)=w1885, text=w1891, error in=w1884) -> (refnum out=w1889:refnum<file>, error out=w1890:errorcluster)  [unwired: 1 in, 1 out]
                          n1109 = Close File(refnum=w1889, error in=w1890) -> (error out=w1882:errorcluster)  [unwired: 1 out]
                          n1110 = call <vilib>:"Simple Error Handler.vi"("error in (no error)"=w1882) -> ()  [unwired: 1 in, 8 out]
                        }
                        frame #6 {
                          w1921 = "\t"
                          w1906 = i16 4 ("width (-)")
                          n1111 = local write "C-1K-N"(w1901) -> ()
                          n1112 = Wait (ms)(milliseconds to wait=u32 5000) -> ()  [unwired: 1 out]
                          n1113 = Open/Create/Replace File(file path (use dialog)=w1902, operation (0:open)=T2."open") -> (refnum out=w1912:refnum<file>, error out=w1913:errorcluster)  [unwired: 2 in, 3 out]
                          n1114 = Set File Position(refnum=w1912, from (0:start)=enum16{"start", "end", "current"}."end", error in=w1913) -> (refnum out=w1910:refnum<file>, error out=w1909:errorcluster)  [unwired: 1 in]
                          n1115 = call "RLC_read.vi"("Path"=w1903, "String"="cmd /c rlc_read_cCN.py") -> ("MEASURE A"=w1900:dbl, "MEASURE V [V]"=w1905:dbl, "MEASURE B"=w1899:dbl, "MEASURE I [A]"=w1904:dbl)  [unwired: 2 out]
                          n1116 = Number To Engineering String(2:w1906, 4:w1904) -> (0:w1920:string)  [unwired: 2 in]
                          n1117 = local write "MEASURE A 6"(w1900) -> ()
                          n1118 = local write "MEASURE B 6"(w1899) -> ()
                          n1119 = Number To Engineering String(2:w1906, 4:w1905) -> (0:w1919:string)  [unwired: 2 in]
                          n1120 = Number To Engineering String(2:w1906, 4:w1900) -> (0:w1917:string)  [unwired: 2 in]
                          n1121 = Number To Engineering String(2:w1906, 4:w1899) -> (0:w1918:string)  [unwired: 2 in]
                          n1122 = Concatenate Strings(w1917, w1921, w1918, w1921, w1919, w1921, w1920, w1921) -> (w1916:string)
                          n1123 = Write to Text File(file (use dialog)=w1910, text=w1916, error in=w1909) -> (refnum out=w1914:refnum<file>, error out=w1915:errorcluster)  [unwired: 1 in, 1 out]
                          n1124 = Close File(refnum=w1914, error in=w1915) -> (error out=w1907:errorcluster)  [unwired: 1 out]
                          n1125 = call <vilib>:"Simple Error Handler.vi"("error in (no error)"=w1907) -> ()  [unwired: 1 in, 8 out]
                        }
                        frame #7 {
                          w1931 = "\t"
                          w1946 = i16 4 ("width (-)")
                          n1126 = Wait (ms)(milliseconds to wait=u32 5000) -> ()  [unwired: 1 out]
                          n1127 = local write "C-10K-L"(w1926) -> ()
                          n1128 = Open/Create/Replace File(file path (use dialog)=w1927, operation (0:open)=T2."open") -> (refnum out=w1940:refnum<file>, error out=w1939:errorcluster)  [unwired: 2 in, 3 out]
                          n1129 = Set File Position(refnum=w1940, from (0:start)=enum16{"start", "end", "current"}."end", error in=w1939) -> (refnum out=w1942:refnum<file>, error out=w1943:errorcluster)  [unwired: 1 in]
                          n1130 = call "RLC_read.vi"("Path"=w1928, "String"="cmd /c rlc_read_cDL.py") -> ("MEASURE A"=w1925:dbl, "MEASURE V [V]"=w1930:dbl, "MEASURE B"=w1924:dbl, "MEASURE I [A]"=w1929:dbl)  [unwired: 2 out]
                          n1131 = Number To Engineering String(2:w1946, 4:w1929) -> (0:w1932:string)  [unwired: 2 in]
                          n1132 = local write "MEASURE A 7"(w1925) -> ()
                          n1133 = local write "MEASURE B 7"(w1924) -> ()
                          n1134 = Number To Engineering String(2:w1946, 4:w1930) -> (0:w1933:string)  [unwired: 2 in]
                          n1135 = Number To Engineering String(2:w1946, 4:w1925) -> (0:w1935:string)  [unwired: 2 in]
                          n1136 = Number To Engineering String(2:w1946, 4:w1924) -> (0:w1934:string)  [unwired: 2 in]
                          n1137 = Concatenate Strings(w1935, w1931, w1934, w1931, w1933, w1931, w1932, w1931) -> (w1936:string)
                          n1138 = Write to Text File(file (use dialog)=w1942, text=w1936, error in=w1943) -> (refnum out=w1938:refnum<file>, error out=w1937:errorcluster)  [unwired: 1 in, 1 out]
                          n1139 = Close File(refnum=w1938, error in=w1937) -> (error out=w1945:errorcluster)  [unwired: 1 out]
                          n1140 = call <vilib>:"Simple Error Handler.vi"("error in (no error)"=w1945) -> ()  [unwired: 1 in, 8 out]
                        }
                        frame #8 {
                          w1956 = "\t"
                          w1971 = i16 4 ("width (-)")
                          n1141 = Wait (ms)(milliseconds to wait=u32 5000) -> ()  [unwired: 1 out]
                          n1142 = local write "C-10K-N"(w1949) -> ()
                          n1143 = Open/Create/Replace File(file path (use dialog)=w1952, operation (0:open)=T2."open") -> (refnum out=w1965:refnum<file>, error out=w1964:errorcluster)  [unwired: 2 in, 3 out]
                          n1144 = Set File Position(refnum=w1965, from (0:start)=enum16{"start", "end", "current"}."end", error in=w1964) -> (refnum out=w1967:refnum<file>, error out=w1968:errorcluster)  [unwired: 1 in]
                          n1145 = call "RLC_read.vi"("Path"=w1953, "String"="cmd /c rlc_read_cDN.py") -> ("MEASURE A"=w1951:dbl, "MEASURE V [V]"=w1955:dbl, "MEASURE B"=w1950:dbl, "MEASURE I [A]"=w1954:dbl)  [unwired: 2 out]
                          n1146 = Number To Engineering String(2:w1971, 4:w1954) -> (0:w1957:string)  [unwired: 2 in]
                          n1147 = local write "MEASURE A 8"(w1951) -> ()
                          n1148 = local write "MEASURE B 8"(w1950) -> ()
                          n1149 = Number To Engineering String(2:w1971, 4:w1955) -> (0:w1958:string)  [unwired: 2 in]
                          n1150 = Number To Engineering String(2:w1971, 4:w1951) -> (0:w1960:string)  [unwired: 2 in]
                          n1151 = Number To Engineering String(2:w1971, 4:w1950) -> (0:w1959:string)  [unwired: 2 in]
                          n1152 = Concatenate Strings(w1960, w1956, w1959, w1956, w1958, w1956, w1957, w1956) -> (w1961:string)
                          n1153 = Write to Text File(file (use dialog)=w1967, text=w1961, error in=w1968) -> (refnum out=w1963:refnum<file>, error out=w1962:errorcluster)  [unwired: 1 in, 1 out]
                          n1154 = Close File(refnum=w1963, error in=w1962) -> (error out=w1970:errorcluster)  [unwired: 1 out]
                          n1155 = call <vilib>:"Simple Error Handler.vi"("error in (no error)"=w1970) -> ()  [unwired: 1 in, 8 out]
                        }
                        frame #9 {
                          w1981 = "\t"
                          w1996 = i16 4 ("width (-)")
                          n1156 = local write "Z-50-L"(w1974) -> ()
                          n1157 = Wait (ms)(milliseconds to wait=u32 5000) -> ()  [unwired: 1 out]
                          n1158 = Open/Create/Replace File(file path (use dialog)=w1977, operation (0:open)=T2."open") -> (refnum out=w1990:refnum<file>, error out=w1989:errorcluster)  [unwired: 2 in, 3 out]
                          n1159 = Set File Position(refnum=w1990, from (0:start)=enum16{"start", "end", "current"}."end", error in=w1989) -> (refnum out=w1992:refnum<file>, error out=w1993:errorcluster)  [unwired: 1 in]
                          n1160 = call "RLC_read.vi"("Path"=w1978, "String"="cmd /c rlc_read_ZAL.py") -> ("MEASURE A"=w1976:dbl, "MEASURE V [V]"=w1980:dbl, "MEASURE B"=w1975:dbl, "MEASURE I [A]"=w1979:dbl)  [unwired: 2 out]
                          n1161 = Number To Engineering String(2:w1996, 4:w1979) -> (0:w1982:string)  [unwired: 2 in]
                          n1162 = local write "MEASURE A 9"(w1976) -> ()
                          n1163 = local write "MEASURE B 9"(w1975) -> ()
                          n1164 = Number To Engineering String(2:w1996, 4:w1980) -> (0:w1983:string)  [unwired: 2 in]
                          n1165 = Number To Engineering String(2:w1996, 4:w1976) -> (0:w1985:string)  [unwired: 2 in]
                          n1166 = Number To Engineering String(2:w1996, 4:w1975) -> (0:w1984:string)  [unwired: 2 in]
                          n1167 = Concatenate Strings(w1985, w1981, w1984, w1981, w1983, w1981, w1982, w1981) -> (w1986:string)
                          n1168 = Write to Text File(file (use dialog)=w1992, text=w1986, error in=w1993) -> (refnum out=w1988:refnum<file>, error out=w1987:errorcluster)  [unwired: 1 in, 1 out]
                          n1169 = Close File(refnum=w1988, error in=w1987) -> (error out=w1995:errorcluster)  [unwired: 1 out]
                          n1170 = call <vilib>:"Simple Error Handler.vi"("error in (no error)"=w1995) -> ()  [unwired: 1 in, 8 out]
                        }
                        frame #10 {
                          w2006 = "\t"
                          w2021 = i16 4 ("width (-)")
                          n1171 = local write "Z-50-N"(w2001) -> ()
                          n1172 = Wait (ms)(milliseconds to wait=u32 5000) -> ()  [unwired: 1 out]
                          n1173 = Open/Create/Replace File(file path (use dialog)=w2002, operation (0:open)=T2."open") -> (refnum out=w2015:refnum<file>, error out=w2014:errorcluster)  [unwired: 2 in, 3 out]
                          n1174 = Set File Position(refnum=w2015, from (0:start)=enum16{"start", "end", "current"}."end", error in=w2014) -> (refnum out=w2017:refnum<file>, error out=w2018:errorcluster)  [unwired: 1 in]
                          n1175 = call "RLC_read.vi"("Path"=w2003, "String"="cmd /c rlc_read_ZAN.py") -> ("MEASURE A"=w2000:dbl, "MEASURE V [V]"=w2005:dbl, "MEASURE B"=w1999:dbl, "MEASURE I [A]"=w2004:dbl)  [unwired: 2 out]
                          n1176 = Number To Engineering String(2:w2021, 4:w2004) -> (0:w2007:string)  [unwired: 2 in]
                          n1177 = local write "MEASURE A 10"(w2000) -> ()
                          n1178 = local write "MEASURE B 10"(w1999) -> ()
                          n1179 = Number To Engineering String(2:w2021, 4:w2005) -> (0:w2008:string)  [unwired: 2 in]
                          n1180 = Number To Engineering String(2:w2021, 4:w2000) -> (0:w2010:string)  [unwired: 2 in]
                          n1181 = Number To Engineering String(2:w2021, 4:w1999) -> (0:w2009:string)  [unwired: 2 in]
                          n1182 = Concatenate Strings(w2010, w2006, w2009, w2006, w2008, w2006, w2007, w2006) -> (w2011:string)
                          n1183 = Write to Text File(file (use dialog)=w2017, text=w2011, error in=w2018) -> (refnum out=w2013:refnum<file>, error out=w2012:errorcluster)  [unwired: 1 in, 1 out]
                          n1184 = Close File(refnum=w2013, error in=w2012) -> (error out=w2020:errorcluster)  [unwired: 1 out]
                          n1185 = call <vilib>:"Simple Error Handler.vi"("error in (no error)"=w2020) -> ()  [unwired: 1 in, 8 out]
                        }
                        frame #11 {
                          w2031 = "\t"
                          w2046 = i16 4 ("width (-)")
                          n1186 = Wait (ms)(milliseconds to wait=u32 5000) -> ()  [unwired: 1 out]
                          n1187 = local write "Z-100-L"(w2024) -> ()
                          n1188 = Open/Create/Replace File(file path (use dialog)=w2027, operation (0:open)=T2."open") -> (refnum out=w2040:refnum<file>, error out=w2039:errorcluster)  [unwired: 2 in, 3 out]
                          n1189 = Set File Position(refnum=w2040, from (0:start)=enum16{"start", "end", "current"}."end", error in=w2039) -> (refnum out=w2042:refnum<file>, error out=w2043:errorcluster)  [unwired: 1 in]
                          n1190 = call "RLC_read.vi"("Path"=w2028, "String"="cmd /c rlc_read_ZBL.py") -> ("MEASURE A"=w2026:dbl, "MEASURE V [V]"=w2030:dbl, "MEASURE B"=w2025:dbl, "MEASURE I [A]"=w2029:dbl)  [unwired: 2 out]
                          n1191 = Number To Engineering String(2:w2046, 4:w2029) -> (0:w2032:string)  [unwired: 2 in]
                          n1192 = local write "MEASURE A 11"(w2026) -> ()
                          n1193 = local write "MEASURE B 11"(w2025) -> ()
                          n1194 = Number To Engineering String(2:w2046, 4:w2030) -> (0:w2033:string)  [unwired: 2 in]
                          n1195 = Number To Engineering String(2:w2046, 4:w2026) -> (0:w2035:string)  [unwired: 2 in]
                          n1196 = Number To Engineering String(2:w2046, 4:w2025) -> (0:w2034:string)  [unwired: 2 in]
                          n1197 = Concatenate Strings(w2035, w2031, w2034, w2031, w2033, w2031, w2032, w2031) -> (w2036:string)
                          n1198 = Write to Text File(file (use dialog)=w2042, text=w2036, error in=w2043) -> (refnum out=w2038:refnum<file>, error out=w2037:errorcluster)  [unwired: 1 in, 1 out]
                          n1199 = Close File(refnum=w2038, error in=w2037) -> (error out=w2045:errorcluster)  [unwired: 1 out]
                          n1200 = call <vilib>:"Simple Error Handler.vi"("error in (no error)"=w2045) -> ()  [unwired: 1 in, 8 out]
                        }
                        frame #12 {
                          w2056 = "\t"
                          w2071 = i16 4 ("width (-)")
                          n1201 = Wait (ms)(milliseconds to wait=u32 5000) -> ()  [unwired: 1 out]
                          n1202 = local write "Z-100-N"(w2051) -> ()
                          n1203 = Open/Create/Replace File(file path (use dialog)=w2052, operation (0:open)=T2."open") -> (refnum out=w2065:refnum<file>, error out=w2064:errorcluster)  [unwired: 2 in, 3 out]
                          n1204 = Set File Position(refnum=w2065, from (0:start)=enum16{"start", "end", "current"}."end", error in=w2064) -> (refnum out=w2067:refnum<file>, error out=w2068:errorcluster)  [unwired: 1 in]
                          n1205 = call "RLC_read.vi"("Path"=w2053, "String"="cmd /c rlc_read_ZBN.py") -> ("MEASURE A"=w2050:dbl, "MEASURE V [V]"=w2055:dbl, "MEASURE B"=w2049:dbl, "MEASURE I [A]"=w2054:dbl)  [unwired: 2 out]
                          n1206 = Number To Engineering String(2:w2071, 4:w2054) -> (0:w2057:string)  [unwired: 2 in]
                          n1207 = local write "MEASURE A 12"(w2050) -> ()
                          n1208 = local write "MEASURE B 12"(w2049) -> ()
                          n1209 = Number To Engineering String(2:w2071, 4:w2055) -> (0:w2058:string)  [unwired: 2 in]
                          n1210 = Number To Engineering String(2:w2071, 4:w2050) -> (0:w2060:string)  [unwired: 2 in]
                          n1211 = Number To Engineering String(2:w2071, 4:w2049) -> (0:w2059:string)  [unwired: 2 in]
                          n1212 = Concatenate Strings(w2060, w2056, w2059, w2056, w2058, w2056, w2057, w2056) -> (w2061:string)
                          n1213 = Write to Text File(file (use dialog)=w2067, text=w2061, error in=w2068) -> (refnum out=w2063:refnum<file>, error out=w2062:errorcluster)  [unwired: 1 in, 1 out]
                          n1214 = Close File(refnum=w2063, error in=w2062) -> (error out=w2070:errorcluster)  [unwired: 1 out]
                          n1215 = call <vilib>:"Simple Error Handler.vi"("error in (no error)"=w2070) -> ()  [unwired: 1 in, 8 out]
                        }
                        frame #13 {
                          w2081 = "\t"
                          w2096 = i16 4 ("width (-)")
                          n1216 = local write "Z-1K-L"(w2076) -> ()
                          n1217 = Wait (ms)(milliseconds to wait=u32 5000) -> ()  [unwired: 1 out]
                          n1218 = Open/Create/Replace File(file path (use dialog)=w2077, operation (0:open)=T2."open") -> (refnum out=w2090:refnum<file>, error out=w2089:errorcluster)  [unwired: 2 in, 3 out]
                          n1219 = Set File Position(refnum=w2090, from (0:start)=enum16{"start", "end", "current"}."end", error in=w2089) -> (refnum out=w2092:refnum<file>, error out=w2093:errorcluster)  [unwired: 1 in]
                          n1220 = call "RLC_read.vi"("Path"=w2078, "String"="cmd /c rlc_read_ZCL.py") -> ("MEASURE A"=w2075:dbl, "MEASURE V [V]"=w2080:dbl, "MEASURE B"=w2074:dbl, "MEASURE I [A]"=w2079:dbl)  [unwired: 2 out]
                          n1221 = Number To Engineering String(2:w2096, 4:w2079) -> (0:w2082:string)  [unwired: 2 in]
                          n1222 = local write "MEASURE A 13"(w2075) -> ()
                          n1223 = local write "MEASURE B 13"(w2074) -> ()
                          n1224 = Number To Engineering String(2:w2096, 4:w2080) -> (0:w2083:string)  [unwired: 2 in]
                          n1225 = Number To Engineering String(2:w2096, 4:w2075) -> (0:w2085:string)  [unwired: 2 in]
                          n1226 = Number To Engineering String(2:w2096, 4:w2074) -> (0:w2084:string)  [unwired: 2 in]
                          n1227 = Concatenate Strings(w2085, w2081, w2084, w2081, w2083, w2081, w2082, w2081) -> (w2086:string)
                          n1228 = Write to Text File(file (use dialog)=w2092, text=w2086, error in=w2093) -> (refnum out=w2088:refnum<file>, error out=w2087:errorcluster)  [unwired: 1 in, 1 out]
                          n1229 = Close File(refnum=w2088, error in=w2087) -> (error out=w2095:errorcluster)  [unwired: 1 out]
                          n1230 = call <vilib>:"Simple Error Handler.vi"("error in (no error)"=w2095) -> ()  [unwired: 1 in, 8 out]
                        }
                        frame #14 {
                          w2106 = "\t"
                          w2121 = i16 4 ("width (-)")
                          n1231 = local write "Z-1K-N"(w2101) -> ()
                          n1232 = Wait (ms)(milliseconds to wait=u32 5000) -> ()  [unwired: 1 out]
                          n1233 = Open/Create/Replace File(file path (use dialog)=w2102, operation (0:open)=T2."open") -> (refnum out=w2115:refnum<file>, error out=w2114:errorcluster)  [unwired: 2 in, 3 out]
                          n1234 = Set File Position(refnum=w2115, from (0:start)=enum16{"start", "end", "current"}."end", error in=w2114) -> (refnum out=w2117:refnum<file>, error out=w2118:errorcluster)  [unwired: 1 in]
                          n1235 = call "RLC_read.vi"("Path"=w2103, "String"="cmd /c rlc_read_ZCN.py") -> ("MEASURE A"=w2100:dbl, "MEASURE V [V]"=w2105:dbl, "MEASURE B"=w2099:dbl, "MEASURE I [A]"=w2104:dbl)  [unwired: 2 out]
                          n1236 = Number To Engineering String(2:w2121, 4:w2104) -> (0:w2107:string)  [unwired: 2 in]
                          n1237 = local write "MEASURE A 14"(w2100) -> ()
                          n1238 = local write "MEASURE B 14"(w2099) -> ()
                          n1239 = Number To Engineering String(2:w2121, 4:w2105) -> (0:w2108:string)  [unwired: 2 in]
                          n1240 = Number To Engineering String(2:w2121, 4:w2100) -> (0:w2110:string)  [unwired: 2 in]
                          n1241 = Number To Engineering String(2:w2121, 4:w2099) -> (0:w2109:string)  [unwired: 2 in]
                          n1242 = Concatenate Strings(w2110, w2106, w2109, w2106, w2108, w2106, w2107, w2106) -> (w2111:string)
                          n1243 = Write to Text File(file (use dialog)=w2117, text=w2111, error in=w2118) -> (refnum out=w2113:refnum<file>, error out=w2112:errorcluster)  [unwired: 1 in, 1 out]
                          n1244 = Close File(refnum=w2113, error in=w2112) -> (error out=w2120:errorcluster)  [unwired: 1 out]
                          n1245 = call <vilib>:"Simple Error Handler.vi"("error in (no error)"=w2120) -> ()  [unwired: 1 in, 8 out]
                        }
                        frame #15 {
                          w2131 = "\t"
                          w2146 = i16 4 ("width (-)")
                          n1246 = Wait (ms)(milliseconds to wait=u32 5000) -> ()  [unwired: 1 out]
                          n1247 = local write "Z-10K-L"(w2124) -> ()
                          n1248 = Open/Create/Replace File(file path (use dialog)=w2127, operation (0:open)=T2."open") -> (refnum out=w2140:refnum<file>, error out=w2139:errorcluster)  [unwired: 2 in, 3 out]
                          n1249 = Set File Position(refnum=w2140, from (0:start)=enum16{"start", "end", "current"}."end", error in=w2139) -> (refnum out=w2142:refnum<file>, error out=w2143:errorcluster)  [unwired: 1 in]
                          n1250 = call "RLC_read.vi"("Path"=w2128, "String"="cmd /c rlc_read_ZDL.py") -> ("MEASURE A"=w2126:dbl, "MEASURE V [V]"=w2130:dbl, "MEASURE B"=w2125:dbl, "MEASURE I [A]"=w2129:dbl)  [unwired: 2 out]
                          n1251 = Number To Engineering String(2:w2146, 4:w2129) -> (0:w2132:string)  [unwired: 2 in]
                          n1252 = local write "MEASURE A 15"(w2126) -> ()
                          n1253 = local write "MEASURE B 15"(w2125) -> ()
                          n1254 = Number To Engineering String(2:w2146, 4:w2130) -> (0:w2133:string)  [unwired: 2 in]
                          n1255 = Number To Engineering String(2:w2146, 4:w2126) -> (0:w2135:string)  [unwired: 2 in]
                          n1256 = Number To Engineering String(2:w2146, 4:w2125) -> (0:w2134:string)  [unwired: 2 in]
                          n1257 = Concatenate Strings(w2135, w2131, w2134, w2131, w2133, w2131, w2132, w2131) -> (w2136:string)
                          n1258 = Write to Text File(file (use dialog)=w2142, text=w2136, error in=w2143) -> (refnum out=w2138:refnum<file>, error out=w2137:errorcluster)  [unwired: 1 in, 1 out]
                          n1259 = Close File(refnum=w2138, error in=w2137) -> (error out=w2145:errorcluster)  [unwired: 1 out]
                          n1260 = call <vilib>:"Simple Error Handler.vi"("error in (no error)"=w2145) -> ()  [unwired: 1 in, 8 out]
                        }
                        frame #16 {
                          w2157 = "\t"
                          w2172 = i16 4 ("width (-)")
                          n1261 = Wait (ms)(milliseconds to wait=u32 5000) -> ()  [unwired: 1 out]
                          n1262 = local write "Z-10K-N"(w2151) -> ()
                          n1263 = Open/Create/Replace File(file path (use dialog)=w2152, operation (0:open)=T2."open") -> (refnum out=w2166:refnum<file>, error out=w2165:errorcluster)  [unwired: 2 in, 3 out]
                          n1264 = Set File Position(refnum=w2166, from (0:start)=enum16{"start", "end", "current"}."end", error in=w2165) -> (refnum out=w2168:refnum<file>, error out=w2169:errorcluster)  [unwired: 1 in]
                          n1265 = call "RLC_read.vi"("Path"=w2153, "String"="cmd /c rlc_read_ZDN.py") -> ("MEASURE A"=w2150:dbl, "MEASURE V [V]"=w2156:dbl, "MEASURE B"=w2149:dbl, "MEASURE I [A]"=w2155:dbl)  [unwired: 2 out]
                          n1266 = Number To Engineering String(2:w2172, 4:w2155) -> (0:w2158:string)  [unwired: 2 in]
                          n1267 = local write "MEASURE A 16"(w2150) -> ()
                          n1268 = local write "MEASURE B 16"(w2149) -> ()
                          n1269 = Number To Engineering String(2:w2172, 4:w2156) -> (0:w2159:string)  [unwired: 2 in]
                          n1270 = Number To Engineering String(2:w2172, 4:w2150) -> (0:w2161:string)  [unwired: 2 in]
                          n1271 = Number To Engineering String(2:w2172, 4:w2149) -> (0:w2160:string)  [unwired: 2 in]
                          n1272 = Concatenate Strings(w2161, w2157, w2160, w2157, w2159, w2157, w2158, w2157, "\r\n") -> (w2162:string)
                          n1273 = Write to Text File(file (use dialog)=w2168, text=w2162, error in=w2169) -> (refnum out=w2164:refnum<file>, error out=w2163:errorcluster)  [unwired: 1 in, 1 out]
                          n1274 = Close File(refnum=w2164, error in=w2163) -> (error out=w2171:errorcluster)  [unwired: 1 out]
                          n1275 = call <vilib>:"Simple Error Handler.vi"("error in (no error)"=w2171) -> ()  [unwired: 1 in, 8 out]
                        }
                        frame #17 {
                          n1276 = local write "Z-50-N"(w2175) -> ()
                          n1277 = local write "Z-50-L"(w2175) -> ()
                          n1278 = local write "C-1K-N"(w2175) -> ()
                          n1279 = local write "C-50-N"(w2175) -> ()
                          n1280 = local write "C-50-L"(w2175) -> ()
                          n1281 = local write "Z-1K-N"(w2175) -> ()
                          n1282 = local write "C-1K-L"(w2175) -> ()
                          n1283 = local write "Z-1K-L"(w2175) -> ()
                          n1284 = local write "Z-100-L"(w2175) -> ()
                          n1285 = local write "C-10K-L"(w2175) -> ()
                          n1286 = local write "Z-10K-L"(w2175) -> ()
                          n1287 = local write "C-10K-N"(w2175) -> ()
                          n1288 = local write "Z-10K-N"(w2175) -> ()
                          n1289 = local write "C-100-N"(w2175) -> ()
                          n1290 = local write "C-100-L"(w2175) -> ()
                          n1291 = local write "Z-100-N"(w2175) -> ()
                        }
                      }
                    }
                    n1292 = call <vilib>:"Mean.vi"("X"=w1726) -> ("mean"=w1709:dbl)  [unwired: 1 out]
                    n1293 = call <vilib>:"Mean.vi"("X"=w1725) -> ("mean"=w1708:dbl)  [unwired: 1 out]
                    n1294 = call <vilib>:"Mean.vi"("X"=w1724) -> ("mean"=w1707:dbl)  [unwired: 1 out]
                    n1295 = call <vilib>:"Mean.vi"("X"=w1723) -> ("mean"=w1706:dbl)  [unwired: 1 out]
                    n1296 = call <vilib>:"Mean.vi"("X"=w1722) -> ("mean"=w1705:dbl)  [unwired: 1 out]
                    n1297 = call <vilib>:"Mean.vi"("X"=w1721) -> ("mean"=w1704:dbl)  [unwired: 1 out]
                    n1298 = call <vilib>:"Mean.vi"("X"=w1720) -> ("mean"=w1703:dbl)  [unwired: 1 out]
                    n1299 = call <vilib>:"Mean.vi"("X"=w1719) -> ("mean"=w1702:dbl)  [unwired: 1 out]
                    n1300 = call <vilib>:"Mean.vi"("X"=w1718) -> ("mean"=w1701:dbl)  [unwired: 1 out]
                    n1301 = call <vilib>:"Mean.vi"("X"=w1717) -> ("mean"=w1700:dbl)  [unwired: 1 out]
                    n1302 = call <vilib>:"Mean.vi"("X"=w1716) -> ("mean"=w1699:dbl)  [unwired: 1 out]
                    n1303 = call <vilib>:"Mean.vi"("X"=w1715) -> ("mean"=w1698:dbl)  [unwired: 1 out]
                    n1304 = call <vilib>:"Mean.vi"("X"=w1714) -> ("mean"=w1697:dbl)  [unwired: 1 out]
                    n1305 = call <vilib>:"Mean.vi"("X"=w1713) -> ("mean"=w1696:dbl)  [unwired: 1 out]
                    n1306 = call <vilib>:"Mean.vi"("X"=w1712) -> ("mean"=w1695:dbl)  [unwired: 1 out]
                    n1307 = call <vilib>:"Mean.vi"("X"=w1711) -> ("mean"=w1694:dbl)  [unwired: 1 out]
                    n1308 = local write "mean"(w1709) -> ()
                    n1309 = local write "mean 2"(w1708) -> ()
                    n1310 = local write "mean 3"(w1707) -> ()
                    n1311 = local write "mean 4"(w1706) -> ()
                    n1312 = local write "mean 5"(w1705) -> ()
                    n1313 = local write "mean 6"(w1704) -> ()
                    n1314 = local write "mean 7"(w1703) -> ()
                    n1315 = local write "mean 8"(w1702) -> ()
                    n1316 = local write "mean 9"(w1701) -> ()
                    n1317 = local write "mean 10"(w1700) -> ()
                    n1318 = local write "mean 11"(w1699) -> ()
                    n1319 = local write "mean 12"(w1698) -> ()
                    n1320 = local write "mean 13"(w1697) -> ()
                    n1321 = local write "mean 14"(w1696) -> ()
                    n1322 = local write "mean 15"(w1695) -> ()
                    n1323 = local write "mean 16"(w1694) -> ()
                  }
                }
              }
              frame #2 {
                n1324 = case shown="True" w2177 {
                  tunnel: w2194 -> [_ w2210]
                  tunnel: w2193 -> [_ w2209]
                  tunnel: w2192 -> [_ w2208]
                  tunnel: w2191 -> [_ w2207]
                  tunnel: w2190 -> [_ w2206]
                  tunnel: w2189 -> [_ w2205]
                  tunnel: w2188 -> [_ w2204]
                  tunnel: w2187 -> [_ w2203]
                  tunnel: w2186 -> [_ w2202]
                  tunnel: w2185 -> [_ w2201]
                  tunnel: w2184 -> [_ w2200]
                  tunnel: w2183 -> [_ w2199]
                  tunnel: w2182 -> [_ w2198]
                  tunnel: w2181 -> [_ w2197]
                  tunnel: w2180 -> [_ w2196]
                  tunnel: w2179 -> [_ w2195]
                  frame False {
                  }
                  frame True {
                    w2225 = "\t"
                    w2242 = i16 4 ("precision (6)")
                    n1325 = property on="SET" class="DigNum (strict)"() -> ("Value"=w2211:i32)  [unwired: 2 in, 2 out]
                    n1326 = Number To Engineering String(2:w2242, 4:w2210) -> (0:w2240:string)  [unwired: 2 in]
                    n1327 = Number To Engineering String(2:w2242, 4:w2209) -> (0:w2239:string)  [unwired: 2 in]
                    n1328 = Number To Engineering String(2:w2242, 4:w2208) -> (0:w2238:string)  [unwired: 2 in]
                    n1329 = Number To Engineering String(2:w2242, 4:w2207) -> (0:w2237:string)  [unwired: 2 in]
                    n1330 = Number To Engineering String(2:w2242, 4:w2206) -> (0:w2236:string)  [unwired: 2 in]
                    n1331 = Number To Engineering String(2:w2242, 4:w2205) -> (0:w2235:string)  [unwired: 2 in]
                    n1332 = Number To Engineering String(2:w2242, 4:w2204) -> (0:w2234:string)  [unwired: 2 in]
                    n1333 = Number To Engineering String(2:w2242, 4:w2203) -> (0:w2233:string)  [unwired: 2 in]
                    n1334 = Number To Engineering String(2:w2242, 4:w2202) -> (0:w2232:string)  [unwired: 2 in]
                    n1335 = Number To Engineering String(2:w2242, 4:w2201) -> (0:w2231:string)  [unwired: 2 in]
                    n1336 = Number To Engineering String(2:w2242, 4:w2195) -> (0:w2230:string)  [unwired: 2 in]
                    n1337 = Number To Engineering String(2:w2242, 4:w2200) -> (0:w2229:string)  [unwired: 2 in]
                    n1338 = Number To Engineering String(2:w2242, 4:w2199) -> (0:w2228:string)  [unwired: 2 in]
                    n1339 = Number To Engineering String(2:w2242, 4:w2198) -> (0:w2227:string)  [unwired: 2 in]
                    n1340 = Number To Engineering String(2:w2242, 4:w2197) -> (0:w2226:string)  [unwired: 2 in]
                    n1341 = Number To Engineering String(2:w2242, 4:w2196) -> (0:w2224:string)  [unwired: 2 in]
                    n1342 = Number To Decimal String(number=w2211) -> (decimal integer string=w2241:string)  [unwired: 1 in]
                    n1343 = property on="path RLC_mean" class="Path"() -> ("Value"=w2212:path)  [unwired: 2 in, 2 out]
                    n1344 = Open/Create/Replace File(file path (use dialog)=w2212, operation (0:open)=T2."open") -> (refnum out=w2217:refnum<file>, error out=w2216:errorcluster)  [unwired: 2 in, 3 out]
                    n1345 = Concatenate Strings(w2241, w2225, w2240, w2225, w2239, w2225, w2238, w2225, w2237, w2225, w2236, w2225, w2235, w2225, w2234, w2225, w2233, w2225, w2232, w2225, w2231, w2225, w2230, w2225, w2229, w2225, w2228, w2225, w2227, w2225, w2226, w2225, w2224, "\r\n") -> (w2213:string)
                    n1346 = Set File Position(refnum=w2217, from (0:start)=enum16{"start", "end", "current"}."end", error in=w2216) -> (refnum out=w2219:refnum<file>, error out=w2220:errorcluster)  [unwired: 1 in]
                    n1347 = Write to Text File(file (use dialog)=w2219, text=w2213, error in=w2220) -> (refnum out=w2215:refnum<file>, error out=w2214:errorcluster)  [unwired: 1 in, 1 out]
                    n1348 = Close File(refnum=w2215, error in=w2214) -> (error out=w2222:errorcluster)  [unwired: 1 out]
                    n1349 = call <vilib>:"Simple Error Handler.vi"("error in (no error)"=w2222) -> ()  [unwired: 1 in, 8 out]
                  }
                }
              }
            }
            n1350 = local write "graph RLC"(w1649) -> ()
          }
        }
        n1351 = call <vilib>:"Linear Fit.vi"("Y"=w1622, "X"=w1626) -> ("Best Linear Fit"=w1624:dbl[], "slope"=→"bar/N":dbl)  [unwired: 9 in, 3 out]
        n1352 = Bundle(w1626, w1622) -> (w1629:cluster{i32[], dbl[]})  [unwired: 1 in]
        n1353 = call <vilib>:"General Polynomial Fit.vi"("Y"=w1631, "polynomial order"=w1647, "X"=w1626) -> ("Best Polynomial Fit"=w1643:dbl[], "Polynomial Coefficients"=w1644:dbl[])  [unwired: 9 in, 2 out]
        "Polynomial Coefficients 2" <- w1644
        n1354 = call <vilib>:"General Polynomial Fit.vi"("Y"=w1622, "polynomial order"=w1647, "X"=w1640) -> ("Best Polynomial Fit"=w1625:dbl[], "Polynomial Coefficients"=w1638:dbl[])  [unwired: 9 in, 2 out]
        "Polynomial Coefficients" <- w1638
        n1355 = Bundle(w1626, "Best Polynomial Fit"=w1625) -> (w1628:cluster{i32[], "Best Polynomial Fit":dbl[]})  [unwired: 1 in]
        n1356 = Build Array(w1631, w1643) -> (→"Linear Model Graph 2":dbl[][])
        n1357 = Index Array(array=w1638, index=0) -> (element=→"p fit":dbl)
        n1358 = Index Array(array=w1644, index=0) -> (element=→"T fit":dbl)
        n1359 = Build Array(w1622, w1625, w1624) -> (→"Linear Model Graph":dbl[][])
        n1360 = Bundle(w1626, "Best Linear Fit"=w1624) -> (w1627:cluster{i32[], "Best Linear Fit":dbl[]})  [unwired: 1 in]
        n1361 = Build Array(w1629, w1628, w1627) -> ()  [unwired: 1 out]
      }
    }
    n1362 = case shown="True" "Ligar RLC" {
      tunnel: w42 -> [_ w167]
      frame False {
      }
      frame True {
        w175 = "\t"
        w196 = "\t"
        w179 = "\r"
        w172 = "\r\n"
        w212 = "\r"
        w202 = "\t"
        n1363 = Strip Path(path=w167) -> (stripped path=w168:path, name=w171:string)
        n1364 = Get Date/Time String(date format (0)=enum16{"short", "long", "abbreviated"}."short", want seconds? (F)=TRUE) -> (date string=w219:string, time string=w218:string)  [unwired: 1 in]
        n1365 = Concatenate Strings("SET" ("Nota 4"), w175, "DATE" ("Nota 4"), w175, "TIME" ("Nota 4"), w175, w196, "P (BAR)" ("Nota 4"), w196, "T (ºC)" ("Nota 4"), w196, "C-50-L" ("Nota 4"), w196, "C-50-N" ("Nota 4"), w196, "C-100-L" ("Nota 4"), w196, "C-100-N" ("Nota 4"), w196, "C-1K-L" ("Nota 4"), w196, "C-1K-N" ("Nota 4"), w196, "C-10K-L" ("Nota 4"), w196, "C-10K-N" ("Nota 4"), w196, "Z-50-L" ("Nota 4"), w196, "Z-50-N" ("Nota 4"), w196, "Z-100-L" ("Nota 4"), w196, "Z-100-N" ("Nota 4"), w196, "Z-1K-L" ("Nota 4"), w196, "Z-1K-N" ("Nota 4"), w196, "Z-10K-L" ("Nota 4"), w196, "Z-10K-N" ("Nota 4")) -> (w180:string)
        n1366 = Concatenate Strings(w219, w202, w218) -> (w214:string)
        n1367 = Concatenate Strings(w171, "_RLC_CDH completo" ("string")) -> (w169:string)
        n1368 = Concatenate Strings("Sievert RLC - CDH:" ("string"), w202, w172, w172) -> (w200:string)
        n1369 = Concatenate Strings("Data Table" ("string"), w179, "==========" ("string"), w179, w180, w179) -> (w213:string)
        n1370 = File Dialog(6:".txt" ("pattern label"), 9:w169, 11:w168) -> (0:w210:errorcluster, 3:w211:path)  [unwired: 2 in, 4 out]
        n1371 = Open/Create/Replace File(file path (use dialog)=w211, error in=w210, operation (0:open)=T2."replace or create with confirmation", access (0:read/write)=enum16{"read/write", "read-only", "write-only"}."read/write") -> (refnum out=w207:refnum<file>, error out=w206:errorcluster)  [unwired: 3 out]
        n1372 = Concatenate Strings(w214, w212, w212, w200, w212, w212, "Nota 01: MEDIDAS COM RLC 300 - MULTILEITURA" ("Nota 4"), w212, w212, w213) -> (w217:string)
        n1373 = Write to Text File(file (use dialog)=w207, text=w217, error in=w206) -> (refnum out=w205:refnum<file>, error out=w203:errorcluster)  [unwired: 1 in, 1 out]
        n1374 = Close File(refnum=w205, error in=w203) -> (path=w199:path)  [unwired: 1 out]
        n1375 = local write "path RLC_completo"(w199) -> ()
      }
    }
    n1376 = case shown="True" "Ligar RLC" {
      tunnel: w42 -> [_ w110]
      frame False {
      }
      frame True {
        w119 = "\t"
        w140 = "\t"
        w123 = "\r"
        w116 = "\r\n"
        w155 = "\r"
        w145 = "\t"
        n1377 = Strip Path(path=w110) -> (stripped path=w112:path, name=w115:string)
        n1378 = Get Date/Time String(date format (0)=enum16{"short", "long", "abbreviated"}."short", want seconds? (F)=TRUE) -> (date string=w162:string, time string=w161:string)  [unwired: 1 in]
        n1379 = Concatenate Strings("SET" ("Nota 4"), w119, "DATE" ("Nota 4"), w119, "TIME" ("Nota 4"), w119, w140, "P (BAR)" ("Nota 4"), w140, "T (ºC)" ("Nota 4"), w140, "C-50-L" ("Nota 4"), w140, "C-50-N" ("Nota 4"), w140, "C-100-L" ("Nota 4"), w140, "C-100-N" ("Nota 4"), w140, "C-1K-L" ("Nota 4"), w140, "C-1K-N" ("Nota 4"), w140, "C-10K-L" ("Nota 4"), w140, "C-10K-N" ("Nota 4"), w140, "Z-50-L" ("Nota 4"), w140, "Z-50-N" ("Nota 4"), w140, "Z-100-L" ("Nota 4"), w140, "Z-100-N" ("Nota 4"), w140, "Z-1K-L" ("Nota 4"), w140, "Z-1K-N" ("Nota 4"), w140, "Z-10K-L" ("Nota 4"), w140, "Z-10K-N" ("Nota 4")) -> (w124:string)
        n1380 = Concatenate Strings(w162, w145, w161) -> (w157:string)
        n1381 = Concatenate Strings(w115, "_RLC_CDH mean" ("string")) -> (w113:string)
        n1382 = Concatenate Strings("Sievert RLC - CDH:" ("string"), w145, w116, w116) -> (w143:string)
        n1383 = Concatenate Strings("Data Table" ("string"), w123, "==========" ("string"), w123, w124, w123) -> (w156:string)
        n1384 = File Dialog(6:".txt" ("pattern label"), 9:w113, 11:w112) -> (0:w153:errorcluster, 3:w154:path)  [unwired: 2 in, 4 out]
        n1385 = Open/Create/Replace File(file path (use dialog)=w154, error in=w153, operation (0:open)=T2."replace or create with confirmation", access (0:read/write)=enum16{"read/write", "read-only", "write-only"}."read/write") -> (refnum out=w150:refnum<file>, error out=w149:errorcluster)  [unwired: 3 out]
        n1386 = Concatenate Strings(w157, w155, w155, w143, w155, w155, "Nota 01: MEDIDAS COM RLC 300 - MULTILEITURA" ("Nota 4"), w155, w155, w156) -> (w160:string)
        n1387 = Write to Text File(file (use dialog)=w150, text=w160, error in=w149) -> (refnum out=w148:refnum<file>, error out=w146:errorcluster)  [unwired: 1 in, 1 out]
        n1388 = Close File(refnum=w148, error in=w146) -> (path=w111:path)  [unwired: 1 out]
        n1389 = local write "path RLC_mean"(w111) -> ()
      }
    }
    n1390 = case shown="False" "Auto Ctrl" {
      tunnel: [TRUE ("Auto Ctrl") FALSE ("Auto Ctrl")] -> w48
      frame False {
      }
      frame True {
      }
    }
    n1391 = Exclusive Or(1:w45, 2:"stop") -> (0:w47:bool)
    n1392 = case shown="True" "RLC on/off" {
      tunnel: w35 -> [_ w53]
      frame False {
      }
      frame True {
        n1393 = call "RLC READ DINAMICO.vi"("Boolean"="graph RLC", "Path"=w53, "String"="Combo Box") -> ("MEASURE R [Ohm ]"=w57:dbl, "MEASURE C [F ]"=w56:dbl)  [unwired: 7 in]
        "MEASURE C [F ]" <- w56
        n1394 = Merge Signals(w56, w57) -> (→"Waveform Chart":dynamicdata)
        "String 4" <- "Combo Box"
      }
    }
    n1395 = case shown="True" "Open Button" {
      frame False {
      }
      frame True {
        n1396 = flat-sequence {
          tunnel: ["Sample name"] -> w1605
          tunnel: ["Nota"] -> w1604
          tunnel: [w1607] -> w1603
          tunnel: w1605 -> [w1620]
          tunnel: w1604 -> [w1619]
          tunnel: w1603 -> [w1614]
          frame #0 {
            n1397 = local write "Count SET"(0 ("Count SET")) -> ()
            n1398 = local write "Set atual"(0 ("Count  3")) -> ()
            n1399 = call "File_data_new.vi"("Nota 01"="Nota", "Sample name"="Sample name", "File name"="File name") -> ("path"=w1607:path)  [unwired: 8 in]
            "path" <- w1607
          }
          frame #1 {
            w1615 = FALSE
            n1400 = Strip Path(path=w1614) -> (stripped path=w1613:path, name=w1612:string)
            n1401 = local write "Pf2"(w1615) -> ()
            n1402 = local write "ZPit"(w1615) -> ()
            n1403 = local write "Pit"(w1615) -> ()
            n1404 = local write "ZPf2"(w1615) -> ()
            n1405 = local write "T"(w1615) -> ()
            n1406 = Concatenate Strings(w1612, "_cinetica" ("string")) -> (w1617:string)
            n1407 = call "File_data_cinetica.vi"("path in"=w1613, "Nota 01"=w1619, "Sample name"=w1620, "File name"=w1617) -> ("path"=→"path 2_cinetica":path)  [unwired: 7 in]
          }
        }
      }
    }
    n1408 = case shown="True" "Close RLC 2" {
      tunnel: w35 -> [_ w165]
      frame False {
      }
      frame True {
        n1409 = call "RLC_close.vi"("Path"=w165) -> ("String"=w166:string)  [unwired: 10 in]
        n1410 = local write "RLC300 - digimess"(w166) -> ()
      }
    }
    n1411 = case shown="True" "Open Button 2" {
      frame False {
      }
      frame True {
        n1412 = property on="Sample name" class="Str"() -> ("Value"=w1601:string)  [unwired: 2 in, 2 out]
        n1413 = property on="File name" class="Str"() -> ("Value"=w1602:string)  [unwired: 2 in, 2 out]
        n1414 = property on="Nota" class="Str"() -> ("Value"=w1600:string)  [unwired: 2 in, 2 out]
        n1415 = call "Open file.vi"("Nota 01"=w1600, "Sample name"=w1601, "File name"=w1602) -> ("path open old"=w1599:path)  [unwired: 8 in]
        n1416 = local write "path"(w1599) -> ()
      }
    }
    n1417 = case shown="True" "Refresh Button 2" {
      frame False {
      }
      frame True {
        n1418 = property on="Waveform Chart" class="WFChart (strict)"("History Data"=dynamicdata[] []) -> ()  [unwired: 2 in, 2 out]
      }
    }
    n1419 = local write "Manual Ctrl"(w48) -> ()
    n1420 = Or(x=w38, y=w37) -> (x .or. y?=w39:bool)
    n1421 = Or(x=w39, y="Refresh Button") -> (x .or. y?=w41:bool)
    n1422 = case shown="True" w41 {
      frame False {
      }
      frame True {
        n1423 = stacked-sequence {
          frame #0 {
            n1424 = property on="Waveform Chart P 2" class="WFChart (strict)"("History Data"=dbl[][] []) -> ()  [unwired: 2 in, 2 out]
          }
          frame #1 {
            n1425 = property on="path RLC_mean" class="Path"() -> ("Value"=w71:path)  [unwired: 2 in, 2 out]
            n1426 = Open/Create/Replace File(file path (use dialog)=w71, operation (0:open)=T2."open", access (0:read/write)=enum16{"read/write", "read-only", "write-only"}."read-only") -> (refnum out=w75:refnum<file>, error out=w74:errorcluster)  [unwired: 3 in, 1 out]
            n1427 = Read from Text File(file (use dialog)=w75, error in=w74) -> (refnum out=w80:refnum<file>, text=w76:string, error out=w79:errorcluster)  [unwired: 2 in, 1 out]
            n1428 = Close File(refnum=w80, error in=w79) -> ()  [unwired: 2 out]
            n1429 = Search/Split String(string=w76, search string/char (-)="SET\tDATE\tTIME\t\tP (BAR)\tT (ºC)\tC-50-L\tC-50-N\tC-100-L\tC-100-N\tC-1K-L\tC-1K-N\tC-10K-L\tC-10K-N\tZ-50-L\tZ-50-N\tZ-100-L\tZ-100-N\tZ-1K-L\tZ-1K-N\tZ-10K-L\tZ-10K-N") -> (match + rest of string=w81:string)  [unwired: 1 in, 2 out]
            n1430 = String Subset(string=w81, offset (0)=150) -> (substring=w88:string)  [unwired: 1 in]
            n1431 = Spreadsheet String To Array(format string="%#g", spreadsheet string=w88) -> (array=w87:dbl[][])  [unwired: 2 in]
            n1432 = Transpose Matrix(1:w87) -> (0:w101:dbl[][])
            n1433 = Index Array(array=w101, index (row)=1 ("index (row) 4")) -> (element=w102:dbl[])  [unwired: 1 in]
            n1434 = Index Array(array=w101, index (row)=2 ("index (row) 5")) -> (element=w103:dbl[])  [unwired: 1 in]
            n1435 = Index Array(array=w101, index (row)=3 ("index (row) 2")) -> (element=w104:dbl[])  [unwired: 1 in]
            n1436 = Index Array(array=w101, index (row)=4 ("index (row) 3")) -> (element=w105:dbl[])  [unwired: 1 in]
            n1437 = Index Array(array=w101, index (row)=5 ("index (row) 4")) -> (element=w106:dbl[])  [unwired: 1 in]
            n1438 = Index Array(array=w101, index (row)=6 ("index (row) 5")) -> (element=w107:dbl[])  [unwired: 1 in]
            n1439 = Index Array(array=w101, index (row)=7 ("index (row) 2")) -> (element=w108:dbl[])  [unwired: 1 in]
            n1440 = Index Array(array=w101, index (row)=8 ("index (row) 3")) -> (element=w109:dbl[])  [unwired: 1 in]
            n1441 = Index Array(array=w101, index (row)=9 ("index (row) 4")) -> (element=w70:dbl[])  [unwired: 1 in]
            n1442 = Index Array(array=w101, index (row)=10 ("index (row) 5")) -> (element=w69:dbl[])  [unwired: 1 in]
            n1443 = Index Array(array=w101, index (row)=11 ("index (row) 2")) -> (element=w68:dbl[])  [unwired: 1 in]
            n1444 = Index Array(array=w101, index (row)=12 ("index (row) 3")) -> (element=w67:dbl[])  [unwired: 1 in]
            n1445 = Index Array(array=w101, index (row)=13 ("index (row) 4")) -> (element=w66:dbl[])  [unwired: 1 in]
            n1446 = Index Array(array=w101, index (row)=14 ("index (row) 5")) -> (element=w65:dbl[])  [unwired: 1 in]
            n1447 = Index Array(array=w101, index (row)=15 ("index (row) 2")) -> (element=w64:dbl[])  [unwired: 1 in]
            n1448 = Index Array(array=w101, index (row)=16 ("index (row) 3")) -> (element=w63:dbl[])  [unwired: 1 in]
            n1449 = Build Array(w102, w103, w104, w105, w106, w107, w108, w109, w70, w69, w68, w67, w66, w65, w64, w63) -> (w62:dbl[][])
            n1450 = Transpose Matrix(1:w62) -> (0:→"Waveform Chart P 2":dbl[][])
          }
        }
      }
    }
  }
  n1451 = local write "path 2_cinetica"(path "C:/H2_Painel/painel_auto/cinetica.txt" ("path")) -> ()
  n1452 = local write "path RLC_completo"(path "C:/H2_Painel/painel_auto/RLC_full.txt" ("path RLC_mean")) -> ()
  n1453 = local write "path RLC_mean"(path "C:/H2_Painel/painel_auto/RLC_mean.txt" ("path RLC_mean")) -> ()
  n1454 = local write "path"(path "C:/H2_Painel/painel_auto/Arquivo_Padrao.txt" ("path")) -> ()
  n1455 = local write "Array"(dbl[] [0.5, 1.0, 2.0, 3.0, 4.0, 5.0, 6.0, 7.0, 8.0, 9.0, 10.0, 11.0, 12.0, 13.0, 14.0, 15.0, 16.0, 17.0, 18.0, 19.0, 20.0, 30.0, 40.0, 50.0, 60.0, 70.0] ("Array")) -> ()
